vi "Run_old02.vi"(8 "error in (no error)":errorcluster, 11 "Channel in":refnum<class "Channel.lvclass">) -> (0 "error out":errorcluster, 3 "Channel out":refnum<class "Channel.lvclass">)   [LabVIEW 2018, in "Channel.lvclass"]
uses:
  Channel.lvclass
  C:/Users/devstaff/sparc4/s4gui/Versao ZeroMQ REQ-REP/SPARC4_GUI -20241009_20240802/Device/Device.lvclass
  Channel.lvclass/Channel.ctl
  Interface/Interface.lvclass/Interface.ctl
  Device/Device.lvclass/Device.ctl
  StateMachine/State Machine.lvclass
  Interface/Interface.lvclass
  Device/Device.lvclass
panel:
  out "resp RESUME":string
  out "resp PAUSE":string
  out "x = y?":T1
  out "resp ABORT":string
  out "resp STOP":string
  out "resposta do STATUS":string
  out "resp INIT":string
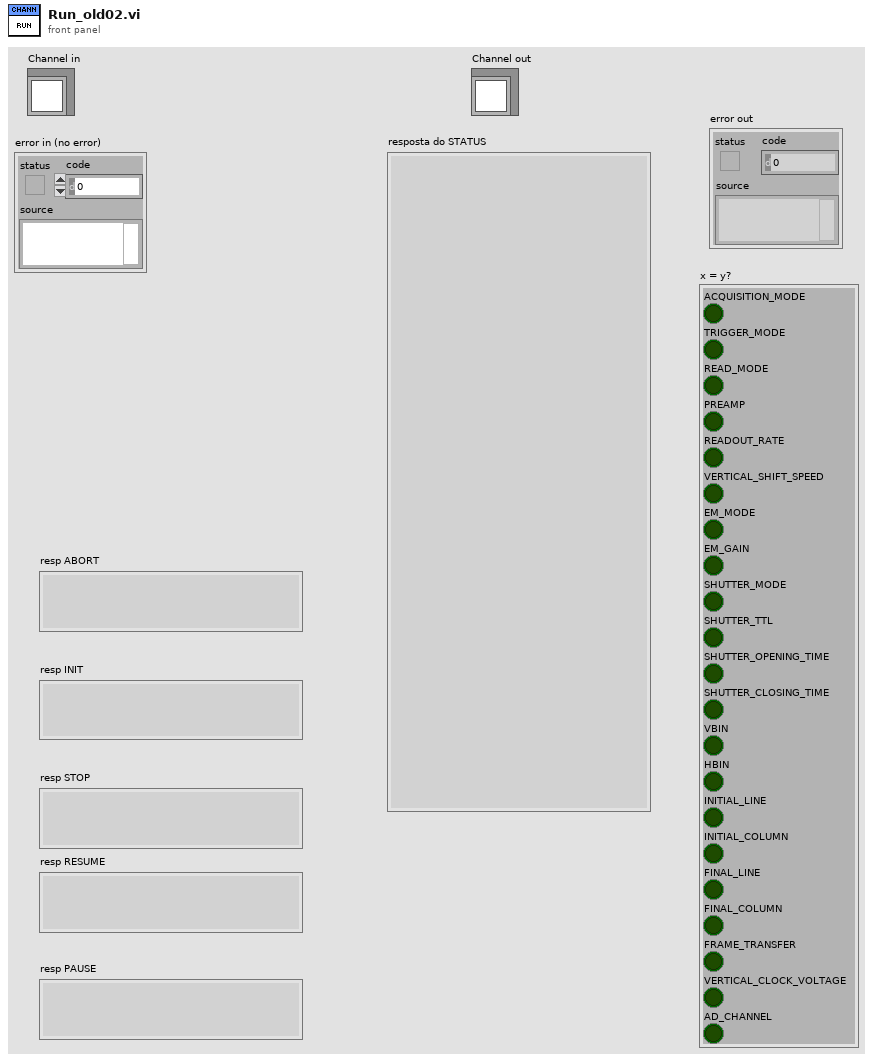
[diagram p1: front panel]
types:
  T1 = cluster{"ACQUISITION_MODE":bool, "TRIGGER_MODE":bool, "READ_MODE":bool, "PREAMP":bool, "READOUT_RATE":bool, "VERTICAL_SHIFT_SPEED":bool, "EM_MODE":bool, "EM_GAIN":bool, "SHUTTER_MODE":bool, "SHUTTER_TTL":bool, "SHUTTER_OPENING_TIME":bool, "SHUTTER_CLOSING_TIME":bool, "VBIN":bool, "HBIN":bool, "INITIAL_LINE":bool, "INITIAL_COLUMN":bool, "FINAL_LINE":bool, "FINAL_COLUMN":bool, "FRAME_TRANSFER":bool, "VERTICAL_CLOCK_VOLTAGE":bool, "AD_CHANNEL":bool}
  T2 = cluster{"TEMP":dbl, "EXPTIME":dbl, "#FRAMES":u32, "#CYCLES":u32, "#SEQS":u32, "WAVEPLATE_POS":u32, "COOLER_POWER_STATUS":dbl, "suffix":string}
  T3 = cluster{"ACQUISITION_MODE":u8, "TRIGGER_MODE":u8, "READ_MODE":u8, "PREAMP":u8, "READOUT_RATE":u8, "VERTICAL_SHIFT_SPEED":u8, "EM_MODE":u8, "EM_GAIN":u16, "SHUTTER_MODE":u8, "SHUTTER_TTL":u8, "SHUTTER_OPENING_TIME":u16, "SHUTTER_CLOSING_TIME":u16, "VBIN":u16, "HBIN":u16, "INITIAL_LINE":u16, "INITIAL_COLUMN":u16, "FINAL_LINE":u16, "FINAL_COLUMN":u16, "FRAME_TRANSFER":bool, "VERTICAL_CLOCK_VOLTAGE":u8, "AD_CHANNEL":u32}
  T4 = cluster{"Image Name":string, "Image Path":string, "#FRAMES":u32, "EXPTIME":dbl, "PREAMP":u8, "READOUT_RATE":u8, "VERTICAL_SHIFT_SPEED":u8, "ACQUISITION_MODE":u8, "READ_MODE":u8, "EM_MODE":u8, "EM_GAIN":u16, "SHUTTER_MODE":u8, "SHUTTER_TTL":u8, "SHUTTER_OPENNING_TIME":u16, "SHUTTER_CLOSING_TIME":u16, "VBIN":u16, "HBIN":u16, "INITIAL_LINE":u16, "INITIAL_COLUMN":u16, "FINAL_LINE":u16, "FINAL_COLUMN":u16, "Cooler ON/OFF":u16, "Set temperature":i8, "Exposições realizadas":u16, "Kinetic Serie Length":u32, "Number of Accumulations":u32, "Kinetic Cycle Time":u32, "FRAME_TRANSFER":bool, "VERTICAL_CLOCK_VOLTAGE":u8, "TRIGGER_MODE":u8, "Number of exp":u32, "AD_CHANNEL":u32}
  T5 = cluster{"OBSERVER":string, "OBJECT":string, "CTRLINTE":string, "PROJID":string, "SYNCMODE":string, "INSTMODE":string, "FILTER":string, "OBSTYPE":string, "CHANNEL 1":bool, "CHANNEL 2":bool, "CHANNEL 3":bool, "CHANNEL 4":bool, "TCSMODE":bool, "COMMENT":string, "broker":string, "GUIVRSN":string, "timestamp":string}
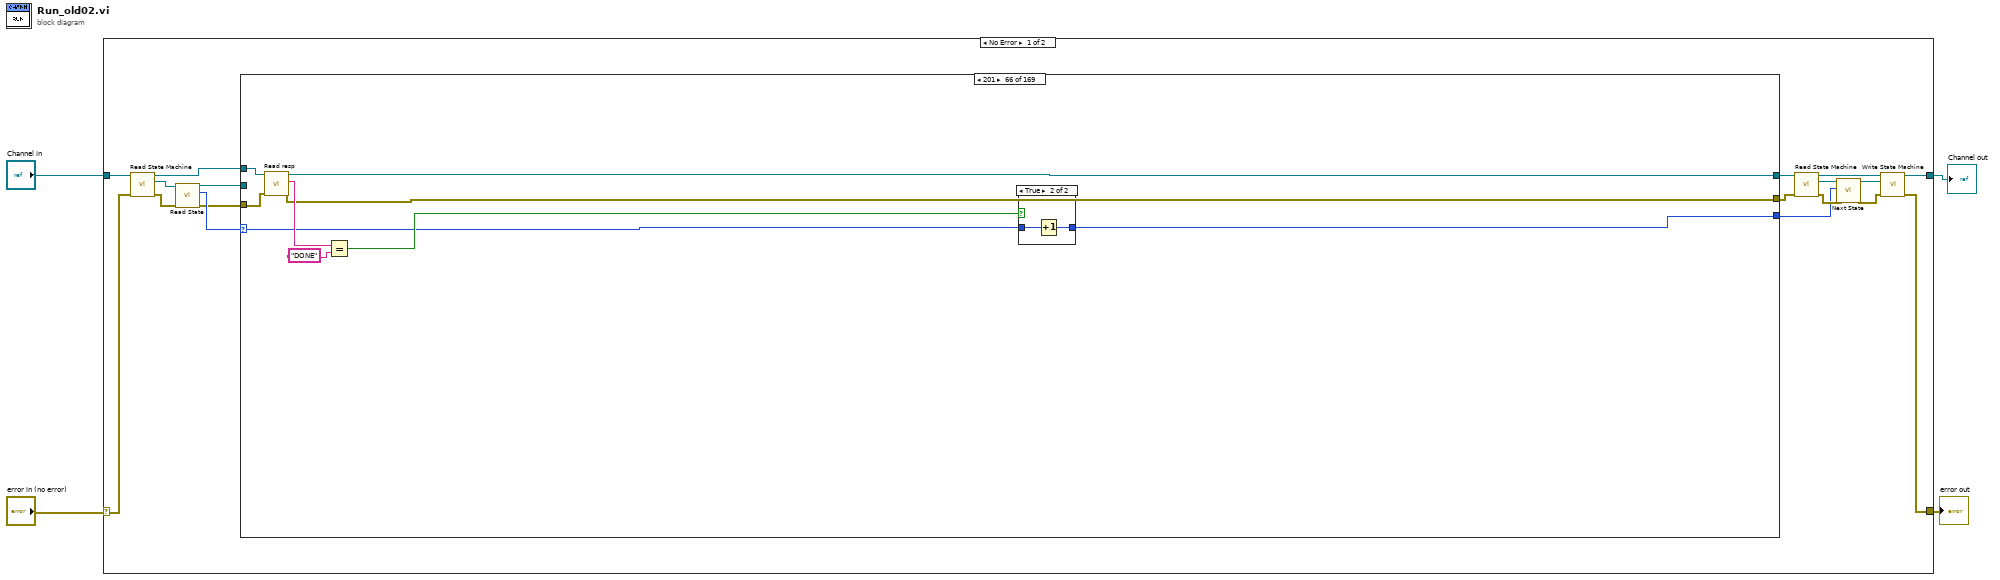
[diagram p0: block diagram]
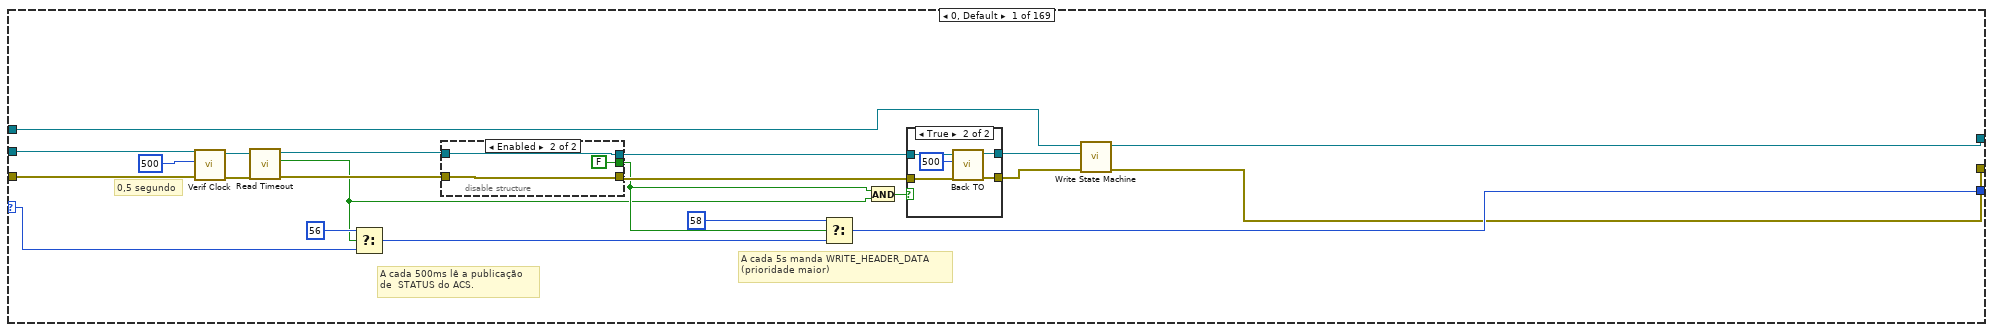
[diagram p2: hidden frame]
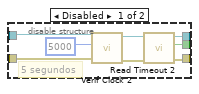
[diagram p3: hidden frame]
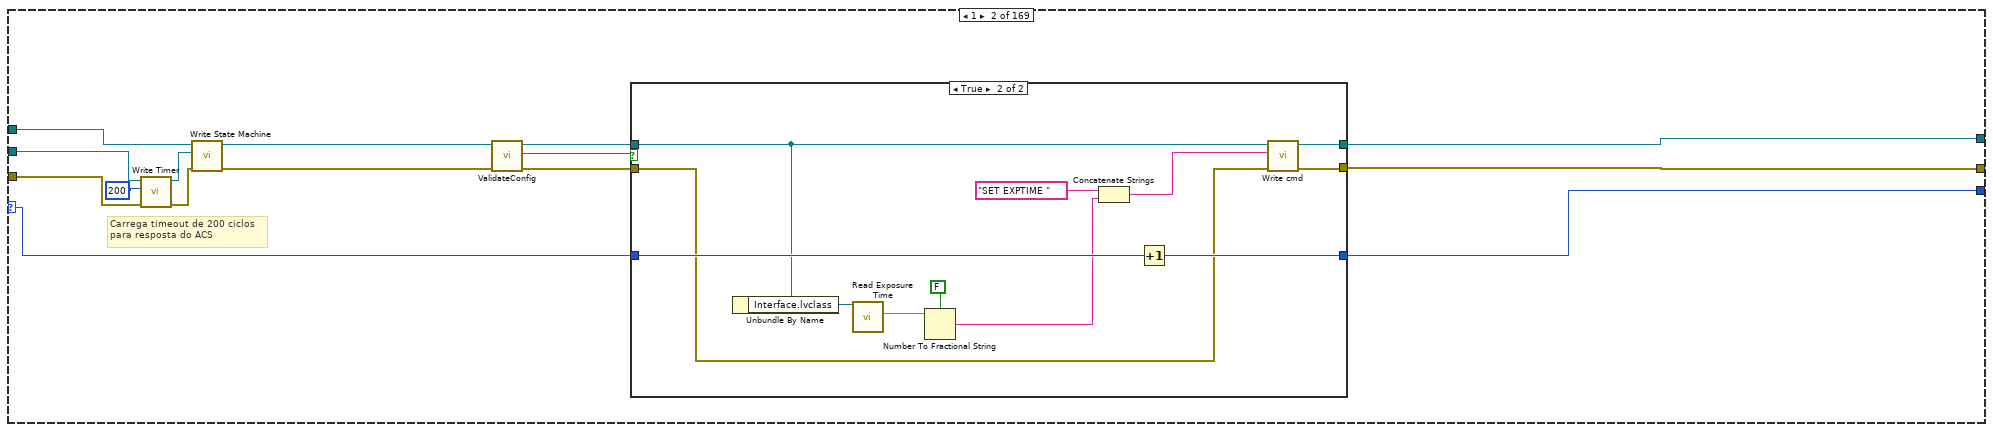
[diagram p5: hidden frame]
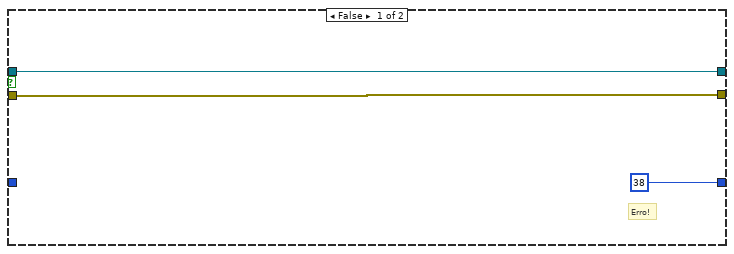
[diagram p6: hidden frame]
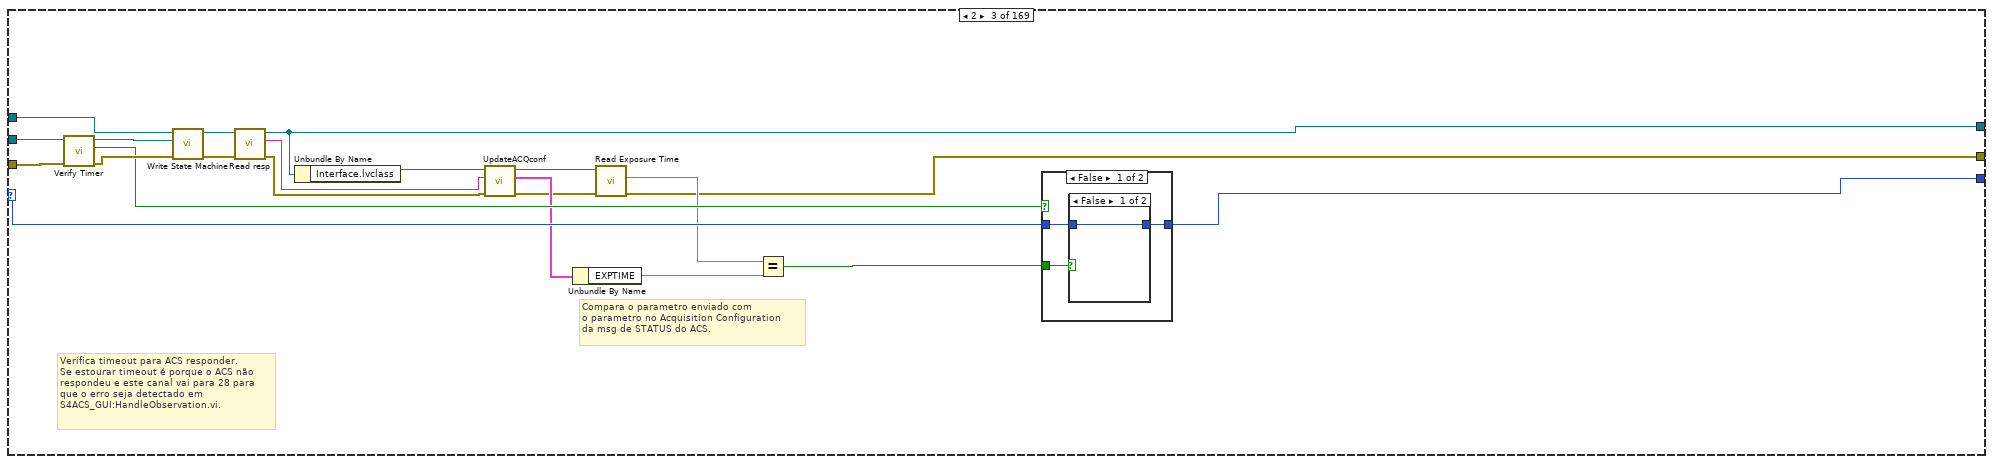
[diagram p7: hidden frame]
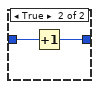
[diagram p8: hidden frame]
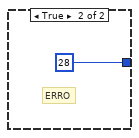
[diagram p9: hidden frame]
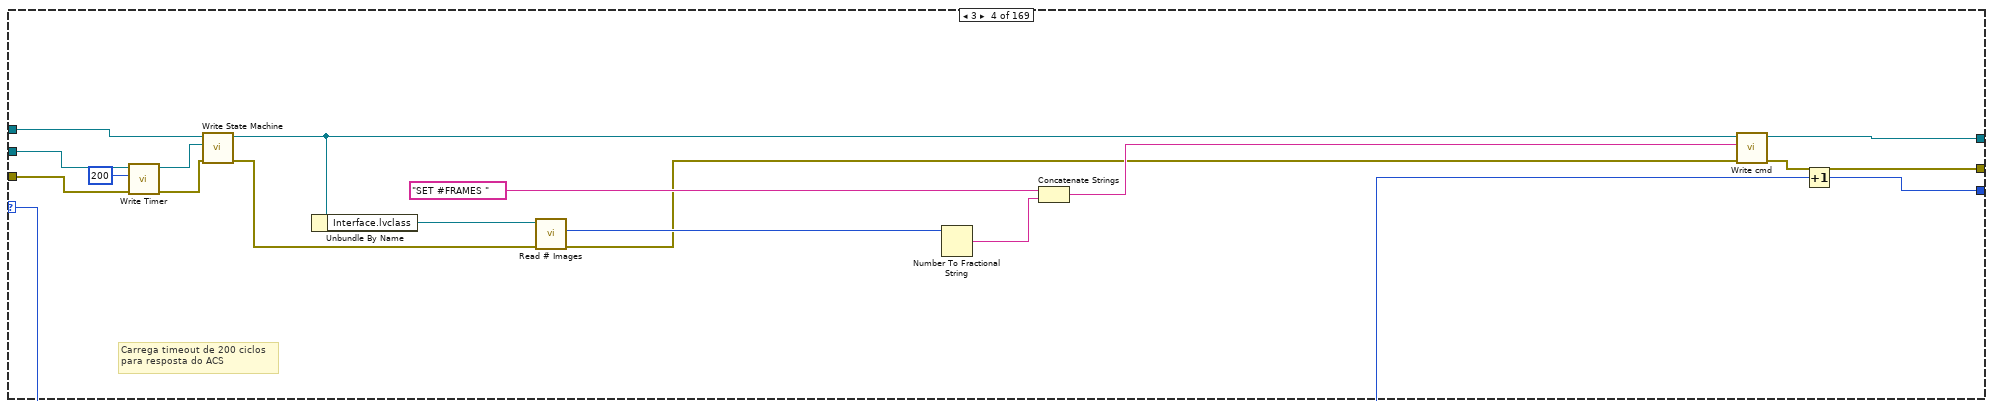
[diagram p10: hidden frame]
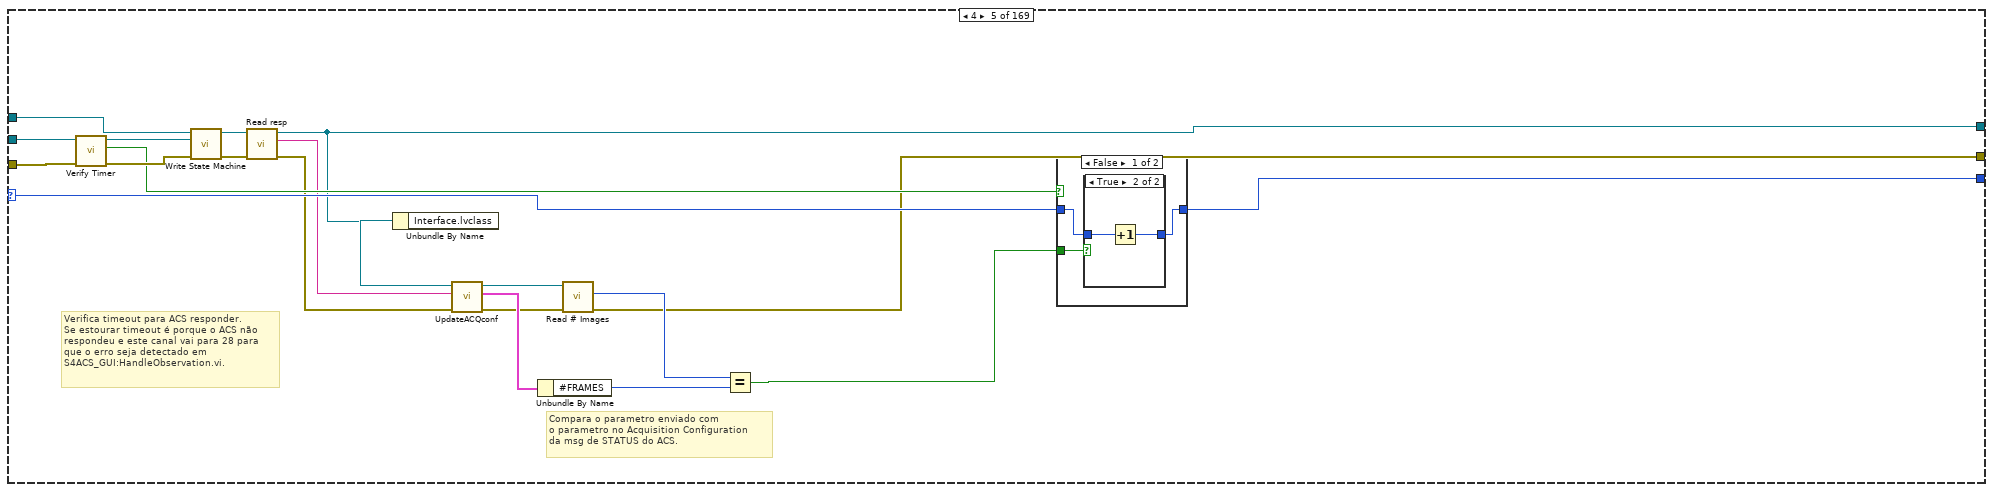
[diagram p11: hidden frame]
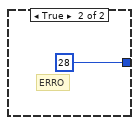
[diagram p13: hidden frame]
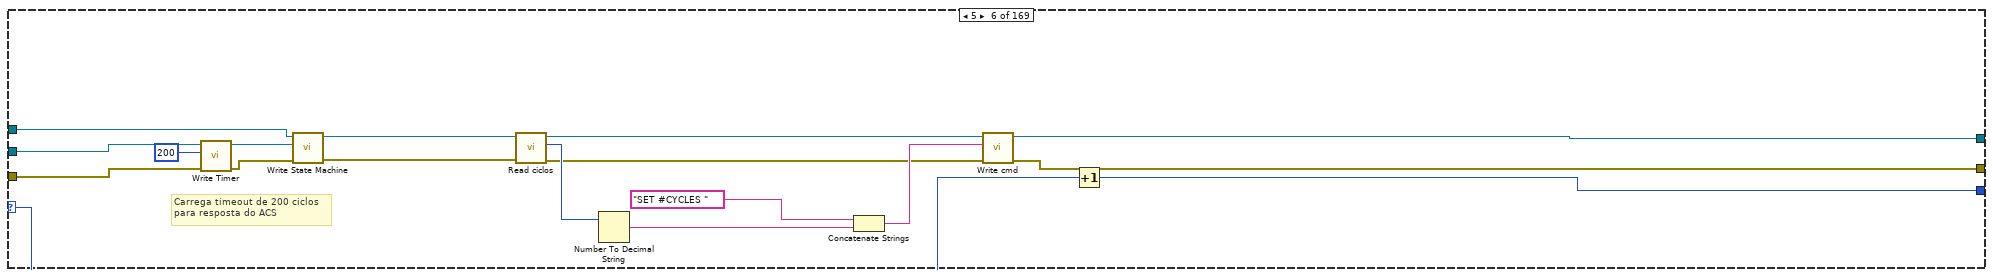
[diagram p14: hidden frame]
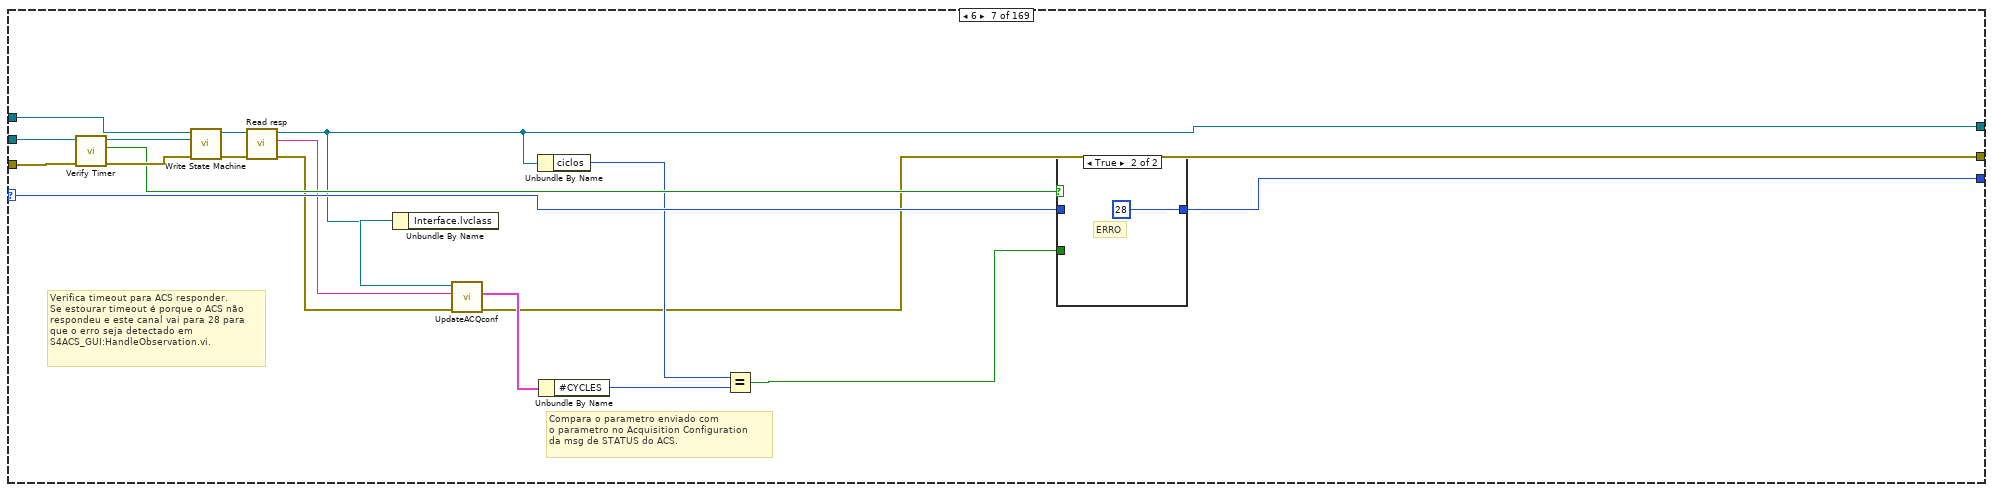
[diagram p15: hidden frame]
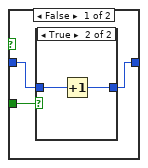
[diagram p16: hidden frame]
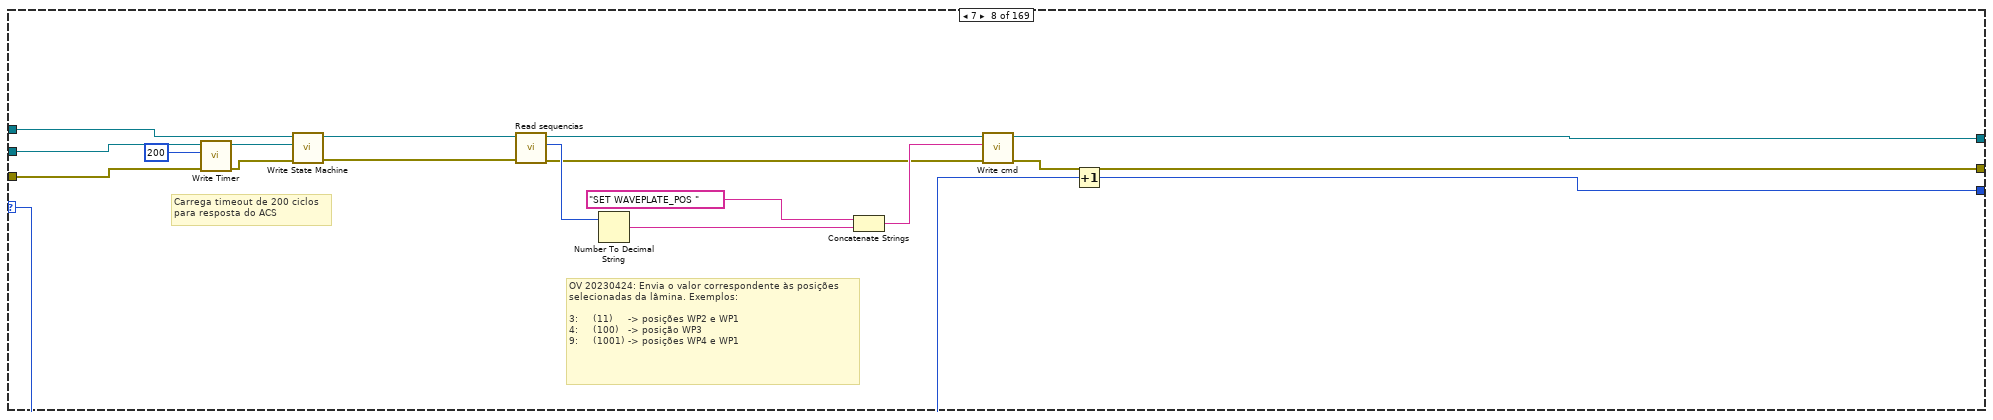
[diagram p18: hidden frame]
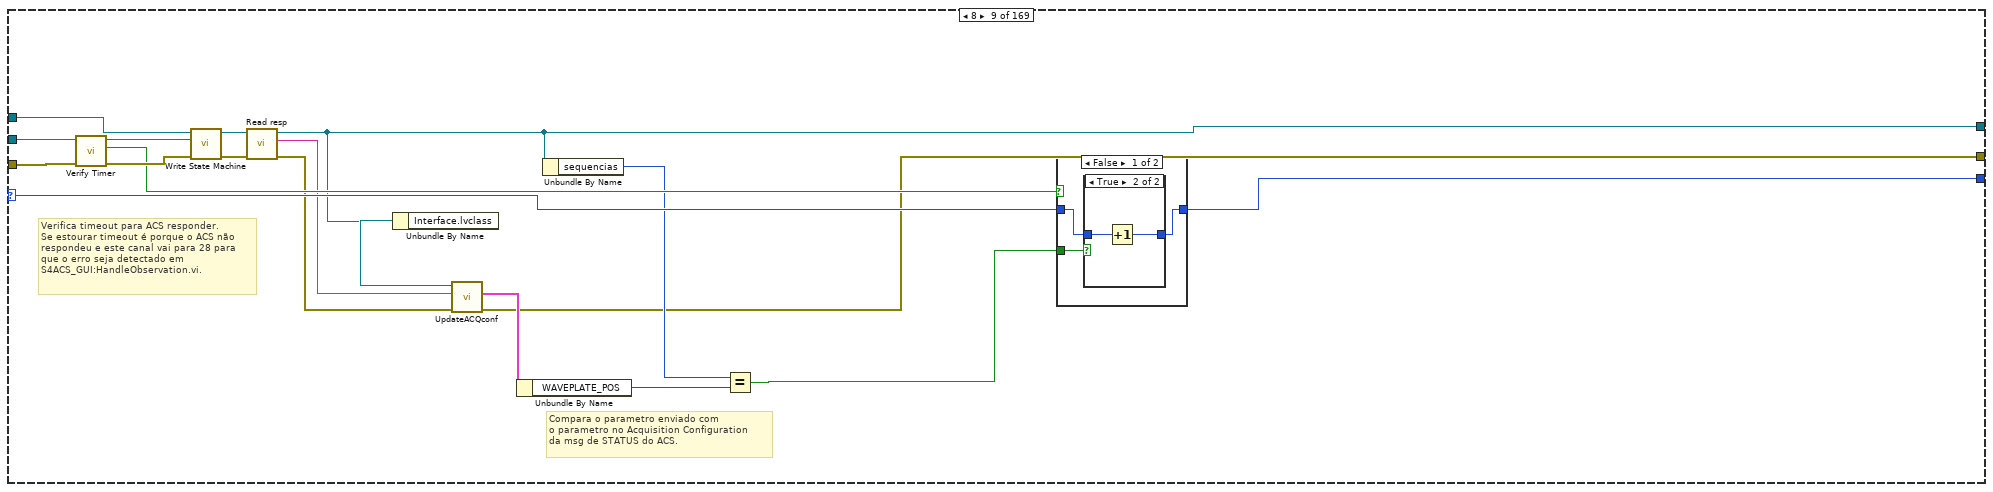
[diagram p19: hidden frame]
diagram:
  n1 = case shown="No Error" "error in (no error)" {
    selector: "error in (no error)" -> [w21 w2905]
    tunnel: [w6 w2905] -> w3
    tunnel: [w11 w2904] -> w1
    tunnel: "Channel in" -> [w22 w2904]
    frame No Error {
      n2 = call-dynamic "Read State Machine.vi"("error in (no error)"=w21, "Device in"=w22) -> ("error out"=w18:errorcluster, "State Machine.lvclass"=w20:refnum<class "State Machine.lvclass">, "Device out"=w16:refnum<class "Channel.lvclass">)  [unwired: 7 in]
      n3 = call-dynamic "Read State.vi"("error in (no error)"=w18, "State Machine in"=w20) -> ("error out"=w17:errorcluster, "State"=w19:i32, "State Machine out"=w5:refnum<class "State Machine.lvclass">)  [unwired: 7 in]
      n4 = case shown="201" w19 {
        selector: w19 -> [w40 w74 w106 w123 w151 w175 w195 w219 w239 w263 w292 w306 w318 w348 w362 w387 w390 w396 w412 w440 w459 w472 w516 w545 _ w568 _ w605 w634 w645 w706 w726 w804 w863 w931 _ _ w1036 w1068 w1089 w1127 w1140 w1156 w1219 w1253 w1286 w1292 w1306 w1314 w1329 _ w1354 _ w1373 w1384 w1404 w1424 w1444 w1464 w1484 w1504 w1524 w1544 _ w1564 w1572 w1585 w1598 w1614 w1622 w1635 w1649 w1661 w1669 w1682 w1695 w1707 w1715 w1728 w1741 w1753 w1761 w1774 w1787 w1799 w1807 w1820 w1833 w1845 w1853 w1866 w1879 w1891 w1899 w1912 w1925 w1937 w1945 w1958 w1971 w1987 w1995 w2008 w2021 w2033 w2041 w2054 w2067 w2079 w2087 w2100 w2113 w2125 w2133 w2146 w2159 w2171 w2179 w2192 w2205 w2217 w2225 w2238 w2251 w2263 w2271 w2284 w2297 w2309 w2317 w2330 w2343 w2355 w2363 w2376 w2389 w2401 w2409 w2422 w2435 w2447 w2455 w2468 w2481 w2497 w2505 w2518 w2531 w2543 w2553 w2566 w2579 w2593 w2601 w2614 w2627 w2645 w2678 w2699 w2721 w2734 w2763 w2769 w2795 w2807 w2832 w2844 w2869 w2881]
        tunnel: w17 -> [w38 w73 w110 w125 w154 w177 w198 w221 w242 w260 w291 w308 w320 w350 w364 w389 w392 w394 w404 w439 w454 w466 w514 w544 w561 w570 w582 w602 w627 w643 w667 w723 w768 w856 w905 w965 w1004 w1044 w1056 w1085 w1122 w1134 w1170 w1216 w1248 w1279 w1296 w1309 w1318 w1331 w1345 w1356 w1370 w1377 w1388 w1399 w1419 w1439 w1459 w1479 w1499 w1519 w1539 w1557 w1570 w1579 w1589 w1601 w1620 w1629 w1639 w1652 w1667 w1676 w1686 w1698 w1713 w1722 w1732 w1744 w1759 w1768 w1778 w1790 w1805 w1814 w1824 w1836 w1851 w1860 w1870 w1882 w1897 w1906 w1916 w1928 w1943 w1952 w1962 w1974 w1993 w2002 w2012 w2024 w2039 w2048 w2058 w2070 w2085 w2094 w2104 w2116 w2131 w2140 w2150 w2162 w2177 w2186 w2196 w2208 w2223 w2232 w2242 w2254 w2269 w2278 w2288 w2300 w2315 w2324 w2334 w2346 w2361 w2370 w2380 w2392 w2407 w2416 w2426 w2438 w2453 w2462 w2472 w2484 w2503 w2512 w2522 w2534 w2549 w2560 w2570 w2582 w2599 w2608 w2618 w2630 w2637 w2682 w2706 w2715 w2740 w2757 w2775 w2797 w2809 w2834 w2846 w2871 w2883]
        tunnel: [w23 w76 w93 w137 w139 w183 w185 w227 w229 w271 w274 w314 w327 w356 w371 w389 w392 w394 w416 w420 w461 w474 w524 w527 w566 w570 w586 w597 w621 w647 w698 w711 w779 w851 w906 w977 w1015 w1043 w1069 w1090 w1119 w1142 w1157 w1221 w1235 w1267 w1293 w1302 w1315 w1326 w1343 w1351 w1365 w1376 w1385 w1399 w1419 w1439 w1459 w1479 w1499 w1519 w1539 w1557 w1569 w1573 w1588 w1599 w1619 w1623 w1638 w1650 w1666 w1670 w1685 w1696 w1712 w1716 w1731 w1742 w1758 w1762 w1777 w1788 w1804 w1808 w1823 w1834 w1850 w1854 w1869 w1880 w1896 w1900 w1915 w1926 w1942 w1946 w1961 w1972 w1992 w1996 w2011 w2022 w2038 w2042 w2057 w2068 w2084 w2088 w2103 w2114 w2130 w2134 w2149 w2160 w2176 w2180 w2195 w2206 w2222 w2226 w2241 w2252 w2268 w2272 w2287 w2298 w2314 w2318 w2333 w2344 w2360 w2364 w2379 w2390 w2406 w2410 w2425 w2436 w2452 w2456 w2471 w2482 w2502 w2506 w2521 w2532 w2548 w2554 w2569 w2580 w2598 w2602 w2617 w2628 w2649 w2664 w2702 w2724 w2743 w2765 w2778 w2803 w2816 w2840 w2853 w2877 w2890] -> w7
        tunnel: w16 -> [w31 w71 w113 w126 w158 w178 w202 w222 w246 w259 w290 w309 w324 w351 w368 w388 w391 w393 w407 w438 w456 w469 w513 w543 w564 w569 w583 w596 w633 w644 w680 w719 w778 w858 w899 w976 w1014 w1038 w1060 w1083 w1123 w1135 w1171 w1215 w1251 w1280 w1297 w1308 w1319 w1323 w1346 w1348 w1371 w1375 w1389 w1397 w1417 w1437 w1457 w1477 w1497 w1517 w1537 w1559 w1568 w1580 w1587 w1602 w1618 w1630 w1637 w1653 w1665 w1677 w1684 w1699 w1711 w1723 w1730 w1745 w1757 w1769 w1776 w1791 w1803 w1815 w1822 w1837 w1849 w1861 w1868 w1883 w1895 w1907 w1914 w1929 w1941 w1953 w1960 w1975 w1991 w2003 w2010 w2025 w2037 w2049 w2056 w2071 w2083 w2095 w2102 w2117 w2129 w2141 w2148 w2163 w2175 w2187 w2194 w2209 w2221 w2233 w2240 w2255 w2267 w2279 w2286 w2301 w2313 w2325 w2332 w2347 w2359 w2371 w2378 w2393 w2405 w2417 w2424 w2439 w2451 w2463 w2470 w2485 w2501 w2513 w2520 w2535 w2547 w2561 w2568 w2583 w2597 w2609 w2616 w2631 w2639 w2685 w2705 w2717 w2741 w2759 w2776 w2798 w2813 w2835 w2850 w2872 w2887]
        tunnel: [w30 w77 w102 w138 w142 w184 w187 w228 w231 w264 w276 w315 w328 w357 w372 w388 w391 w393 w417 w421 w462 w477 w517 w529 w567 w569 w571 w598 w622 w648 w705 w712 w803 w852 w930 w978 w1016 w1045 w1070 w1091 w1120 w1143 w1167 w1222 w1233 w1273 w1294 w1301 w1316 w1325 w1344 w1350 w1369 w1378 w1381 w1401 w1421 w1441 w1461 w1481 w1501 w1521 w1541 w1559 w1571 w1574 w1590 w1597 w1621 w1624 w1640 w1648 w1668 w1671 w1687 w1694 w1714 w1717 w1733 w1740 w1760 w1763 w1779 w1786 w1806 w1809 w1825 w1832 w1852 w1855 w1871 w1878 w1898 w1901 w1917 w1924 w1944 w1947 w1963 w1970 w1994 w1997 w2013 w2020 w2040 w2043 w2059 w2066 w2086 w2089 w2105 w2112 w2132 w2135 w2151 w2158 w2178 w2181 w2197 w2204 w2224 w2227 w2243 w2250 w2270 w2273 w2289 w2296 w2316 w2319 w2335 w2342 w2362 w2365 w2381 w2388 w2408 w2411 w2427 w2434 w2454 w2457 w2473 w2480 w2504 w2507 w2523 w2530 w2550 w2555 w2571 w2578 w2600 w2603 w2619 w2626 w2650 w2675 w2701 w2725 w2744 w2766 w2779 w2804 w2817 w2841 w2854 w2878 w2891] -> w14
        tunnel: [w37 w75 w105 w132 w150 w182 w194 w226 w238 w265 w293 w313 w319 w355 w360 w387 w390 w397 w413 w441 w460 w473 w518 w546 31 ("State") w568 0 ("State") w603 w635 w646 w707 w727 w805 w864 w932 0 ("State") 54 ("State") w1035 w1071 w1088 w1128 w1141 w1155 w1220 w1254 w1287 w1295 w1307 w1317 w1330 0 ("State") w1355 0 ("State") w1374 w1386 w1396 w1416 w1436 w1456 w1476 w1496 w1516 w1536 u8 0 ("State") w1565 w1575 w1586 w1600 w1615 w1625 w1636 w1651 w1662 w1672 w1683 w1697 w1708 w1718 w1729 w1743 w1754 w1764 w1775 w1789 w1800 w1810 w1821 w1835 w1846 w1856 w1867 w1881 w1892 w1902 w1913 w1927 w1938 w1948 w1959 w1973 w1988 w1998 w2009 w2023 w2034 w2044 w2055 w2069 w2080 w2090 w2101 w2115 w2126 w2136 w2147 w2161 w2172 w2182 w2193 w2207 w2218 w2228 w2239 w2253 w2264 w2274 w2285 w2299 w2310 w2320 w2331 w2345 w2356 w2366 w2377 w2391 w2402 w2412 w2423 w2437 w2448 w2458 w2469 w2483 w2498 w2508 w2519 w2533 w2544 w2556 w2567 w2581 w2594 w2604 w2615 w2629 w2646 w2677 w2700 w2722 w2732 w2764 w2767 w2802 w2808 w2839 w2845 w2876 w2879] -> w8
        tunnel: w5 -> [w39 w72 w112 w127 w159 w176 w203 w220 w247 w261 w288 w307 w321 w349 w365 _ _ _ w406 w436 w455 w470 w512 w541 w563 _ w584 w601 w631 _ w670 w724 w771 w860 w904 w966 w1005 w1040 w1061 w1086 w1124 w1137 w1172 w1217 w1252 w1281 _ _ _ _ _ _ _ _ _ _ _ _ _ _ _ _ _ _ _ _ _ _ _ _ _ _ _ _ _ _ _ _ _ _ _ _ _ _ _ _ _ _ _ _ _ _ _ _ _ _ _ _ _ _ _ _ _ _ _ _ _ _ _ _ _ _ _ _ _ _ _ _ _ _ _ _ _ _ _ _ _ _ _ _ _ _ _ _ _ _ _ _ _ _ _ _ _ _ _ _ _ _ _ _ _ _ _ _ _ _ w2641 w2684 w2707 w2713 w2738 w2756 w2773 w2796 w2810 w2833 w2847 w2870 w2884]
        frame 0, Default {
          # "A cada 5s manda WRITE_HEADER_DATA\n(prioridade maior)"
          # "A cada 500ms lê a publicação \nde  STATUS do ACS."
          # "0,5 segundo"
          n5 = call-dynamic "Verif Clock.vi"("error in (no error)"=w38, "period (ms)"=u32 500 ("period"), "State Machine in"=w39) -> ("error out"=w43:errorcluster, "State Machine out"=w42:refnum<class "State Machine.lvclass">)  [unwired: 6 in, 1 out]
          n6 = call-dynamic "Read Timeout.vi"("error in (no error)"=w43, "State Machine in"=w42) -> ("error out"=w33:errorcluster, "Timeout"=w24:bool, "State Machine out"=w34:refnum<class "State Machine.lvclass">)  [unwired: 7 in]
          n7 = Select(t=56 ("State"), s=w24, f=w40) -> (s? t:f=w35:i32)
          n8 = disable-structure shown="Enabled" {
            disable-tunnel: w34 -> [w52 w54]
            disable-tunnel: w33 -> [w50 w53]
            disable-tunnel: [w47 w53] -> w32
            disable-tunnel: [w46 w54] -> w28
            disable-tunnel: [w45 FALSE ("Timeout 2")] -> w25
            frame Disabled {
              # "5 segundos"
              n9 = call-dynamic "Verif Clock 2.vi"("error in (no error)"=w50, "period (ms)"=u32 5000 ("period"), "State Machine in"=w52) -> ("error out"=w49:errorcluster, "State Machine out"=w51:refnum<class "State Machine.lvclass">)  [unwired: 6 in, 1 out]
              n10 = call-dynamic "Read Timeout 2.vi"("error in (no error)"=w49, "State Machine in"=w51) -> ("error out"=w47:errorcluster, "Timeout 2"=w45:bool, "State Machine out"=w46:refnum<class "State Machine.lvclass">)  [unwired: 7 in]
            }
            frame Enabled {
            }
          }
          n11 = Select(t=58 ("f"), s=w25, f=w35) -> (s? t:f=w37:i32)
          n12 = And(x=w25, y=w24) -> (x .and. y?=w26:bool)
          n13 = case shown="True" w26 {
            tunnel: w32 -> [w56 w62]
            tunnel: [w56 w61] -> w29
            tunnel: w28 -> [w57 w60]
            tunnel: [w57 w59] -> w27
            frame False {
            }
            frame True {
              n14 = call-dynamic "Back TO.vi"("error in (no error)"=w62, "time back (ms)"=u32 500 ("time(ms)"), "State Machine in"=w60) -> ("error out"=w61:errorcluster, "State Machine out"=w59:refnum<class "State Machine.lvclass">)  [unwired: 7 in]
            }
          }
          n15 = call-dynamic "Write State Machine.vi"("error in (no error)"=w29, "State Machine.lvclass"=w27, "Device in"=w31) -> ("error out"=w23:errorcluster, "Device out"=w30:refnum<class "Channel.lvclass">)  [unwired: 7 in]
        }
        frame 1 {
          # "Carrega timeout de 200 ciclos\npara resposta do ACS"
          n16 = call-dynamic "Write Timer.vi"("error in (no error)"=w73, "Timer"=u32 200, "State Machine in"=w72) -> ("error out"=w68:errorcluster, "State Machine out"=w70:refnum<class "State Machine.lvclass">)  [unwired: 7 in]
          n17 = call-dynamic "Write State Machine.vi"("error in (no error)"=w68, "State Machine.lvclass"=w70, "Device in"=w71) -> ("error out"=w66:errorcluster, "Device out"=w67:refnum<class "Channel.lvclass">)  [unwired: 7 in]
          n18 = call-dynamic "ValidateConfig.vi"("error in (no error)"=w66, "Channel in"=w67) -> ("error out"=w64:errorcluster, "valid?"=w63:bool, "Channel out"=w65:refnum<class "Channel.lvclass">)  [unwired: 7 in]
          n19 = case shown="True" w63 {
            tunnel: [w80 w92] -> w77
            tunnel: [w79 w91] -> w76
            tunnel: [38 w90] -> w75
            tunnel: w74 -> [_ w89]
            tunnel: w65 -> [w80 w82]
            tunnel: w64 -> [w79 w81]
            frame False {
              # "Erro!"
            }
            frame True {
              n20 = Unbundle By Name(w82) -> ("Interface.lvclass"=w88:refnum<class "Interface.lvclass">)
              n21 = call "Read Exposure Time.vi"("Interface in"=w88) -> ("Exposure Time"=w87:dbl)  [unwired: 8 in, 2 out]
              n22 = Number To Fractional String(use system decimal point (T)=FALSE, number=w87) -> (F-format string=w86:string)  [unwired: 2 in]
              n23 = Concatenate Strings("SET EXPTIME " ("cmd"), w86) -> (w85:string)
              n24 = Increment(x=w89) -> (x+1=w90:i32)
              n25 = call-dynamic "Write cmd.vi"("error in (no error)"=w81, "cmd"=w85, "Device in"=w82) -> ("error out"=w91:errorcluster, "Device out"=w92:refnum<class "Channel.lvclass">)  [unwired: 7 in]
            }
          }
        }
        frame 2 {
          # "Compara o parametro enviado com\no parametro no Acquisition Configuration\nda msg de STATUS do ACS."
          # "Verifica timeout para ACS responder.\nSe estourar timeout é porque o ACS não \nrespondeu e este canal vai para 28 para \nque o erro seja detectado em\nS4ACS_GUI:HandleObservation.vi."
          n26 = call "Verify Timer.vi"("error in (no error)"=w110, "State Machine in"=w112) -> ("error out"=w109:errorcluster, "timeout"=w107:bool, "State Machine out"=w111:refnum<class "State Machine.lvclass">)  [unwired: 7 in]
          n27 = call-dynamic "Write State Machine.vi"("error in (no error)"=w109, "State Machine.lvclass"=w111, "Device in"=w113) -> ("error out"=w108:errorcluster, "Device out"=w104:refnum<class "Channel.lvclass">)  [unwired: 7 in]
          n28 = call-dynamic "Read resp.vi"("error in (no error)"=w108, "Device in"=w104) -> ("error out"=w95:errorcluster, "resp"=w103:string, "Device out"=w102:refnum<class "Channel.lvclass">)  [unwired: 7 in]
          n29 = Unbundle By Name(w102) -> ("Interface.lvclass"=w101:refnum<class "Interface.lvclass">)
          n30 = call-dynamic "UpdateACQconf.vi"("error in (no error)"=w95, "status"=w103, "Interface in"=w101) -> ("error out"=w94:errorcluster, "ACQ conf rx"=w99:T2, "Interface out"=w100:refnum<class "Interface.lvclass">)  [unwired: 6 in]
          n31 = Unbundle By Name(w99) -> ("EXPTIME"=w97:dbl)
          n32 = call "Read Exposure Time.vi"("error in (no error)"=w94, "Interface in"=w100) -> ("error out"=w93:errorcluster, "Exposure Time"=w98:dbl)  [unwired: 7 in, 1 out]
          n33 = Equal?(x=w98, y=w97) -> (x = y?=w96:bool)
          n34 = case shown="False" w107 {
            tunnel: [w115 28] -> w105
            tunnel: w106 -> [w116 _]
            tunnel: w96 -> [w114 _]
            frame False {
              n35 = case shown="False" w114 {
                tunnel: [w117 w118] -> w115
                tunnel: w116 -> [w117 w119]
                frame False {
                }
                frame True {
                  n36 = Increment(x=w119) -> (x+1=w118:i32)
                }
              }
            }
            frame True {
              # "ERRO"
            }
          }
        }
        frame 3 {
          # "Carrega timeout de 200 ciclos\npara resposta do ACS"
          n37 = call-dynamic "Write Timer.vi"("error in (no error)"=w125, "Timer"=u32 200, "State Machine in"=w127) -> ("error out"=w128:errorcluster, "State Machine out"=w130:refnum<class "State Machine.lvclass">)  [unwired: 7 in]
          n38 = call-dynamic "Write State Machine.vi"("error in (no error)"=w128, "State Machine.lvclass"=w130, "Device in"=w126) -> ("error out"=w122:errorcluster, "Device out"=w124:refnum<class "Channel.lvclass">)  [unwired: 7 in]
          n39 = Unbundle By Name(w124) -> ("Interface.lvclass"=w136:refnum<class "Interface.lvclass">)
          n40 = call-dynamic "Read # Images.vi"("error in (no error)"=w122, "Interface in"=w136) -> ("error out"=w121:errorcluster, "# Images"=w135:u32)  [unwired: 7 in, 1 out]
          n41 = Number To Fractional String(number=w135) -> (F-format string=w134:string)  [unwired: 3 in]
          n42 = Concatenate Strings("SET #FRAMES " ("cmd"), w134) -> (w133:string)
          n43 = call-dynamic "Write cmd.vi"("error in (no error)"=w121, "cmd"=w133, "Device in"=w124) -> ("error out"=w137:errorcluster, "Device out"=w138:refnum<class "Channel.lvclass">)  [unwired: 7 in]
          n44 = Increment(x=w123) -> (x+1=w132:i32)
        }
        frame 4 {
          # "Verifica timeout para ACS responder.\nSe estourar timeout é porque o ACS não \nrespondeu e este canal vai para 28 para \nque o erro seja detectado em\nS4ACS_GUI:HandleObservation.vi."
          # "Compara o parametro enviado com\no parametro no Acquisition Configuration\nda msg de STATUS do ACS."
          n45 = call "Verify Timer.vi"("error in (no error)"=w154, "State Machine in"=w159) -> ("error out"=w153:errorcluster, "timeout"=w152:bool, "State Machine out"=w155:refnum<class "State Machine.lvclass">)  [unwired: 7 in]
          n46 = call-dynamic "Write State Machine.vi"("error in (no error)"=w153, "State Machine.lvclass"=w155, "Device in"=w158) -> ("error out"=w156:errorcluster, "Device out"=w157:refnum<class "Channel.lvclass">)  [unwired: 7 in]
          n47 = call-dynamic "Read resp.vi"("error in (no error)"=w156, "Device in"=w157) -> ("error out"=w140:errorcluster, "resp"=w141:string, "Device out"=w142:refnum<class "Channel.lvclass">)  [unwired: 7 in]
          n48 = Unbundle By Name(w142) -> ("Interface.lvclass"=w149:refnum<class "Interface.lvclass">)
          n49 = call-dynamic "UpdateACQconf.vi"("error in (no error)"=w140, "status"=w141, "Interface in"=w149) -> ("error out"=w144:errorcluster, "ACQ conf rx"=w147:T2, "Interface out"=w148:refnum<class "Interface.lvclass">)  [unwired: 6 in]
          n50 = Unbundle By Name(w147) -> ("#FRAMES"=w145:u32)
          n51 = call-dynamic "Read # Images.vi"("error in (no error)"=w144, "Interface in"=w148) -> ("error out"=w139:errorcluster, "# Images"=w146:u32)  [unwired: 7 in, 1 out]
          n52 = Equal?(x=w146, y=w145) -> (x = y?=w143:bool)
          n53 = case shown="False" w152 {
            tunnel: [w161 28] -> w150
            tunnel: w151 -> [w162 _]
            tunnel: w143 -> [w160 _]
            frame False {
              n54 = case shown="True" w160 {
                tunnel: [w163 w164] -> w161
                tunnel: w162 -> [w163 w165]
                frame False {
                }
                frame True {
                  n55 = Increment(x=w165) -> (x+1=w164:i32)
                }
              }
            }
            frame True {
              # "ERRO"
            }
          }
        }
        frame 5 {
          # "Carrega timeout de 200 ciclos\npara resposta do ACS"
          n56 = call-dynamic "Write Timer.vi"("error in (no error)"=w177, "Timer"=u32 200, "State Machine in"=w176) -> ("error out"=w179:errorcluster, "State Machine out"=w181:refnum<class "State Machine.lvclass">)  [unwired: 7 in]
          n57 = call-dynamic "Write State Machine.vi"("error in (no error)"=w179, "State Machine.lvclass"=w181, "Device in"=w178) -> ("error out"=w173:errorcluster, "Device out"=w174:refnum<class "Channel.lvclass">)  [unwired: 7 in]
          n58 = call-dynamic "Read ciclos.vi"("error in (no error)"=w173, "Channel in"=w174) -> ("error out"=w167:errorcluster, "ciclos"=w171:u32, "Channel out"=w172:refnum<class "Channel.lvclass">)  [unwired: 7 in]
          n59 = Number To Decimal String(number=w171) -> (decimal integer string=w169:string)  [unwired: 1 in]
          n60 = Concatenate Strings("SET #CYCLES " ("cmd"), w169) -> (w168:string)
          n61 = call-dynamic "Write cmd.vi"("error in (no error)"=w167, "cmd"=w168, "Device in"=w172) -> ("error out"=w183:errorcluster, "Device out"=w184:refnum<class "Channel.lvclass">)  [unwired: 7 in]
          n62 = Increment(x=w175) -> (x+1=w182:i32)
        }
        frame 6 {
          # "Verifica timeout para ACS responder.\nSe estourar timeout é porque o ACS não \nrespondeu e este canal vai para 28 para \nque o erro seja detectado em\nS4ACS_GUI:HandleObservation.vi."
          # "Compara o parametro enviado com\no parametro no Acquisition Configuration\nda msg de STATUS do ACS."
          n63 = call "Verify Timer.vi"("error in (no error)"=w198, "State Machine in"=w203) -> ("error out"=w197:errorcluster, "timeout"=w196:bool, "State Machine out"=w199:refnum<class "State Machine.lvclass">)  [unwired: 7 in]
          n64 = call-dynamic "Write State Machine.vi"("error in (no error)"=w197, "State Machine.lvclass"=w199, "Device in"=w202) -> ("error out"=w200:errorcluster, "Device out"=w201:refnum<class "Channel.lvclass">)  [unwired: 7 in]
          n65 = call-dynamic "Read resp.vi"("error in (no error)"=w200, "Device in"=w201) -> ("error out"=w188:errorcluster, "resp"=w189:string, "Device out"=w187:refnum<class "Channel.lvclass">)  [unwired: 7 in]
          n66 = Unbundle By Name(w187) -> ("Interface.lvclass"=w193:refnum<class "Interface.lvclass">)
          n67 = call-dynamic "UpdateACQconf.vi"("error in (no error)"=w188, "status"=w189, "Interface in"=w193) -> ("error out"=w185:errorcluster, "ACQ conf rx"=w192:T2)  [unwired: 6 in, 1 out]
          n68 = Unbundle By Name(w187) -> ("ciclos"=w186:u32)
          n69 = Unbundle By Name(w192) -> ("#CYCLES"=w191:u32)
          n70 = Equal?(x=w186, y=w191) -> (x = y?=w190:bool)
          n71 = case shown="True" w196 {
            tunnel: [w205 28] -> w194
            tunnel: w195 -> [w206 _]
            tunnel: w190 -> [w204 _]
            frame False {
              n72 = case shown="True" w204 {
                tunnel: [w207 w208] -> w205
                tunnel: w206 -> [w207 w209]
                frame False {
                }
                frame True {
                  n73 = Increment(x=w209) -> (x+1=w208:i32)
                }
              }
            }
            frame True {
              # "ERRO"
            }
          }
        }
        frame 7 {
          # "OV 20230424: Envia o valor correspondente às posições\nselecionadas da lâmina. Exemplos:\n\n3:     (11)     -> posições WP2 e WP1\n4:     (100)   -> posição WP3\n9:     (1001) -> posições WP4 e WP1"
          # "Carrega timeout de 200 ciclos\npara resposta do ACS"
          n74 = call-dynamic "Write Timer.vi"("error in (no error)"=w221, "Timer"=u32 200, "State Machine in"=w220) -> ("error out"=w223:errorcluster, "State Machine out"=w225:refnum<class "State Machine.lvclass">)  [unwired: 7 in]
          n75 = call-dynamic "Write State Machine.vi"("error in (no error)"=w223, "State Machine.lvclass"=w225, "Device in"=w222) -> ("error out"=w217:errorcluster, "Device out"=w218:refnum<class "Channel.lvclass">)  [unwired: 7 in]
          n76 = call-dynamic "Read sequencias.vi"("error in (no error)"=w217, "Channel in"=w218) -> ("error out"=w211:errorcluster, "sequencias"=w215:u32, "Channel out"=w216:refnum<class "Channel.lvclass">)  [unwired: 7 in]
          n77 = Number To Decimal String(number=w215) -> (decimal integer string=w213:string)  [unwired: 1 in]
          n78 = Concatenate Strings("SET WAVEPLATE_POS " ("cmd"), w213) -> (w212:string)
          n79 = call-dynamic "Write cmd.vi"("error in (no error)"=w211, "cmd"=w212, "Device in"=w216) -> ("error out"=w227:errorcluster, "Device out"=w228:refnum<class "Channel.lvclass">)  [unwired: 7 in]
          n80 = Increment(x=w219) -> (x+1=w226:i32)
        }
        frame 8 {
          # "Verifica timeout para ACS responder.\nSe estourar timeout é porque o ACS não \nrespondeu e este canal vai para 28 para \nque o erro seja detectado em\nS4ACS_GUI:HandleObservation.vi."
          # "Compara o parametro enviado com\no parametro no Acquisition Configuration\nda msg de STATUS do ACS."
          n81 = call "Verify Timer.vi"("error in (no error)"=w242, "State Machine in"=w247) -> ("error out"=w241:errorcluster, "timeout"=w240:bool, "State Machine out"=w243:refnum<class "State Machine.lvclass">)  [unwired: 7 in]
          n82 = call-dynamic "Write State Machine.vi"("error in (no error)"=w241, "State Machine.lvclass"=w243, "Device in"=w246) -> ("error out"=w244:errorcluster, "Device out"=w245:refnum<class "Channel.lvclass">)  [unwired: 7 in]
          n83 = call-dynamic "Read resp.vi"("error in (no error)"=w244, "Device in"=w245) -> ("error out"=w232:errorcluster, "resp"=w233:string, "Device out"=w231:refnum<class "Channel.lvclass">)  [unwired: 7 in]
          n84 = Unbundle By Name(w231) -> ("Interface.lvclass"=w237:refnum<class "Interface.lvclass">)
          n85 = call-dynamic "UpdateACQconf.vi"("error in (no error)"=w232, "status"=w233, "Interface in"=w237) -> ("error out"=w229:errorcluster, "ACQ conf rx"=w236:T2)  [unwired: 6 in, 1 out]
          n86 = Unbundle By Name(w236) -> ("WAVEPLATE_POS"=w235:u32)
          n87 = Unbundle By Name(w231) -> ("sequencias"=w230:u32)
          n88 = Equal?(x=w230, y=w235) -> (x = y?=w234:bool)
          n89 = case shown="False" w240 {
            tunnel: [w249 28] -> w238
            tunnel: w239 -> [w250 _]
            tunnel: w234 -> [w248 _]
            frame False {
              n90 = case shown="True" w248 {
                tunnel: [w251 w252] -> w249
                tunnel: w250 -> [w251 w253]
                frame False {
                }
                frame True {
                  n91 = Increment(x=w253) -> (x+1=w252:i32)
                }
              }
            }
            frame True {
              # "ERRO"
            }
          }
        }
        frame 9 {
          # "Carrega timeout de 200 ciclos\npara resposta do ACS"
          n92 = call-dynamic "Write Timer.vi"("error in (no error)"=w260, "Timer"=u32 200, "State Machine in"=w261) -> ("error out"=w257:errorcluster, "State Machine out"=w258:refnum<class "State Machine.lvclass">)  [unwired: 7 in]
          n93 = call-dynamic "Write State Machine.vi"("error in (no error)"=w257, "State Machine.lvclass"=w258, "Device in"=w259) -> ("error out"=w255:errorcluster, "Device out"=w256:refnum<class "Channel.lvclass">)  [unwired: 7 in]
          n94 = Unbundle By Name(w256) -> ("Interface.lvclass"=w270:refnum<class "Interface.lvclass">)
          n95 = call-dynamic "Read Temperature.vi"("Interface in"=w270) -> ("Temperature"=w267:i8)  [unwired: 8 in, 2 out]
          n96 = Number To Decimal String(number=w267) -> (decimal integer string=w266:string)  [unwired: 1 in]
          n97 = Concatenate Strings("SET TEMP " ("cmd"), w266) -> (w269:string)
          n98 = call-dynamic "Write cmd.vi"("error in (no error)"=w255, "cmd"=w269, "Device in"=w256) -> ("error out"=w271:errorcluster, "Device out"=w264:refnum<class "Channel.lvclass">)  [unwired: 7 in]
          n99 = Increment(x=w263) -> (x+1=w265:i32)
        }
        frame 10 {
          # "Verifica timeout para ACS responder.\nSe estourar timeout é porque o ACS não \nrespondeu e este canal vai para 28 para \nque o erro seja detectado em\nS4ACS_GUI:HandleObservation.vi."
          n100 = call "Verify Timer.vi"("error in (no error)"=w291, "State Machine in"=w288) -> ("error out"=w286:errorcluster, "timeout"=w284:bool, "State Machine out"=w287:refnum<class "State Machine.lvclass">)  [unwired: 7 in]
          n101 = call-dynamic "Write State Machine.vi"("error in (no error)"=w286, "State Machine.lvclass"=w287, "Device in"=w290) -> ("error out"=w285:errorcluster, "Device out"=w289:refnum<class "Channel.lvclass">)  [unwired: 7 in]
          n102 = call-dynamic "Read resp.vi"("error in (no error)"=w285, "Device in"=w289) -> ("error out"=w275:errorcluster, "resp"=w277:string, "Device out"=w276:refnum<class "Channel.lvclass">)  [unwired: 7 in]
          n103 = Unbundle By Name(w276) -> ("Interface.lvclass"=w283:refnum<class "Interface.lvclass">)
          n104 = call-dynamic "UpdateACQconf.vi"("error in (no error)"=w275, "status"=w277, "Interface in"=w283) -> ("error out"=w279:errorcluster, "ACQ conf rx"=w282:T2, "Interface out"=w280:refnum<class "Interface.lvclass">)  [unwired: 6 in]
          n105 = Unbundle By Name(w282) -> ("TEMP"=w273:dbl)
          n106 = call-dynamic "Read Temperature.vi"("error in (no error)"=w279, "Interface in"=w280) -> ("error out"=w274:errorcluster, "Temperature"=w278:i8)  [unwired: 7 in, 1 out]
          n107 = To Byte Integer(number=w273) -> (8bit integer=w272:i8)
          n108 = Equal?(x=w278, y=w272) -> (x = y?=w281:bool)
          n109 = case shown="False" w284 {
            tunnel: w281 -> [w296 _]
            tunnel: [w295 28 ("State")] -> w293
            tunnel: w292 -> [w294 _]
            frame False {
              n110 = case shown="True" w296 {
                tunnel: [w297 0 ("State")] -> w295
                tunnel: w294 -> [w297 _]
                frame False {
                }
                frame True {
                  # "OV 2024-04-2: Apenas seta a temperatura, pois \ncooler já está ligado. Fim do setup inicial para aquisição."
                }
              }
            }
            frame True {
              # "ERRO"
              # "Estourou timeour e ACS não recebeu\no valor da temperatura desejada.\nAborta o processo com erro de \nconfiguração"
            }
          }
        }
        frame 11 {
          # "Carrega timeout de 50 ciclos\npara resposta do ACS"
          n111 = call-dynamic "Write Timer.vi"("error in (no error)"=w308, "Timer"=u32 50, "State Machine in"=w307) -> ("error out"=w310:errorcluster, "State Machine out"=w312:refnum<class "State Machine.lvclass">)  [unwired: 7 in]
          n112 = call-dynamic "Write State Machine.vi"("error in (no error)"=w310, "State Machine.lvclass"=w312, "Device in"=w309) -> ("error out"=w303:errorcluster, "Device out"=w302:refnum<class "Channel.lvclass">)  [unwired: 7 in]
          n113 = Unbundle By Name(w302) -> ("Channel Status"=w301:u32)
          n114 = Number To Decimal String(number=w301) -> (decimal integer string=w300:string)  [unwired: 1 in]
          n115 = Concatenate Strings("SET CHANNELSST " ("cmd"), w300) -> (w304:string)
          n116 = call-dynamic "Write cmd.vi"("error in (no error)"=w303, "cmd"=w304, "Device in"=w302) -> ("error out"=w314:errorcluster, "Device out"=w315:refnum<class "Channel.lvclass">)  [unwired: 7 in]
          n117 = Increment(x=w306) -> (x+1=w313:i32)
        }
        frame 12 {
          n118 = call "Verify Timer.vi"("error in (no error)"=w320, "State Machine in"=w321) -> ("error out"=w325:errorcluster, "timeout"=w317:bool, "State Machine out"=w326:refnum<class "State Machine.lvclass">)  [unwired: 7 in]
          n119 = call-dynamic "Write State Machine.vi"("error in (no error)"=w325, "State Machine.lvclass"=w326, "Device in"=w324) -> ("error out"=w322:errorcluster, "Device out"=w323:refnum<class "Channel.lvclass">)  [unwired: 7 in]
          n120 = call-dynamic "Read resp.vi"("error in (no error)"=w322, "Device in"=w323) -> ("error out"=w327:errorcluster, "resp"=w330:string, "Device out"=w328:refnum<class "Channel.lvclass">)  [unwired: 7 in]
          n121 = Equal?(x=w330, y="DONE") -> (x = y?=w316:bool)
          n122 = case shown="True" w317 {
            tunnel: [w332 w338] -> w319
            tunnel: w318 -> [w333 w337]
            tunnel: w316 -> [w331 _]
            frame False {
              n123 = case shown="True" w331 {
                tunnel: [w334 w335] -> w332
                tunnel: w333 -> [w334 w336]
                frame False {
                }
                frame True {
                  n124 = Increment(x=w336) -> (x+1=w335:i32)
                }
              }
            }
            frame True {
              n125 = disable-structure shown="Enabled" {
                disable-tunnel: [28 w340] -> w338
                disable-tunnel: w337 -> [_ w341]
                frame Enabled {
                  # "ERRO"
                }
                frame Disabled {
                  # "Por enquanto, prossegue\nmesmo sem receber DONE."
                  n126 = Increment(x=w341) -> (x+1=w340:i32)
                }
              }
            }
          }
        }
        frame 13 {
          # "Carrega timeout de 50 ciclos\npara resposta do ACS"
          n127 = call-dynamic "Write Timer.vi"("error in (no error)"=w350, "Timer"=u32 50, "State Machine in"=w349) -> ("error out"=w352:errorcluster, "State Machine out"=w354:refnum<class "State Machine.lvclass">)  [unwired: 7 in]
          n128 = call-dynamic "Write State Machine.vi"("error in (no error)"=w352, "State Machine.lvclass"=w354, "Device in"=w351) -> ("error out"=w345:errorcluster, "Device out"=w344:refnum<class "Channel.lvclass">)  [unwired: 7 in]
          n129 = Unbundle By Name(w344) -> ("syncmode"=w343:bool)
          n130 = case shown="False" w343 {
            tunnel: ["ASYNC" "SYNC"] -> w342
            frame False {
            }
            frame True {
            }
          }
          n131 = Concatenate Strings("SET SYNCMODE " ("cmd"), w342) -> (w346:string)
          n132 = call-dynamic "Write cmd.vi"("error in (no error)"=w345, "cmd"=w346, "Device in"=w344) -> ("error out"=w356:errorcluster, "Device out"=w357:refnum<class "Channel.lvclass">)  [unwired: 7 in]
          n133 = Increment(x=w348) -> (x+1=w355:i32)
        }
        frame 14 {
          n134 = call "Verify Timer.vi"("error in (no error)"=w364, "State Machine in"=w365) -> ("error out"=w369:errorcluster, "timeout"=w363:bool, "State Machine out"=w370:refnum<class "State Machine.lvclass">)  [unwired: 7 in]
          n135 = call-dynamic "Write State Machine.vi"("error in (no error)"=w369, "State Machine.lvclass"=w370, "Device in"=w368) -> ("error out"=w366:errorcluster, "Device out"=w367:refnum<class "Channel.lvclass">)  [unwired: 7 in]
          n136 = call-dynamic "Read resp.vi"("error in (no error)"=w366, "Device in"=w367) -> ("error out"=w371:errorcluster, "resp"=w374:string, "Device out"=w372:refnum<class "Channel.lvclass">)  [unwired: 7 in]
          n137 = Equal?(x=w374, y="DONE") -> (x = y?=w361:bool)
          n138 = case shown="True" w363 {
            tunnel: [w376 w384] -> w360
            tunnel: w362 -> [w377 _]
            tunnel: w361 -> [w375 _]
            frame False {
              n139 = case shown="True" w375 {
                tunnel: [w378 w379] -> w376
                tunnel: w377 -> [w378 w380]
                frame False {
                }
                frame True {
                  n140 = disable-structure shown="Enabled" {
                    disable-tunnel: w380 -> [w382 _]
                    disable-tunnel: [w381 29 ("State")] -> w379
                    frame Disabled {
                      n141 = Increment(x=w382) -> (x+1=w381:i32)
                    }
                    frame Enabled {
                    }
                  }
                }
              }
            }
            frame True {
              n142 = disable-structure shown="Enabled" {
                disable-tunnel: [28 29] -> w384
                frame Enabled {
                  # "ERRO"
                }
                frame Disabled {
                  # "Por enquanto, prossegue\nmesmo sem receber DONE."
                }
              }
            }
          }
        }
        frame 27 {
          # "ESTADO DE ERRO: Falha na configuraçãodo sufixo: vide estados 300 e 301."
        }
        frame 28 {
          # "ESTADO DE ERRO: Fica aqui até que S4GUI:HandleObservationSync.vi ou S4GUI:HandleObservationAsync.vi ou os botões START, STOP, ABORT mandem para outro estado."
        }
        frame 29 {
          n143 = Unbundle By Name(w393) -> ("expose"=w395:bool)
          n144 = case shown="True" w395 {
            tunnel: [u8 0 ("State") u8 50 ("State")] -> w397
            tunnel: w396 -> [_ _]
            frame False {
            }
            frame True {
            }
          }
        }
        frame 30 {
          n145 = call-dynamic "Write Timer.vi"("error in (no error)"=w404, "Timer"=u32 50, "State Machine in"=w406) -> ("error out"=w403:errorcluster, "State Machine out"=w405:refnum<class "State Machine.lvclass">)  [unwired: 7 in]
          n146 = call-dynamic "Write State Machine.vi"("error in (no error)"=w403, "State Machine.lvclass"=w405, "Device in"=w407) -> ("error out"=w401:errorcluster, "Device out"=w402:refnum<class "Channel.lvclass">)  [unwired: 7 in]
          n147 = Unbundle By Name(w402) -> ("Interface.lvclass"=w415:refnum<class "Interface.lvclass">)
          n148 = call-dynamic "Read Cooler ON_OFF.vi"("error in (no error)"=w401, "Interface in"=w415) -> ("error out"=w400:errorcluster, "Cooler ON/OFF"=w410:i16)  [unwired: 7 in, 1 out]
          n149 = case shown="0" w410 {
            tunnel: ["1" "0"] -> w409
            frame 0 {
              (unwired) "ON"
              # "Se COOLER desligado, manda ligar."
            }
            frame 1, Default {
              (unwired) "OFF"
              # "Se COOLER ligado, manda desligar."
            }
          }
          n150 = Concatenate Strings("SET COOLER_POWER_STATUS " ("cmd"), w409) -> (w414:string)
          n151 = call-dynamic "Write cmd.vi"("error in (no error)"=w400, "cmd"=w414, "Device in"=w402) -> ("error out"=w416:errorcluster, "Device out"=w417:refnum<class "Channel.lvclass">)  [unwired: 7 in]
          n152 = Increment(x=w412) -> (x+1=w413:i32)
        }
        frame 31 {
          n153 = call "Verify Timer.vi"("error in (no error)"=w439, "State Machine in"=w436) -> ("error out"=w434:errorcluster, "timeout"=w432:bool, "State Machine out"=w435:refnum<class "State Machine.lvclass">)  [unwired: 7 in]
          n154 = call-dynamic "Write State Machine.vi"("error in (no error)"=w434, "State Machine.lvclass"=w435, "Device in"=w438) -> ("error out"=w433:errorcluster, "Device out"=w437:refnum<class "Channel.lvclass">)  [unwired: 7 in]
          n155 = call-dynamic "Read resp.vi"("error in (no error)"=w433, "Device in"=w437) -> ("error out"=w422:errorcluster, "resp"=w423:string, "Device out"=w421:refnum<class "Channel.lvclass">)  [unwired: 7 in]
          n156 = Unbundle By Name(w421) -> ("Interface.lvclass"=w431:refnum<class "Interface.lvclass">)
          n157 = call-dynamic "UpdateACQconf.vi"("error in (no error)"=w422, "status"=w423, "Interface in"=w431) -> ("error out"=w428:errorcluster, "ACQ conf rx"=w430:T2, "Interface out"=w429:refnum<class "Interface.lvclass">)  [unwired: 6 in]
          n158 = Unbundle By Name(w430) -> ("COOLER_POWER_STATUS"=w426:dbl)
          n159 = call-dynamic "Read Cooler ON_OFF.vi"("error in (no error)"=w428, "Interface in"=w429) -> ("error out"=w420:errorcluster, "Cooler ON/OFF"=w427:i16)  [unwired: 7 in, 1 out]
          n160 = To Byte Integer(number=w426) -> (8bit integer=w425:i8)
          n161 = Equal?(x=w427, y=w425) -> (x = y?=w424:bool)
          n162 = case shown="True" w432 {
            tunnel: w424 -> [w444 _]
            tunnel: [w443 w447] -> w441
            tunnel: w440 -> [w442 _]
            frame False {
              n163 = case shown="False" w444 {
                tunnel: [w445 300 ("State")] -> w443
                tunnel: w442 -> [w445 _]
                frame False {
                }
                frame True {
                }
              }
            }
            frame True {
              n164 = disable-structure shown="Enabled" {
                disable-tunnel: [0 ("State") 300 ("State")] -> w447
                frame Disabled {
                }
                frame Enabled {
                  (unwired) 12 ("State")
                  # "300: configura os\nparametros por comando\nSET"
                }
              }
            }
          }
        }
        frame 32 {
          # "Este estado não é mais usado!!"
          n165 = call-dynamic "Write Timer.vi"("error in (no error)"=w454, "Timer"=u32 50, "State Machine in"=w455) -> ("error out"=w457:errorcluster, "State Machine out"=w452:refnum<class "State Machine.lvclass">)  [unwired: 7 in]
          n166 = call-dynamic "Write State Machine.vi"("error in (no error)"=w457, "State Machine.lvclass"=w452, "Device in"=w456) -> ("error out"=w450:errorcluster, "Device out"=w451:refnum<class "Channel.lvclass">)  [unwired: 7 in]
          n167 = call-dynamic "Write cmd.vi"("error in (no error)"=w450, "cmd"="GET COOLER_POWER_STATUS ", "Device in"=w451) -> ("error out"=w461:errorcluster, "Device out"=w462:refnum<class "Channel.lvclass">)  [unwired: 7 in]
          n168 = Increment(x=w459) -> (x+1=w460:i32)
        }
        frame 33 {
          # "Este estado não é mais usado!!"
          n169 = call "Verify Timer.vi"("error in (no error)"=w466, "State Machine in"=w470) -> ("error out"=w465:errorcluster, "timeout"=w464:bool, "State Machine out"=w467:refnum<class "State Machine.lvclass">)  [unwired: 7 in]
          n170 = call-dynamic "Write State Machine.vi"("error in (no error)"=w465, "State Machine.lvclass"=w467, "Device in"=w469) -> ("error out"=w463:errorcluster, "Device out"=w468:refnum<class "Channel.lvclass">)  [unwired: 7 in]
          n171 = call-dynamic "Read resp.vi"("error in (no error)"=w463, "Device in"=w468) -> ("error out"=w475:errorcluster, "resp"=w471:string, "Device out"=w476:refnum<class "Channel.lvclass">)  [unwired: 7 in]
          n172 = case shown="False" w464 {
            tunnel: [w484 w505] -> w477
            tunnel: w476 -> [w483 w505]
            tunnel: w475 -> [w482 w504]
            tunnel: [w481 w504] -> w474
            tunnel: [w480 w503] -> w473
            tunnel: w472 -> [w479 _]
            tunnel: w471 -> [w478 _]
            frame False {
              n173 = case shown="\"0\", \"1\"" w478 {
                selector: w478 -> [_ w496]
                tunnel: [w487 w492] -> w484
                tunnel: w483 -> [w487 w500]
                tunnel: w482 -> [w486 w498]
                tunnel: [w486 w490] -> w481
                tunnel: [w485 w497] -> w480
                tunnel: w479 -> [w485 _]
                frame Default {
                }
                frame "0", "1" {
                  n174 = Decimal String To Number(string=w496) -> (number=w495:i32)  [unwired: 2 in, 1 out]
                  n175 = Unbundle By Name(w500) -> ("Interface.lvclass"=w499:refnum<class "Interface.lvclass">)
                  n176 = To Word Integer(number=w495) -> (16bit integer=w494:i16)
                  n177 = call-dynamic "Write Cooler ON_OFF.vi"("error in (no error)"=w498, "Cooler ON/OFF"=w494, "Interface in"=w499) -> ("error out"=w491:errorcluster, "Interface out"=w489:refnum<class "Interface.lvclass">)  [unwired: 7 in]
                  n178 = Bundle By Name(cluster=w500, "Interface.lvclass"=w489) -> (w493:refnum<class "Channel.lvclass">)
                  n179 = disable-structure shown="Enabled" {
                    disable-tunnel: [0 ("State") 300 ("State")] -> w497
                    frame Disabled {
                    }
                    frame Enabled {
                      (unwired) 12 ("State")
                      # "300: configura os\nparametros por comando\nSET"
                    }
                  }
                  n180 = call-dynamic "Save Temp.vi"("error in (no error)"=w491, "temp file"="lasttemp.cfg", "Channel in"=w493) -> ("error out"=w490:errorcluster, "Channel out"=w492:refnum<class "Channel.lvclass">)  [unwired: 7 in]
                }
              }
            }
            frame True {
              n181 = disable-structure shown="Enabled" {
                disable-tunnel: [0 ("State") 300 ("State")] -> w503
                frame Disabled {
                }
                frame Enabled {
                  (unwired) 12 ("State")
                  # "300: configura os\nparametros por comando\nSET"
                }
              }
            }
          }
        }
        frame 35 {
          # "Carrega timeout de 50 ciclos\n50 x 20ms = 1s\npara resposta do ACS"
          n182 = call-dynamic "Write Timer.vi"("error in (no error)"=w514, "Timer"=u32 50, "State Machine in"=w512) -> ("error out"=w510:errorcluster, "State Machine out"=w511:refnum<class "State Machine.lvclass">)  [unwired: 7 in]
          n183 = call-dynamic "Write State Machine.vi"("error in (no error)"=w510, "State Machine.lvclass"=w511, "Device in"=w513) -> ("error out"=w509:errorcluster, "Device out"=w508:refnum<class "Channel.lvclass">)  [unwired: 7 in]
          n184 = Unbundle By Name(w508) -> ("Interface.lvclass"=w523:refnum<class "Interface.lvclass">)
          n185 = call-dynamic "Read Temperature.vi"("Interface in"=w523) -> ("Temperature"=w520:i8)  [unwired: 8 in, 2 out]
          n186 = Number To Decimal String(number=w520) -> (decimal integer string=w519:string)  [unwired: 1 in]
          n187 = Concatenate Strings("SET TEMP " ("cmd"), w519) -> (w522:string)
          n188 = call-dynamic "Write cmd.vi"("error in (no error)"=w509, "cmd"=w522, "Device in"=w508) -> ("error out"=w524:errorcluster, "Device out"=w517:refnum<class "Channel.lvclass">)  [unwired: 7 in]
          n189 = Increment(x=w516) -> (x+1=w518:i32)
        }
        frame 36 {
          n190 = call "Verify Timer.vi"("error in (no error)"=w544, "State Machine in"=w541) -> ("error out"=w539:errorcluster, "timeout"=w537:bool, "State Machine out"=w540:refnum<class "State Machine.lvclass">)  [unwired: 7 in]
          n191 = call-dynamic "Write State Machine.vi"("error in (no error)"=w539, "State Machine.lvclass"=w540, "Device in"=w543) -> ("error out"=w538:errorcluster, "Device out"=w542:refnum<class "Channel.lvclass">)  [unwired: 7 in]
          n192 = call-dynamic "Read resp.vi"("error in (no error)"=w538, "Device in"=w542) -> ("error out"=w528:errorcluster, "resp"=w530:string, "Device out"=w529:refnum<class "Channel.lvclass">)  [unwired: 7 in]
          n193 = Unbundle By Name(w529) -> ("Interface.lvclass"=w536:refnum<class "Interface.lvclass">)
          n194 = call-dynamic "UpdateACQconf.vi"("error in (no error)"=w528, "status"=w530, "Interface in"=w536) -> ("error out"=w532:errorcluster, "ACQ conf rx"=w535:T2, "Interface out"=w533:refnum<class "Interface.lvclass">)  [unwired: 6 in]
          n195 = Unbundle By Name(w535) -> ("TEMP"=w526:dbl)
          n196 = call-dynamic "Read Temperature.vi"("error in (no error)"=w532, "Interface in"=w533) -> ("error out"=w527:errorcluster, "Temperature"=w531:i8)  [unwired: 7 in, 1 out]
          n197 = To Byte Integer(number=w526) -> (8bit integer=w525:i8)
          n198 = Equal?(x=w531, y=w525) -> (x = y?=w534:bool)
          n199 = case shown="True" w537 {
            tunnel: w534 -> [w549 _]
            tunnel: [w548 w553] -> w546
            tunnel: w545 -> [w547 _]
            frame False {
              n200 = case shown="True" w549 {
                tunnel: [w550 w551] -> w548
                tunnel: w547 -> [w550 w552]
                frame False {
                }
                frame True {
                  # "OV 2022-11-16: Ao setar a temperatura, liga \nautomaticamente o COLLER."
                  n201 = Increment(x=w552) -> (x+1=w551:i32)
                }
              }
            }
            frame True {
              n202 = disable-structure shown="Enabled" {
                disable-tunnel: [0 ("State") 300 ("State")] -> w553
                frame Disabled {
                }
                frame Enabled {
                  (unwired) 12 ("State")
                  # "300: configura os\nparametros por comando\nSET e WAIT_EXPOSE_COMMAND"
                }
              }
            }
          }
        }
        frame 37 {
          # "Liga COOLER"
          n203 = call-dynamic "Write Timer.vi"("error in (no error)"=w561, "Timer"=u32 50, "State Machine in"=w563) -> ("error out"=w560:errorcluster, "State Machine out"=w562:refnum<class "State Machine.lvclass">)  [unwired: 7 in]
          n204 = call-dynamic "Write State Machine.vi"("error in (no error)"=w560, "State Machine.lvclass"=w562, "Device in"=w564) -> ("error out"=w558:errorcluster, "Device out"=w557:refnum<class "Channel.lvclass">)  [unwired: 7 in]
          n205 = call-dynamic "Write cmd.vi"("error in (no error)"=w558, "cmd"="SET COOLER_POWER_STATUS 1", "Device in"=w557) -> ("error out"=w566:errorcluster, "Device out"=w567:refnum<class "Channel.lvclass">)  [unwired: 7 in]
        }
        frame 38 {
          # "ESTADO DE ERRO: Texp incompativel com a configuração do CCD;\nFica aqui até que S4GUI:HandleObservationSync.vi ou S4GUI:HandleObservationAsync.vi ou os botões START, STOP, ABORT mandem para outro estado."
        }
        frame 40 {
          n206 = disable-structure shown="Disabled" {
            disable-tunnel: [w591 w593] -> w585
            disable-tunnel: w584 -> [w589 w593]
            disable-tunnel: w582 -> [w588 w592]
            disable-tunnel: [w587 w592] -> w581
            frame Disabled {
              # "Carrega timeout de 10 ciclos\npara resposta do ACS"
              n207 = call-dynamic "Write Timer.vi"("error in (no error)"=w588, "Timer"=u32 10, "State Machine in"=w589) -> ("error out"=w587:errorcluster, "State Machine out"=w591:refnum<class "State Machine.lvclass">)  [unwired: 7 in]
            }
            frame Enabled {
            }
          }
          n208 = call-dynamic "Write State Machine.vi"("error in (no error)"=w581, "State Machine.lvclass"=w585, "Device in"=w583) -> ("error out"=w580:errorcluster, "Device out"=w577:refnum<class "Channel.lvclass">)  [unwired: 7 in]
          n209 = Unbundle By Name(w577) -> ("wait_expose"=w576:bool)
          n210 = Select(t="ON", s=w576, f="OFF") -> (s? t:f=w573:string)
          n211 = Concatenate Strings("WAIT_EXPOSE_COMMAND " ("cmd"), w573) -> (w572:string)
          n212 = call-dynamic "Write cmd.vi"("error in (no error)"=w580, "cmd"=w572, "Device in"=w577) -> ("error out"=w586:errorcluster, "Device out"=w571:refnum<class "Channel.lvclass">)  [unwired: 7 in]
        }
        frame 50 {
          n213 = Bundle By Name(cluster=w596, "stopping"=FALSE) -> (w594:refnum<class "Channel.lvclass">)
          n214 = call-dynamic "Write cmd.vi"("error in (no error)"=w602, "cmd"="EXPOSE", "Device in"=w594) -> ("error out"=w599:errorcluster, "Device out"=w600:refnum<class "Channel.lvclass">)  [unwired: 7 in]
          n215 = disable-structure shown="Enabled" {
            disable-tunnel: w605 -> [w609 w612]
            disable-tunnel: [w606 w610] -> w603
            disable-tunnel: w601 -> [_ w619]
            disable-tunnel: w600 -> [w608 w617]
            disable-tunnel: w599 -> [w607 w615]
            disable-tunnel: [w608 w616] -> w598
            disable-tunnel: [w607 w613] -> w597
            frame Disabled {
              # "OV 2024-03-12:\nVai para a pausa antes\ndo pedido de STATUS"
              n216 = Increment(x=w609) -> (x+1=w606:i32)
            }
            frame Enabled {
              # "Força a recarga do Ticks com\no valor do relógio do PC.\n\n2024-03-20: Nao precisa mais \npedir STATUS, pois ACS o publica\na cada 1s."
              n217 = call-dynamic "Verif Clock.vi"("error in (no error)"=w615, "period (ms)"=u32 1 ("period"), "State Machine in"=w619) -> ("error out"=w614:errorcluster, "State Machine out"=w618:refnum<class "State Machine.lvclass">)  [unwired: 6 in, 1 out]
              n218 = Add(x=w612, y=3) -> (x+y=w610:i32)
              n219 = call-dynamic "Write State Machine.vi"("error in (no error)"=w614, "State Machine.lvclass"=w618, "Device in"=w617) -> ("error out"=w613:errorcluster, "Device out"=w616:refnum<class "Channel.lvclass">)  [unwired: 7 in]
            }
          }
        }
        frame 51 {
          # "ESTADO OPCIONAL:\nEspera estourar o timeout (200ms).\nApós o timeout vai para o próximo estado enviar STATUS para confirmar\nse o ACS  foi para ACTIVE."
          n220 = call-dynamic "Verif Clock.vi"("error in (no error)"=w627, "period (ms)"=u32 200 ("period"), "State Machine in"=w631) -> ("error out"=w626:errorcluster, "State Machine out"=w630:refnum<class "State Machine.lvclass">)  [unwired: 6 in, 1 out]
          n221 = call-dynamic "Read Timeout.vi"("error in (no error)"=w626, "State Machine in"=w630) -> ("error out"=w625:errorcluster, "Timeout"=w628:bool, "State Machine out"=w629:refnum<class "State Machine.lvclass">)  [unwired: 7 in]
          n222 = call-dynamic "Write State Machine.vi"("error in (no error)"=w625, "State Machine.lvclass"=w629, "Device in"=w633) -> ("error out"=w624:errorcluster, "Device out"=w623:refnum<class "Channel.lvclass">)  [unwired: 7 in]
          n223 = case shown="True" w628 {
            tunnel: [w638 w641] -> w635
            tunnel: w634 -> [w638 w642]
            tunnel: w624 -> [w636 w639]
            tunnel: w623 -> [w637 w640]
            tunnel: [w637 w640] -> w622
            tunnel: [w636 w639] -> w621
            frame False {
            }
            frame True {
              n224 = Increment(x=w642) -> (x+1=w641:i32)
            }
          }
        }
        frame 52 {
          n225 = disable-structure shown="Enabled" {
            disable-tunnel: [w653 w655] -> w648
            disable-tunnel: [w652 w654] -> w647
            disable-tunnel: w644 -> [w650 w655]
            disable-tunnel: w643 -> [w649 w654]
            frame Disabled {
              n226 = call-dynamic "Write cmd.vi"("error in (no error)"=w649, "cmd"="STATUS", "Device in"=w650) -> ("error out"=w652:errorcluster, "Device out"=w653:refnum<class "Channel.lvclass">)  [unwired: 7 in]
            }
            frame Enabled {
              # "ACS publica STATUS"
            }
          }
          n227 = Increment(x=w645) -> (x+1=w646:i32)
        }
        frame 53 {
          # "Status.Texp = Current frame exptime\nlastStatus = cam status (acquiring, idle, writing, reading, ...)\nStatus.Nimages = frames done\nStatus.CubesDone = ciclos realizados pelo ACS\nStatus.SequesDone = sequencias realizadas pelo ACS.\nStatus.UsedDiskSpace = espaco usado no disco.\nStatus.Error = Se TRUE, houve erro na aquisição do canal."
          # "Verifica timeout para ACS iniciar exposição.\nSe estourar timeout é porque o ACS não \nrecebeu o EXPOSE e então volta para 50\npara enviar novo EXPOSE."
          # "Extrair todos os parametros da respsota de STATUS e\natualizar a informação na classe Channel."
          n228 = call-dynamic "Verif Clock.vi"("error in (no error)"=w667, "period (ms)"=u32 500 ("period"), "State Machine in"=w670) -> ("error out"=w668:errorcluster, "State Machine out"=w669:refnum<class "State Machine.lvclass">)  [unwired: 6 in, 1 out]
          n229 = call-dynamic "Read Timeout.vi"("error in (no error)"=w668, "State Machine in"=w669) -> ("error out"=w681:errorcluster, "Timeout"=w671:bool, "State Machine out"=w682:refnum<class "State Machine.lvclass">)  [unwired: 7 in]
          n230 = call-dynamic "Write State Machine.vi"("error in (no error)"=w681, "State Machine.lvclass"=w682, "Device in"=w680) -> ("error out"=w678:errorcluster, "Device out"=w679:refnum<class "Channel.lvclass">)  [unwired: 7 in]
          n231 = call-dynamic "Read resp.vi"("error in (no error)"=w678, "Device in"=w679) -> ("error out"=w700:errorcluster, "resp"=w701:string, "Device out"=w704:refnum<class "Channel.lvclass">)  [unwired: 7 in]
          "resposta do STATUS" <- w701
          n232 = call-dynamic "Read Interface.vi"("error in (no error)"=w700, "Channel in"=w704) -> ("error out"=w699:errorcluster, "Interface.lvclass"=w702:refnum<class "Interface.lvclass">, "Channel out"=w703:refnum<class "Channel.lvclass">)  [unwired: 7 in]
          n233 = call-dynamic "UpdateStatus.vi"("error in (no error)"=w699, "status"=w701, "Interface in"=w702) -> ("error out"=w658:errorcluster, "Interface out"=w660:refnum<class "Interface.lvclass">)  [unwired: 7 in]
          n234 = call-dynamic "Read Error.vi"("error in (no error)"=w658, "Interface in"=w660) -> ("error out"=w657:errorcluster, "Error"=w656:bool, "Interface out"=w659:refnum<class "Interface.lvclass">)  [unwired: 7 in]
          n235 = call-dynamic "Read Exposições realizadas.vi"("error in (no error)"=w657, "Interface in"=w659) -> ("error out"=w687:errorcluster, "Exposições realizadas"=w688:dbl, "Interface out"=w689:refnum<class "Interface.lvclass">)  [unwired: 7 in]
          n236 = call-dynamic "Read Cam_Status.vi"("error in (no error)"=w687, "Interface in"=w689) -> ("error out"=w695:errorcluster, "Cam_Status"=w683:string, "Interface out"=w696:refnum<class "Interface.lvclass">)  [unwired: 7 in]
          n237 = call-dynamic "Read %Acquired.vi"("error in (no error)"=w695, "Interface in"=w696) -> ("error out"=w676:errorcluster, "% Acquired"=w692:dbl, "Interface out"=w677:refnum<class "Interface.lvclass">)  [unwired: 7 in]
          n238 = call-dynamic "Read Number of Cycles.vi"("error in (no error)"=w676, "Interface in"=w677) -> ("error out"=w673:errorcluster, "Number of Cycles"=w675:u32, "Interface out"=w674:refnum<class "Interface.lvclass">)  [unwired: 7 in]
          n239 = call-dynamic "Read Number of Sequences.vi"("error in (no error)"=w673, "Interface in"=w674) -> ("error out"=w663:errorcluster, "Number of Sequences"=w672:u32, "Interface out"=w665:refnum<class "Interface.lvclass">)  [unwired: 7 in]
          n240 = call-dynamic "Read Ocupacao do disco.vi"("error in (no error)"=w663, "Interface in"=w665) -> ("error out"=w662:errorcluster, "Ocupacao do disco"=w661:u16, "Interface out"=w664:refnum<class "Interface.lvclass">)  [unwired: 7 in]
          n241 = call "Read Exposure Time.vi"("error in (no error)"=w662, "Interface in"=w664) -> ("error out"=w685:errorcluster, "Exposure Time"=w694:dbl, "Interface out"=w684:refnum<class "Interface.lvclass">)  [unwired: 7 in]
          n242 = call-dynamic "Write Interface.vi"("error in (no error)"=w685, "Interface.lvclass"=w684, "Channel in"=w703) -> ("error out"=w698:errorcluster, "Channel out"=w697:refnum<class "Channel.lvclass">)  [unwired: 7 in]
          n243 = case shown="Default" w683 {
            tunnel: [w708 w710] -> w707
            tunnel: w706 -> [w709 w710]
            tunnel: w671 -> [_ _]
            frame "ACTIVE" {
              n244 = Increment(x=w709) -> (x+1=w708:i32)
            }
            frame Default {
              # "Não usa o timeout. Deixa o \nS4GUI:HandleObservationSync.vi  e ..Async.vi\ndetectarem o timeout no estado 53."
            }
          }
          n245 = To Unsigned Long Integer(number=w688) -> (unsigned 32bit integer=w686:u32)
          n246 = Divide(x=w692, y=100.0) -> (x/y=w690:dbl)
          n247 = Multiply(x=w694, y=w690) -> (x*y=w693:dbl)
          n248 = Bundle By Name(cluster=w697, "Texp"=w693, "lastStatus"=w683, "Nimages"=w686, "CyclesDone"=w675, "SequesDone"=w672, "UsedDiskSpace"=w661, "Error"=w656) -> (w705:refnum<class "Channel.lvclass">)
        }
        frame 54 {
          # "Verifica o timeout de 5s para enviar\ntelemetria para o ACS."
          n249 = call-dynamic "Verif Clock 2.vi"("error in (no error)"=w723, "period (ms)"=u32 5000 ("period"), "State Machine in"=w724) -> ("error out"=w721:errorcluster, "State Machine out"=w722:refnum<class "State Machine.lvclass">)  [unwired: 6 in, 1 out]
          n250 = call-dynamic "Read Timeout 2.vi"("error in (no error)"=w721, "State Machine in"=w722) -> ("error out"=w717:errorcluster, "Timeout 2"=w720:bool, "State Machine out"=w718:refnum<class "State Machine.lvclass">)  [unwired: 7 in]
          n251 = call-dynamic "Write State Machine.vi"("error in (no error)"=w717, "State Machine.lvclass"=w718, "Device in"=w719) -> ("error out"=w716:errorcluster, "Device out"=w715:refnum<class "Channel.lvclass">)  [unwired: 7 in]
          n252 = case shown="False" w720 {
            tunnel: [w740 w749] -> w714
            tunnel: [w739 w750] -> w713
            tunnel: [w738 w751] -> w727
            tunnel: w726 -> [w737 w748]
            tunnel: w715 -> [w736 w749]
            tunnel: w716 -> [w735 w750]
            frame False {
              n253 = disable-structure shown="Enabled" {
                disable-tunnel: [w745 w747] -> w740
                disable-tunnel: [w744 w746] -> w739
                disable-tunnel: w736 -> [w742 w747]
                disable-tunnel: w735 -> [w741 w746]
                frame Disabled {
                  n254 = call-dynamic "Write cmd.vi"("error in (no error)"=w741, "cmd"="STATUS", "Device in"=w742) -> ("error out"=w744:errorcluster, "Device out"=w745:refnum<class "Channel.lvclass">)  [unwired: 7 in]
                }
                frame Enabled {
                  # "2024_03_20: Nao pede mais STATUS,\npois ACS o publica a cada 1s."
                }
              }
              n255 = Increment(x=w737) -> (x+1=w738:i32)
            }
            frame True {
              n256 = disable-structure shown="Enabled" {
                disable-tunnel: [59 w753] -> w751
                disable-tunnel: w748 -> [_ w753]
                frame Disabled {
                  # "Estourou timeout de 5s:\nDesvia para enviar dados de \nTELEMETRIA a cada 5s (estado 59)"
                }
                frame Enabled {
                  # "2024-03020: Não evia mais dados\nda TELEMETRIA, pois ACS assina\nas publicacoes do S4GUI, TCS, etc."
                }
              }
            }
          }
          n257 = disable-structure shown="Disabled" {
            disable-tunnel: w714 -> [w731 w734]
            disable-tunnel: w713 -> [w730 w733]
            disable-tunnel: [w729 w734] -> w712
            disable-tunnel: [w728 w733] -> w711
            frame Disabled {
              n258 = call "Write connected.vi"("error in (no error)"=w730, "connected"=FALSE, "Device in"=w731) -> ("error out"=w728:errorcluster, "Device out"=w729:refnum<class "Channel.lvclass">)  [unwired: 7 in]
            }
            frame Enabled {
            }
          }
        }
        frame 55 {
          # "Status.Texp = Current frame exptime\nlastStatus = cam status (acquiring, idle, writing, reading, ...)\nStatus.Nimages = frames done\nStatus.CubesDone = ciclos realizados pelo ACS\nStatus.SequesDone = sequencias realizadas pelo ACS.\nStatus.UsedDiskSpace = espaco usado no disco.\nStatus.Error = Se TRUE, houve erro na aquisição do canal."
          # "Extrair todos os parametros da respsota de STATUS e\natualizar a informação na classe Channel."
          n259 = call-dynamic "Verif Clock.vi"("error in (no error)"=w768, "period (ms)"=u32 500 ("period"), "State Machine in"=w771) -> ("error out"=w767:errorcluster, "State Machine out"=w770:refnum<class "State Machine.lvclass">)  [unwired: 6 in, 1 out]
          n260 = call-dynamic "Read Timeout.vi"("error in (no error)"=w767, "State Machine in"=w770) -> ("error out"=w765:errorcluster, "Timeout"=w766:bool, "State Machine out"=w769:refnum<class "State Machine.lvclass">)  [unwired: 7 in]
          n261 = call-dynamic "Read resp.vi"("error in (no error)"=w765, "Device in"=w778) -> ("error out"=w798:errorcluster, "resp"=w799:string, "Device out"=w802:refnum<class "Channel.lvclass">)  [unwired: 7 in]
          n262 = call-dynamic "Read Interface.vi"("error in (no error)"=w798, "Channel in"=w802) -> ("error out"=w797:errorcluster, "Interface.lvclass"=w800:refnum<class "Interface.lvclass">, "Channel out"=w801:refnum<class "Channel.lvclass">)  [unwired: 7 in]
          n263 = call-dynamic "UpdateStatus.vi"("error in (no error)"=w797, "status"=w799, "Interface in"=w800) -> ("error out"=w756:errorcluster, "Interface out"=w758:refnum<class "Interface.lvclass">)  [unwired: 7 in]
          n264 = call-dynamic "Read Error.vi"("error in (no error)"=w756, "Interface in"=w758) -> ("error out"=w755:errorcluster, "Error"=w754:bool, "Interface out"=w757:refnum<class "Interface.lvclass">)  [unwired: 7 in]
          n265 = call-dynamic "Read Exposições realizadas.vi"("error in (no error)"=w755, "Interface in"=w757) -> ("error out"=w785:errorcluster, "Exposições realizadas"=w786:dbl, "Interface out"=w787:refnum<class "Interface.lvclass">)  [unwired: 7 in]
          n266 = call-dynamic "Read Cam_Status.vi"("error in (no error)"=w785, "Interface in"=w787) -> ("error out"=w794:errorcluster, "Cam_Status"=w783:string, "Interface out"=w796:refnum<class "Interface.lvclass">)  [unwired: 7 in]
          n267 = call-dynamic "Read %Acquired.vi"("error in (no error)"=w794, "Interface in"=w796) -> ("error out"=w793:errorcluster, "% Acquired"=w790:dbl, "Interface out"=w795:refnum<class "Interface.lvclass">)  [unwired: 7 in]
          n268 = call "Read Exposure Time.vi"("error in (no error)"=w793, "Interface in"=w795) -> ("error out"=w776:errorcluster, "Exposure Time"=w792:dbl, "Interface out"=w777:refnum<class "Interface.lvclass">)  [unwired: 7 in]
          n269 = call-dynamic "Read Number of Cycles.vi"("error in (no error)"=w776, "Interface in"=w777) -> ("error out"=w773:errorcluster, "Number of Cycles"=w775:u32, "Interface out"=w774:refnum<class "Interface.lvclass">)  [unwired: 7 in]
          n270 = call-dynamic "Read Number of Sequences.vi"("error in (no error)"=w773, "Interface in"=w774) -> ("error out"=w762:errorcluster, "Number of Sequences"=w772:u32, "Interface out"=w763:refnum<class "Interface.lvclass">)  [unwired: 7 in]
          n271 = call-dynamic "Read Ocupacao do disco.vi"("error in (no error)"=w762, "Interface in"=w763) -> ("error out"=w761:errorcluster, "Ocupacao do disco"=w759:u16, "Interface out"=w760:refnum<class "Interface.lvclass">)  [unwired: 7 in]
          n272 = call-dynamic "Write Interface.vi"("error in (no error)"=w761, "Interface.lvclass"=w760, "Channel in"=w801) -> ("error out"=w782:errorcluster, "Channel out"=w781:refnum<class "Channel.lvclass">)  [unwired: 7 in]
          n273 = case shown="Default" w783 {
            tunnel: [w814 w823 w837] -> w805
            tunnel: w804 -> [_ w824 w838]
            tunnel: w782 -> [w812 w819 w835]
            tunnel: [w809 w821 w832] -> w780
            tunnel: w781 -> [w810 w822 w836]
            tunnel: [w806 w818 w829] -> w779
            tunnel: w769 -> [w813 w820 w834]
            tunnel: w766 -> [_ w817 w828]
            frame "ACQUISITION_ABORTED" {
              # "250x20ms=5s"
              n274 = call-dynamic "Write Timer.vi"("error in (no error)"=w812, "Timer"=u32 250, "State Machine in"=w813) -> ("error out"=w807:errorcluster, "State Machine out"=w808:refnum<class "State Machine.lvclass">)  [unwired: 7 in]
              n275 = call-dynamic "Write State Machine.vi"("error in (no error)"=w807, "State Machine.lvclass"=w808, "Device in"=w810) -> ("error out"=w806:errorcluster, "Device out"=w809:refnum<class "Channel.lvclass">)  [unwired: 7 in]
              n276 = disable-structure shown="Enabled" {
                disable-tunnel: [32 ("State") 0 ("State")] -> w814
                frame Disabled {
                }
                frame Enabled {
                  # "OVJ 20230704"
                }
              }
            }
            frame "ACTIVE", "IDLE", "WAITING_EXPOSE_COMMAND" {
              # "STATUS DETECTOR = ACTIVE or WAITING EXPOSE COMMAND"
              n277 = case shown="True" w817 {
                tunnel: w824 -> [w825 w827]
                tunnel: [w825 w826] -> w823
                frame False {
                }
                frame True {
                  n278 = Decrement(x=w827) -> (x-1=w826:i32)
                }
              }
              n279 = call-dynamic "Write State Machine.vi"("error in (no error)"=w819, "State Machine.lvclass"=w820, "Device in"=w822) -> ("error out"=w818:errorcluster, "Device out"=w821:refnum<class "Channel.lvclass">)  [unwired: 7 in]
            }
            frame Default {
              # "STATUS \ndesconhecido\nou IDLE"
              n280 = case shown="False" w828 {
                tunnel: w838 -> [w840 _]
                tunnel: [w839 0] -> w837
                tunnel: w836 -> [w843 w846]
                tunnel: [w843 w846] -> w833
                tunnel: w835 -> [w842 w847]
                tunnel: [w842 w844] -> w830
                tunnel: w834 -> [w841 w849]
                tunnel: [w841 w845] -> w831
                frame False {
                  n281 = Decrement(x=w840) -> (x-1=w839:i32)
                }
                frame True {
                  n282 = call-dynamic "Write Timer.vi"("error in (no error)"=w847, "Timer"=u32 250, "State Machine in"=w849) -> ("error out"=w844:errorcluster, "State Machine out"=w845:refnum<class "State Machine.lvclass">)  [unwired: 7 in]
                }
              }
              n283 = call-dynamic "Write State Machine.vi"("error in (no error)"=w830, "State Machine.lvclass"=w831, "Device in"=w833) -> ("error out"=w829:errorcluster, "Device out"=w832:refnum<class "Channel.lvclass">)  [unwired: 7 in]
            }
          }
          n284 = To Unsigned Long Integer(number=w786) -> (unsigned 32bit integer=w784:u32)
          n285 = Divide(x=w790, y=100.0) -> (x/y=w788:dbl)
          n286 = Multiply(x=w792, y=w788) -> (x*y=w791:dbl)
          n287 = Bundle By Name(cluster=w780, "Texp"=w791, "lastStatus"=w783, "Nimages"=w784, "CyclesDone"=w775, "SequesDone"=w772, "UsedDiskSpace"=w759, "Error"=w754) -> (w803:refnum<class "Channel.lvclass">)
        }
        frame 56 {
          # "Pedido de STATUS para verificar conexão com ACS"
          # "Carrega timeout de 10 ciclos \n(20 x 20ms = 0.4s) \npara resposta do ACS"
          n288 = call-dynamic "Write Timer.vi"("error in (no error)"=w856, "Timer"=u32 20, "State Machine in"=w860) -> ("error out"=w861:errorcluster, "State Machine out"=w862:refnum<class "State Machine.lvclass">)  [unwired: 7 in]
          n289 = call-dynamic "Write State Machine.vi"("error in (no error)"=w861, "State Machine.lvclass"=w862, "Device in"=w858) -> ("error out"=w855:errorcluster, "Device out"=w857:refnum<class "Channel.lvclass">)  [unwired: 7 in]
          n290 = disable-structure shown="Enabled" {
            disable-tunnel: w857 -> [w875 w878]
            disable-tunnel: w855 -> [w874 w877]
            disable-tunnel: [w873 w878] -> w854
            disable-tunnel: [w872 w877] -> w853
            frame Disabled {
              n291 = call-dynamic "Write cmd.vi"("error in (no error)"=w874, "cmd"="STATUS", "Device in"=w875) -> ("error out"=w872:errorcluster, "Device out"=w873:refnum<class "Channel.lvclass">)  [unwired: 7 in]
            }
            frame Enabled {
              # "2024-03-20: Não envia mais pedido\nde STATUS, pois o ACS publica seu\nSTATUS a cada 1s."
            }
          }
          n292 = Increment(x=w863) -> (x+1=w864:i32)
          n293 = disable-structure shown="Disabled" {
            disable-tunnel: w854 -> [w869 w871]
            disable-tunnel: w853 -> [w868 w870]
            disable-tunnel: [w867 w871] -> w852
            disable-tunnel: [w866 w870] -> w851
            frame Disabled {
              # "2024.05.16\ncausa bug de\nfalsa queda na\ncomunicação \ncom ACS"
              n294 = call "Write connected.vi"("error in (no error)"=w868, "connected"=FALSE, "Device in"=w869) -> ("error out"=w866:errorcluster, "Device out"=w867:refnum<class "Channel.lvclass">)  [unwired: 7 in]
            }
            frame Enabled {
            }
          }
        }
        frame 57 {
          # "Status.Texp = Current frame exptime\nlastStatus = cam status (acquiring, idle, writing, reading, ...)\nStatus.Nimages = frames done\nStatus.CubesDone = ciclos realizados pelo ACS\nStatus.SequesDone = sequencias realizadas pelo ACS.\nStatus.UsedDiskSpace = espaco usado no disco.\nStatus.Error = Se TRUE, houve erro na aquisção do canal."
          # "Extrair todos os parametros da respsota de STATUS e\natualizar a informação na classe Channel."
          n295 = call "Verify Timer.vi"("error in (no error)"=w905, "State Machine in"=w904) -> ("error out"=w901:errorcluster, "State Machine out"=w903:refnum<class "State Machine.lvclass">)  [unwired: 7 in, 1 out]
          n296 = call-dynamic "Read Timeout.vi"("error in (no error)"=w901, "State Machine in"=w903) -> ("error out"=w896:errorcluster, "Timeout"=w900:bool, "State Machine out"=w902:refnum<class "State Machine.lvclass">)  [unwired: 7 in]
          n297 = call "Read connected.vi"("error in (no error)"=w896, "Device in"=w899) -> ("error out"=w897:errorcluster, "connected"=w895:bool, "Device out"=w898:refnum<class "Channel.lvclass">)  [unwired: 7 in]
          n298 = call-dynamic "Read resp.vi"("error in (no error)"=w897, "Device in"=w898) -> ("error out"=w925:errorcluster, "resp"=w926:string, "Device out"=w929:refnum<class "Channel.lvclass">)  [unwired: 7 in]
          n299 = call-dynamic "Read Interface.vi"("error in (no error)"=w925, "Channel in"=w929) -> ("error out"=w924:errorcluster, "Interface.lvclass"=w927:refnum<class "Interface.lvclass">, "Channel out"=w928:refnum<class "Channel.lvclass">)  [unwired: 7 in]
          n300 = call-dynamic "UpdateStatus.vi"("error in (no error)"=w924, "status"=w926, "Interface in"=w927) -> ("error out"=w881:errorcluster, "Interface out"=w883:refnum<class "Interface.lvclass">)  [unwired: 7 in]
          n301 = call-dynamic "Read Error.vi"("error in (no error)"=w881, "Interface in"=w883) -> ("error out"=w880:errorcluster, "Error"=w879:bool, "Interface out"=w882:refnum<class "Interface.lvclass">)  [unwired: 7 in]
          n302 = call-dynamic "Read Exposições realizadas.vi"("error in (no error)"=w880, "Interface in"=w882) -> ("error out"=w912:errorcluster, "Exposições realizadas"=w913:dbl, "Interface out"=w914:refnum<class "Interface.lvclass">)  [unwired: 7 in]
          n303 = call-dynamic "Read Cam_Status.vi"("error in (no error)"=w912, "Interface in"=w914) -> ("error out"=w921:errorcluster, "Cam_Status"=w910:string, "Interface out"=w923:refnum<class "Interface.lvclass">)  [unwired: 7 in]
          n304 = call-dynamic "Read %Acquired.vi"("error in (no error)"=w921, "Interface in"=w923) -> ("error out"=w920:errorcluster, "% Acquired"=w917:dbl, "Interface out"=w922:refnum<class "Interface.lvclass">)  [unwired: 7 in]
          n305 = call "Read Exposure Time.vi"("error in (no error)"=w920, "Interface in"=w922) -> ("error out"=w893:errorcluster, "Exposure Time"=w919:dbl, "Interface out"=w894:refnum<class "Interface.lvclass">)  [unwired: 7 in]
          n306 = call-dynamic "Read Number of Cycles.vi"("error in (no error)"=w893, "Interface in"=w894) -> ("error out"=w890:errorcluster, "Number of Cycles"=w892:u32, "Interface out"=w891:refnum<class "Interface.lvclass">)  [unwired: 7 in]
          n307 = call-dynamic "Read Number of Sequences.vi"("error in (no error)"=w890, "Interface in"=w891) -> ("error out"=w886:errorcluster, "Number of Sequences"=w889:u32, "Interface out"=w888:refnum<class "Interface.lvclass">)  [unwired: 7 in]
          n308 = call-dynamic "Read Ocupacao do disco.vi"("error in (no error)"=w886, "Interface in"=w888) -> ("error out"=w885:errorcluster, "Ocupacao do disco"=w884:u16, "Interface out"=w887:refnum<class "Interface.lvclass">)  [unwired: 7 in]
          n309 = call-dynamic "Write Interface.vi"("error in (no error)"=w885, "Interface.lvclass"=w887, "Channel in"=w928) -> ("error out"=w909:errorcluster, "Channel out"=w908:refnum<class "Channel.lvclass">)  [unwired: 7 in]
          n310 = case shown="False" w895 {
            tunnel: [w935 w952] -> w932
            tunnel: w931 -> [w936 w953]
            tunnel: w909 -> [w933 w950]
            tunnel: [w938 w947] -> w907
            tunnel: w908 -> [w939 w951]
            tunnel: [w937 w944] -> w906
            tunnel: w902 -> [w934 w949]
            tunnel: w900 -> [_ w943]
            frame True {
              # "Conneted=T\nACS respondeu"
              n311 = disable-structure shown="Enabled" {
                disable-tunnel: w936 -> [w941 _]
                disable-tunnel: [w940 0] -> w935
                frame Disabled {
                  n312 = Increment(x=w941) -> (x+1=w940:i32)
                }
                frame Enabled {
                }
              }
              n313 = call-dynamic "Write State Machine.vi"("error in (no error)"=w933, "State Machine.lvclass"=w934, "Device in"=w939) -> ("error out"=w937:errorcluster, "Device out"=w938:refnum<class "Channel.lvclass">)  [unwired: 7 in]
            }
            frame False {
              # "Conneted=F\nACS não resp."
              n314 = case shown="True" w943 {
                tunnel: w953 -> [w954 _]
                tunnel: [w954 0] -> w952
                tunnel: w951 -> [w957 w960]
                tunnel: [w957 w960] -> w948
                tunnel: w950 -> [w956 w961]
                tunnel: [w956 w958] -> w945
                tunnel: w949 -> [w955 w963]
                tunnel: [w955 w959] -> w946
                frame False {
                }
                frame True {
                  n315 = call-dynamic "Write Timer.vi"("error in (no error)"=w961, "Timer"=u32 250, "State Machine in"=w963) -> ("error out"=w958:errorcluster, "State Machine out"=w959:refnum<class "State Machine.lvclass">)  [unwired: 7 in]
                }
              }
              n316 = call-dynamic "Write State Machine.vi"("error in (no error)"=w945, "State Machine.lvclass"=w946, "Device in"=w948) -> ("error out"=w944:errorcluster, "Device out"=w947:refnum<class "Channel.lvclass">)  [unwired: 7 in]
            }
          }
          n317 = Divide(x=w917, y=100.0) -> (x/y=w915:dbl)
          n318 = To Unsigned Long Integer(number=w913) -> (unsigned 32bit integer=w911:u32)
          n319 = Multiply(x=w919, y=w915) -> (x*y=w918:dbl)
          n320 = Bundle By Name(cluster=w907, "Texp"=w918, "lastStatus"=w910, "Nimages"=w911, "CyclesDone"=w892, "SequesDone"=w889, "UsedDiskSpace"=w884, "Error"=w879) -> (w930:refnum<class "Channel.lvclass">)
        }
        frame 58 {
          w969 = "}" ("regular expression")
          # "Passa valores da telemetria adquiridos do TCS"
          n321 = call-dynamic "Write State Machine.vi"("error in (no error)"=w965, "State Machine.lvclass"=w966, "Device in"=w976) -> ("error out"=w973:errorcluster, "Device out"=w975:refnum<class "Channel.lvclass">)  [unwired: 7 in]
          n322 = Unbundle By Name(w975) -> ("TCS telemetry"=w970:string, "Filter"=w972:u8)
          n323 = Match Pattern(string=w970, regular expression=w969) -> (before substring=w968:string, match substring=w967:string)  [unwired: 1 in, 2 out]
          n324 = Equal?(x=w967, y=w969) -> (x = y?=w971:bool)
          n325 = case shown="True" w971 {
            tunnel: [w980 w990] -> w978
            tunnel: [w979 w989] -> w977
            tunnel: w975 -> [w980 w988]
            tunnel: w973 -> [w979 w985]
            tunnel: w972 -> [_ w984]
            tunnel: w968 -> [_ w983]
            tunnel: w967 -> [_ w982]
            frame False {
            }
            frame True {
              (unwired) "\"CTRLINTE\":\"S4GUI\"}" ("string")
              (unwired) "\"FILTER\":\"" ("string")
              n326 = case shown="5" w984 {
                tunnel: ["CLEAR\"," ("string") "U\"," ("string") "B\"," ("string") "V\"," ("string") "R\"," ("string") "S\"," ("string")] -> _
                frame 0, Default {
                }
                frame 1 {
                }
                frame 2 {
                }
                frame 3 {
                }
                frame 4 {
                }
                frame 5 {
                }
              }
              n327 = Concatenate Strings(w983, w982) -> (w981:string)
              n328 = Concatenate Strings("WRITE_HEADER_DATA " ("cmd"), w981) -> (w986:string)
              n329 = disable-structure shown="Enabled" {
                disable-tunnel: [w995 w997] -> w990
                disable-tunnel: [w994 w996] -> w989
                disable-tunnel: w988 -> [w993 w997]
                disable-tunnel: w986 -> [w992 _]
                disable-tunnel: w985 -> [w991 w996]
                frame Disabled {
                  n330 = call-dynamic "Write cmd.vi"("error in (no error)"=w991, "cmd"=w992, "Device in"=w993) -> ("error out"=w994:errorcluster, "Device out"=w995:refnum<class "Channel.lvclass">)  [unwired: 7 in]
                }
                frame Enabled {
                  # "Não existe mais\neste comando."
                }
              }
            }
          }
        }
        frame 59 {
          w1008 = "}" ("regular expression")
          # "Passa valores da telemetria adquiridos do TCS durante a aquisição do canal (estados 54 e 55)"
          n331 = call-dynamic "Write State Machine.vi"("error in (no error)"=w1004, "State Machine.lvclass"=w1005, "Device in"=w1014) -> ("error out"=w1011:errorcluster, "Device out"=w1013:refnum<class "Channel.lvclass">)  [unwired: 7 in]
          n332 = Unbundle By Name(w1013) -> ("TCS telemetry"=w1009:string)
          n333 = Match Pattern(string=w1009, regular expression=w1008) -> (before substring=w1007:string, match substring=w1006:string)  [unwired: 1 in, 2 out]
          n334 = Equal?(x=w1006, y=w1008) -> (x = y?=w1010:bool)
          n335 = case shown="True" w1010 {
            tunnel: [w1018 w1027] -> w1016
            tunnel: [w1017 w1026] -> w1015
            tunnel: w1013 -> [w1018 w1025]
            tunnel: w1011 -> [w1017 w1022]
            tunnel: w1007 -> [_ w1021]
            tunnel: w1006 -> [_ w1020]
            frame False {
            }
            frame True {
              n336 = Concatenate Strings(w1021, w1020) -> (w1019:string)
              n337 = Concatenate Strings("WRITE_HEADER_DATA " ("cmd"), w1019) -> (w1023:string)
              n338 = disable-structure shown="Enabled" {
                disable-tunnel: [w1032 w1034] -> w1027
                disable-tunnel: [w1031 w1033] -> w1026
                disable-tunnel: w1025 -> [w1030 w1034]
                disable-tunnel: w1023 -> [w1029 _]
                disable-tunnel: w1022 -> [w1028 w1033]
                frame Disabled {
                  n339 = call-dynamic "Write cmd.vi"("error in (no error)"=w1028, "cmd"=w1029, "Device in"=w1030) -> ("error out"=w1031:errorcluster, "Device out"=w1032:refnum<class "Channel.lvclass">)  [unwired: 7 in]
                }
                frame Enabled {
                  # "Não existe mais\neste comando."
                }
              }
            }
          }
        }
        frame 60 {
          # "Carrega timeout de 5 ciclos\npara resposta do ACS"
          n340 = call-dynamic "Write Timer.vi"("Timer"=u32 5, "State Machine in"=w1040) -> ("error out"=w1041:errorcluster, "State Machine out"=w1039:refnum<class "State Machine.lvclass">)  [unwired: 8 in]
          n341 = call-dynamic "Write State Machine.vi"("error in (no error)"=w1041, "State Machine.lvclass"=w1039, "Device in"=w1038) -> ("Device out"=w1037:refnum<class "Channel.lvclass">)  [unwired: 7 in, 1 out]
          n342 = disable-structure shown="Enabled" {
            disable-tunnel: [w1052 w1054] -> w1045
            disable-tunnel: w1044 -> [w1051 w1053]
            disable-tunnel: [w1050 w1053] -> w1043
            disable-tunnel: w1037 -> [w1048 w1054]
            disable-tunnel: w1036 -> [w1047 _]
            disable-tunnel: [w1046 62] -> w1035
            frame Disabled {
              n343 = Increment(x=w1047) -> (x+1=w1046:i32)
              n344 = call-dynamic "Write cmd.vi"("error in (no error)"=w1051, "cmd"="INIT", "Device in"=w1048) -> ("error out"=w1050:errorcluster, "Device out"=w1052:refnum<class "Channel.lvclass">)  [unwired: 7 in]
            }
            frame Enabled {
            }
          }
        }
        frame 61 {
          w1065 = "INITIALIZATION"
          # "Verifica timeout para ACS responder.\nSe estourar timeout é porque o ACS não \nrespondeu e este canal volta para o estado 0\npara não \"travar\" os outros canais no \nS4ACS_GUI:HandleObservation.vi."
          n345 = call "Verify Timer.vi"("error in (no error)"=w1056, "State Machine in"=w1061) -> ("error out"=w1062:errorcluster, "timeout"=w1057:bool, "State Machine out"=w1063:refnum<class "State Machine.lvclass">)  [unwired: 7 in]
          n346 = call-dynamic "Write State Machine.vi"("error in (no error)"=w1062, "State Machine.lvclass"=w1063, "Device in"=w1060) -> ("error out"=w1058:errorcluster, "Device out"=w1059:refnum<class "Channel.lvclass">)  [unwired: 7 in]
          n347 = call-dynamic "Read resp.vi"("error in (no error)"=w1058, "Device in"=w1059) -> ("error out"=w1069:errorcluster, "resp"=w1067:string, "Device out"=w1070:refnum<class "Channel.lvclass">)  [unwired: 7 in]
          "resp INIT" <- w1067
          n348 = Match Pattern(string=w1067, regular expression=w1065) -> (match substring=w1066:string)  [unwired: 1 in, 3 out]
          n349 = Equal?(x=w1066, y=w1065) -> (x = y?=w1064:bool)
          n350 = case shown="True" w1064 {
            tunnel: [w1072 w1077] -> w1071
            tunnel: w1068 -> [w1073 w1078]
            tunnel: w1057 -> [w1074 _]
            frame False {
              n351 = case shown="False" w1074 {
                tunnel: [w1075 0 ("State")] -> w1072
                tunnel: w1073 -> [w1075 _]
                frame False {
                }
                frame True {
                }
              }
            }
            frame True {
              n352 = disable-structure shown="Enabled" {
                disable-tunnel: w1078 -> [w1080 _]
                disable-tunnel: [w1079 54] -> w1077
                frame Disabled {
                  n353 = Increment(x=w1080) -> (x+1=w1079:i32)
                }
                frame Enabled {
                  # "debug:\nNão deve enviar\n WRITE_SETUP para o \nACS antigo"
                }
              }
            }
          }
        }
        frame 62 {
          # "Aguarda para reconfigurar.\n(o timer deve ser recarregado \nquando SM:NextState.vi recebe 62).\n\nIsso foi inserido para dar tempo\ndas VIs de ZMQ estarem prontas\npara enviar e receber mensagens \ndos ACS após o S4GUI:Initialize.vi."
          n354 = call "Verify Timer.vi"("error in (no error)"=w1085, "State Machine in"=w1086) -> ("error out"=w1082:errorcluster, "timeout"=w1087:bool, "State Machine out"=w1084:refnum<class "State Machine.lvclass">)  [unwired: 7 in]
          n355 = case shown="True" w1087 {
            tunnel: [w1095 w1118] -> w1091
            tunnel: [w1096 w1117] -> w1090
            tunnel: w1089 -> [w1097 w1115]
            tunnel: [w1097 w1109] -> w1088
            tunnel: w1082 -> [w1092 w1100]
            tunnel: w1084 -> [w1094 w1102]
            tunnel: w1083 -> [w1093 w1104]
            frame False {
              n356 = call-dynamic "Write State Machine.vi"("error in (no error)"=w1092, "State Machine.lvclass"=w1094, "Device in"=w1093) -> ("error out"=w1096:errorcluster, "Device out"=w1095:refnum<class "Channel.lvclass">)  [unwired: 7 in]
            }
            frame True {
              # "Salta para estado 65\npara tratar a próxima\npublicação de STATUS\n do ACS."
              n357 = call-dynamic "Write Timer.vi"("error in (no error)"=w1100, "Timer"=u32 50, "State Machine in"=w1102) -> ("error out"=w1099:errorcluster, "State Machine out"=w1101:refnum<class "State Machine.lvclass">)  [unwired: 7 in]
              n358 = call-dynamic "Write State Machine.vi"("error in (no error)"=w1099, "State Machine.lvclass"=w1101, "Device in"=w1104) -> ("error out"=w1098:errorcluster, "Device out"=w1103:refnum<class "Channel.lvclass">)  [unwired: 7 in]
              n359 = call-dynamic "Read target cluster.vi"("error in (no error)"=w1098, "Channel in"=w1103) -> ("error out"=w1107:errorcluster, "target cluster"=w1108:T3, "Channel out"=w1106:refnum<class "Channel.lvclass">)  [unwired: 7 in]
              n360 = Increment(x=w1115) -> (x+1=w1116:i32)
              n361 = Flatten To JSON(anything=w1108, error in (no error)=w1107) -> (JSON string=w1112:string, 11:w1111:errorcluster)  [unwired: 1 in]
              n362 = Increment(x=w1116) -> (x+1=w1110:i32)
              n363 = Increment(x=w1110) -> (x+1=w1109:i32)
              n364 = Concatenate Strings("WRITE_SETUP " ("cmd"), w1112) -> (w1113:string)
              n365 = call-dynamic "Write cmd.vi"("error in (no error)"=w1111, "cmd"=w1113, "Device in"=w1106) -> ("error out"=w1117:errorcluster, "Device out"=w1118:refnum<class "Channel.lvclass">)  [unwired: 7 in]
            }
          }
        }
        frame 63 {
          # "Não há resposta para o comando WRTITE_SETUP\nQuando estourar timeout vai para o estado 64 para \nobter o STATUS do ACS."
          n366 = call "Verify Timer.vi"("error in (no error)"=w1122, "State Machine in"=w1124) -> ("error out"=w1125:errorcluster, "timeout"=w1121:bool, "State Machine out"=w1126:refnum<class "State Machine.lvclass">)  [unwired: 7 in]
          n367 = call-dynamic "Write State Machine.vi"("error in (no error)"=w1125, "State Machine.lvclass"=w1126, "Device in"=w1123) -> ("error out"=w1119:errorcluster, "Device out"=w1120:refnum<class "Channel.lvclass">)  [unwired: 7 in]
          n368 = case shown="True" w1121 {
            tunnel: [w1129 w1130] -> w1128
            tunnel: w1127 -> [w1129 w1131]
            frame False {
            }
            frame True {
              n369 = Increment(x=w1131) -> (x+1=w1130:i32)
            }
          }
        }
        frame 64 {
          # "Carrega timeout de 50 ciclos\npara resposta do ACS"
          n370 = call-dynamic "Write Timer.vi"("error in (no error)"=w1134, "Timer"=u32 50, "State Machine in"=w1137) -> ("error out"=w1138:errorcluster, "State Machine out"=w1136:refnum<class "State Machine.lvclass">)  [unwired: 7 in]
          n371 = call-dynamic "Write State Machine.vi"("error in (no error)"=w1138, "State Machine.lvclass"=w1136, "Device in"=w1135) -> ("error out"=w1132:errorcluster, "Device out"=w1133:refnum<class "Channel.lvclass">)  [unwired: 7 in]
          n372 = disable-structure shown="Enabled" {
            disable-tunnel: [w1148 w1150] -> w1143
            disable-tunnel: [w1147 w1149] -> w1142
            disable-tunnel: w1133 -> [w1146 w1150]
            disable-tunnel: w1132 -> [w1144 w1149]
            frame Disabled {
              n373 = call-dynamic "Write cmd.vi"("error in (no error)"=w1144, "cmd"="READ_SETUP ", "Device in"=w1146) -> ("error out"=w1147:errorcluster, "Device out"=w1148:refnum<class "Channel.lvclass">)  [unwired: 7 in]
            }
            frame Enabled {
            }
          }
          n374 = Increment(x=w1140) -> (x+1=w1141:i32)
        }
        frame 65 {
          n375 = call "Verify Timer.vi"("error in (no error)"=w1170, "State Machine in"=w1172) -> ("error out"=w1173:errorcluster, "timeout"=w1159:bool, "State Machine out"=w1174:refnum<class "State Machine.lvclass">)  [unwired: 7 in]
          n376 = call-dynamic "Write State Machine.vi"("error in (no error)"=w1173, "State Machine.lvclass"=w1174, "Device in"=w1171) -> ("error out"=w1168:errorcluster, "Device out"=w1169:refnum<class "Channel.lvclass">)  [unwired: 7 in]
          n377 = call-dynamic "Read resp.vi"("error in (no error)"=w1168, "Device in"=w1169) -> ("error out"=w1164:errorcluster, "resp"=w1154:string, "Device out"=w1151:refnum<class "Channel.lvclass">)  [unwired: 7 in]
          n378 = disable-structure shown="Enabled" {
            disable-tunnel: w1151 -> [w1175 w1190]
            disable-tunnel: [w1182 w1185] -> w1166
            disable-tunnel: [w1181 w1187] -> w1165
            disable-tunnel: w1164 -> [w1179 w1188]
            disable-tunnel: [w1178 w1184] -> w1163
            disable-tunnel: w1154 -> [w1177 w1189]
            disable-tunnel: [w1176 w1183] -> w1153
            disable-tunnel: [w1175 w1186] -> w1152
            frame Disabled {
              n379 = Unbundle By Name(w1175) -> ("Interface.lvclass"=w1180:refnum<class "Interface.lvclass">)
              n380 = call-dynamic "UpdateCCDconf.vi"("error in (no error)"=w1179, "status"=w1177, "Interface in"=w1180) -> ("error out"=w1181:errorcluster, "CCD conf rx"=w1178:T3, "Cluster comparison"=w1176:T1, "Interface out"=w1182:refnum<class "Interface.lvclass">)  [unwired: 5 in]
            }
            frame Enabled {
              n381 = call-dynamic "Check CCD Config.vi"("error in (no error)"=w1188, "Status"=w1189, "Channel in"=w1190) -> ("error out"=w1187:errorcluster, "cluster RX"=w1184:T3, "Cluster COMPARE"=w1183:T1, "Channel out"=w1186:refnum<class "Channel.lvclass">)  [unwired: 5 in]
              n382 = Unbundle By Name(w1186) -> ("Interface.lvclass"=w1185:refnum<class "Interface.lvclass">)
            }
          }
          n383 = case shown="True" w1159 {
            tunnel: w1166 -> [w1193 w1208]
            tunnel: w1165 -> [w1192 w1207]
            tunnel: w1163 -> [_ w1203]
            tunnel: [w1193 w1206] -> w1161
            tunnel: [w1192 w1205] -> w1162
            tunnel: [w1194 w1202] -> w1160
            tunnel: w1156 -> [w1191 w1204]
            tunnel: [w1191 w1199] -> w1155
            tunnel: w1153 -> [_ w1202]
            frame False {
              n384 = disable-structure shown="Enabled" {
                disable-tunnel: [T1 {"ACQUISITION_MODE"=FALSE, "TRIGGER_MODE"=FALSE, "READ_MODE"=FALSE, "PREAMP"=FALSE, "READOUT_RATE"=FALSE, "VERTICAL_SHIFT_SPEED"=FALSE, "EM_MODE"=FALSE, "EM_GAIN"=FALSE, "SHUTTER_MODE"=FALSE, "SHUTTER_TTL"=FALSE, "SHUTTER_OPENING_TIME"=FALSE, "SHUTTER_CLOSING_TIME"=FALSE, "VBIN"=FALSE, "HBIN"=FALSE, "INITIAL_LINE"=FALSE, "INITIAL_COLUMN"=FALSE, "FINAL_LINE"=FALSE, "FINAL_COLUMN"=FALSE, "FRAME_TRANSFER"=FALSE, "VERTICAL_CLOCK_VOLTAGE"=FALSE, "AD_CHANNEL"=FALSE} ("x = y?") T1 {"ACQUISITION_MODE"=TRUE, "TRIGGER_MODE"=TRUE, "READ_MODE"=TRUE, "PREAMP"=TRUE, "READOUT_RATE"=TRUE, "VERTICAL_SHIFT_SPEED"=TRUE, "EM_MODE"=TRUE, "EM_GAIN"=TRUE, "SHUTTER_MODE"=TRUE, "SHUTTER_TTL"=TRUE, "SHUTTER_OPENING_TIME"=TRUE, "SHUTTER_CLOSING_TIME"=TRUE, "VBIN"=TRUE, "HBIN"=TRUE, "INITIAL_LINE"=TRUE, "INITIAL_COLUMN"=TRUE, "FINAL_LINE"=TRUE, "FINAL_COLUMN"=TRUE, "FRAME_TRANSFER"=TRUE, "VERTICAL_CLOCK_VOLTAGE"=TRUE, "AD_CHANNEL"=TRUE} ("x = y?")] -> w1194
                frame Disabled {
                }
                frame Enabled {
                }
              }
            }
            frame True {
              n385 = Not Equal?(x=T1 {"ACQUISITION_MODE"=TRUE, "TRIGGER_MODE"=TRUE, "READ_MODE"=TRUE, "PREAMP"=TRUE, "READOUT_RATE"=TRUE, "VERTICAL_SHIFT_SPEED"=TRUE, "EM_MODE"=TRUE, "EM_GAIN"=TRUE, "SHUTTER_MODE"=TRUE, "SHUTTER_TTL"=TRUE, "SHUTTER_OPENING_TIME"=TRUE, "SHUTTER_CLOSING_TIME"=TRUE, "VBIN"=TRUE, "HBIN"=TRUE, "INITIAL_LINE"=TRUE, "INITIAL_COLUMN"=TRUE, "FINAL_LINE"=TRUE, "FINAL_COLUMN"=TRUE, "FRAME_TRANSFER"=TRUE, "VERTICAL_CLOCK_VOLTAGE"=TRUE, "AD_CHANNEL"=TRUE}, y=w1202) -> (x != y?=w1200:bool)
              n386 = Increment(x=w1204) -> (x+1=w1197:i32)
              n387 = call-dynamic "Set CCD_Config.vi"("error in (no error)"=w1207, "input cluster"=w1203, "Interface in"=w1208) -> ("error out"=w1205:errorcluster, "Interface out"=w1206:refnum<class "Interface.lvclass">)  [unwired: 7 in]
              n388 = Select(t=27 ("f"), s=w1200, f=w1197) -> (s? t:f=w1199:i32)
            }
          }
          "x = y?" <- w1160
          n389 = call "Write Checked Params.vi"("error in (no error)"=w1162, "Checked Params"=w1160, "Interface in"=w1161) -> ("error out"=w1157:errorcluster, "Interface out"=w1158:refnum<class "Interface.lvclass">)  [unwired: 7 in]
          n390 = Bundle By Name(cluster=w1152, "Interface.lvclass"=w1158) -> (w1167:refnum<class "Channel.lvclass">)
        }
        frame 66 {
          # "O valor do COOLER aqui\nfoi carregado no Acquistion:Init.vi"
          # "Se COOLER=0\n        SET COLLERPOWER_STATUS 0\n        AVANÇA ESTADO\n        VAI PRA 0\nSe COOLER=1:\n      DESVIA PARA Estado 35"
          # "Carrega timeout de 50 ciclos\npara resposta do ACS"
          n391 = call-dynamic "Write Timer.vi"("error in (no error)"=w1216, "Timer"=u32 50, "State Machine in"=w1217) -> ("error out"=w1214:errorcluster, "State Machine out"=w1213:refnum<class "State Machine.lvclass">)  [unwired: 7 in]
          n392 = call-dynamic "Write State Machine.vi"("error in (no error)"=w1214, "State Machine.lvclass"=w1213, "Device in"=w1215) -> ("error out"=w1212:errorcluster, "Device out"=w1211:refnum<class "Channel.lvclass">)  [unwired: 7 in]
          n393 = Unbundle By Name(w1211) -> ("Interface.lvclass"=w1210:refnum<class "Interface.lvclass">)
          n394 = call-dynamic "Read Cooler ON_OFF.vi"("Interface in"=w1210) -> ("Cooler ON/OFF"=w1209:i16)  [unwired: 8 in, 2 out]
          n395 = case shown="1" w1209 {
            tunnel: [w1225 w1232] -> w1222
            tunnel: [w1224 w1231] -> w1221
            tunnel: [35 w1230] -> w1220
            tunnel: w1219 -> [_ w1229]
            tunnel: w1212 -> [w1224 w1227]
            tunnel: w1211 -> [w1225 w1226]
            frame 1 {
              # "Se COOLER foi carregado com 1 na inicialização.\ndesvia para 35 para setar a temperatura e ligar o COOLER."
            }
            frame 0, Default {
              n396 = Increment(x=w1229) -> (x+1=w1230:i32)
              n397 = call-dynamic "Write cmd.vi"("error in (no error)"=w1227, "cmd"="SET COOLER_POWER_STATUS 0", "Device in"=w1226) -> ("error out"=w1231:errorcluster, "Device out"=w1232:refnum<class "Channel.lvclass">)  [unwired: 7 in]
            }
          }
        }
        frame 67 {
          # "Compara o parametro enviado com\no parametro no Acquisition Configuration\nda msg de STATUS do ACS."
          n398 = call "Verify Timer.vi"("error in (no error)"=w1248, "State Machine in"=w1252) -> ("error out"=w1247:errorcluster, "timeout"=w1245:bool, "State Machine out"=w1249:refnum<class "State Machine.lvclass">)  [unwired: 7 in]
          n399 = call-dynamic "Write State Machine.vi"("error in (no error)"=w1247, "State Machine.lvclass"=w1249, "Device in"=w1251) -> ("error out"=w1246:errorcluster, "Device out"=w1250:refnum<class "Channel.lvclass">)  [unwired: 7 in]
          n400 = call-dynamic "Read resp.vi"("error in (no error)"=w1246, "Device in"=w1250) -> ("error out"=w1237:errorcluster, "resp"=w1238:string, "Device out"=w1233:refnum<class "Channel.lvclass">)  [unwired: 7 in]
          n401 = Unbundle By Name(w1233) -> ("Interface.lvclass"=w1244:refnum<class "Interface.lvclass">)
          n402 = call-dynamic "UpdateACQconf.vi"("error in (no error)"=w1237, "status"=w1238, "Interface in"=w1244) -> ("error out"=w1239:errorcluster, "ACQ conf rx"=w1242:T2, "Interface out"=w1243:refnum<class "Interface.lvclass">)  [unwired: 6 in]
          n403 = Unbundle By Name(w1242) -> ("COOLER_POWER_STATUS"=w1240:dbl)
          n404 = call-dynamic "Read Cooler ON_OFF.vi"("error in (no error)"=w1239, "Interface in"=w1243) -> ("error out"=w1235:errorcluster, "Cooler ON/OFF"=w1241:i16)  [unwired: 7 in, 1 out]
          n405 = To Word Integer(number=w1240) -> (16bit integer=w1234:i16)
          n406 = Equal?(x=w1241, y=w1234) -> (x = y?=w1236:bool)
          n407 = case shown="False" w1236 {
            tunnel: [w1255 w1260] -> w1254
            tunnel: w1253 -> [w1256 _]
            tunnel: w1245 -> [w1257 _]
            frame False {
              n408 = case shown="True" w1257 {
                tunnel: [w1258 300 ("State")] -> w1255
                tunnel: w1256 -> [w1258 _]
                frame False {
                }
                frame True {
                  (unwired) 40 ("State")
                  # "2024.07.01:\nConfigura\nsuffix e  \nExp mode."
                }
              }
            }
            frame True {
              n409 = disable-structure shown="Enabled" {
                disable-tunnel: [54 ("State") 300 ("State")] -> w1260
                frame Disabled {
                }
                frame Enabled {
                  # "Fim. Vai para 300\nsetar Suffix e\nhabilitar WAIT_\nEXPOSE_COMMAND"
                }
              }
            }
          }
        }
        frame 70 {
          w1266 = "" ("resp")
          # "Carrega timeout de 5 ciclos\npara resposta do ACS"
          n410 = call-dynamic "Write Timer.vi"("error in (no error)"=w1279, "Timer"=u32 5, "State Machine in"=w1281) -> ("error out"=w1283:errorcluster, "State Machine out"=w1282:refnum<class "State Machine.lvclass">)  [unwired: 7 in]
          n411 = call-dynamic "Write State Machine.vi"("error in (no error)"=w1283, "State Machine.lvclass"=w1282, "Device in"=w1280) -> ("error out"=w1278:errorcluster, "Device out"=w1265:refnum<class "Channel.lvclass">)  [unwired: 7 in]
          n412 = Bundle By Name(cluster=w1265, "stopping"=TRUE) -> (w1263:refnum<class "Channel.lvclass">)
          n413 = call-dynamic "Write cmd.vi"("error in (no error)"=w1278, "cmd"="STOP_ACQUISITION", "Device in"=w1263) -> ("error out"=w1276:errorcluster, "Device out"=w1277:refnum<class "Channel.lvclass">)  [unwired: 7 in]
          n414 = call-dynamic "Write resp.vi"("error in (no error)"=w1276, "resp"=w1266, "Device in"=w1277) -> ("error out"=w1272:errorcluster, "Device out"=w1275:refnum<class "Channel.lvclass">)  [unwired: 7 in]
          n415 = call-dynamic "Read Interface.vi"("error in (no error)"=w1272, "Channel in"=w1275) -> ("error out"=w1271:errorcluster, "Interface.lvclass"=w1270:refnum<class "Interface.lvclass">, "Channel out"=w1274:refnum<class "Channel.lvclass">)  [unwired: 7 in]
          n416 = call-dynamic "UpdateStatus.vi"("error in (no error)"=w1271, "status"=w1266, "Interface in"=w1270) -> ("error out"=w1268:errorcluster, "Interface out"=w1269:refnum<class "Interface.lvclass">)  [unwired: 7 in]
          n417 = call-dynamic "Write Interface.vi"("error in (no error)"=w1268, "Interface.lvclass"=w1269, "Channel in"=w1274) -> ("error out"=w1267:errorcluster, "Channel out"=w1273:refnum<class "Channel.lvclass">)  [unwired: 7 in]
          n418 = Increment(x=w1286) -> (x+1=w1287:i32)
        }
        frame 71 {
          w1289 = "DONE"
          n419 = call-dynamic "Read resp.vi"("error in (no error)"=w1296, "Device in"=w1297) -> ("error out"=w1293:errorcluster, "resp"=w1291:string, "Device out"=w1294:refnum<class "Channel.lvclass">)  [unwired: 7 in]
          "resp STOP" <- w1291
          n420 = Match Pattern(string=w1291, regular expression=w1289) -> (match substring=w1290:string)  [unwired: 1 in, 3 out]
          n421 = Equal?(x=w1290, y=w1289) -> ()  [unwired: 1 out]
          n422 = case shown="True" TRUE {
            tunnel: [w1298 0 ("State")] -> w1295
            tunnel: w1292 -> [w1298 _]
            frame False {
            }
            frame True {
            }
          }
        }
        frame 80 {
          n423 = call-dynamic "Write cmd.vi"("error in (no error)"=w1309, "cmd"="ABORT_ACQUISITION", "Device in"=w1308) -> ("error out"=w1303:errorcluster, "Device out"=w1304:refnum<class "Channel.lvclass">)  [unwired: 7 in]
          n424 = call-dynamic "Write resp.vi"("error in (no error)"=w1303, "resp"="", "Device in"=w1304) -> ("error out"=w1302:errorcluster, "Device out"=w1301:refnum<class "Channel.lvclass">)  [unwired: 7 in]
          n425 = Increment(x=w1306) -> (x+1=w1307:i32)
        }
        frame 81 {
          w1311 = "DONE"
          n426 = call-dynamic "Read resp.vi"("error in (no error)"=w1318, "Device in"=w1319) -> ("error out"=w1315:errorcluster, "resp"=w1313:string, "Device out"=w1316:refnum<class "Channel.lvclass">)  [unwired: 7 in]
          "resp ABORT" <- w1313
          n427 = Match Pattern(string=w1313, regular expression=w1311) -> (match substring=w1312:string)  [unwired: 1 in, 3 out]
          n428 = Equal?(x=w1312, y=w1311) -> ()  [unwired: 1 out]
          n429 = case shown="True" TRUE {
            tunnel: [w1320 0 ("State")] -> w1317
            tunnel: w1314 -> [w1320 _]
            frame False {
            }
            frame True {
            }
          }
        }
        frame 90 {
          n430 = Unbundle By Name(w1323) -> ("wait_expose"=w1322:bool)
          n431 = case shown="False" w1322 {
            tunnel: w1331 -> [w1336 w1337]
            tunnel: w1323 -> [w1335 w1338]
            tunnel: [w1334 w1338] -> w1328
            tunnel: [w1333 w1337] -> w1327
            frame False {
              # "20240710: Se o ACS não estiver\nesperando EXPOSE, manda pausar a\naquisição."
              n432 = call-dynamic "Write cmd.vi"("error in (no error)"=w1336, "cmd"="PAUSE_ACQUISITION", "Device in"=w1335) -> ("error out"=w1333:errorcluster, "Device out"=w1334:refnum<class "Channel.lvclass">)  [unwired: 7 in]
            }
            frame True {
            }
          }
          n433 = call-dynamic "Write resp.vi"("error in (no error)"=w1327, "resp"="", "Device in"=w1328) -> ("error out"=w1326:errorcluster, "Device out"=w1325:refnum<class "Channel.lvclass">)  [unwired: 7 in]
          n434 = Increment(x=w1329) -> (x+1=w1330:i32)
        }
        frame 91 {
          w1340 = "DONE"
          # "Volta pra repouso para que os indicadores de progresso da aquisição sejam atualizados na GUI."
          n435 = call-dynamic "Read resp.vi"("error in (no error)"=w1345, "Device in"=w1346) -> ("error out"=w1343:errorcluster, "resp"=w1342:string, "Device out"=w1344:refnum<class "Channel.lvclass">)  [unwired: 7 in]
          "resp PAUSE" <- w1342
          n436 = Match Pattern(string=w1342, regular expression=w1340) -> (match substring=w1341:string)  [unwired: 1 in, 3 out]
          n437 = Equal?(x=w1341, y=w1340) -> ()  [unwired: 1 out]
        }
        frame 96 {
          n438 = Unbundle By Name(w1348) -> ("wait_expose"=w1347:bool)
          n439 = case shown="False" w1347 {
            tunnel: w1356 -> [w1361 w1362]
            tunnel: w1348 -> [w1360 w1363]
            tunnel: [w1359 w1363] -> w1353
            tunnel: [w1358 w1362] -> w1352
            frame False {
              # "20240710: Se o ACS não estiver\nesperando EXPOSE, manda reiniciar\na aquisição."
              n440 = call-dynamic "Write cmd.vi"("error in (no error)"=w1361, "cmd"="RESUME_ACQUISITION", "Device in"=w1360) -> ("error out"=w1358:errorcluster, "Device out"=w1359:refnum<class "Channel.lvclass">)  [unwired: 7 in]
            }
            frame True {
            }
          }
          n441 = call-dynamic "Write resp.vi"("error in (no error)"=w1352, "resp"="", "Device in"=w1353) -> ("error out"=w1351:errorcluster, "Device out"=w1350:refnum<class "Channel.lvclass">)  [unwired: 7 in]
          n442 = Increment(x=w1354) -> (x+1=w1355:i32)
        }
        frame 97 {
          w1366 = "DONE"
          # "No estado 500 de S4GUI:HandleObservationSync.vi e S4GUI:HandleObservationAsync.vi\né feita a verificação se o canal foi pra repouso (estados 0,56,57 de Channel:Run.vi). \nSe foi, o estado de retorno do canal é recarregado e o processo continua de onde parou."
          n443 = call-dynamic "Read resp.vi"("error in (no error)"=w1370, "Device in"=w1371) -> ("error out"=w1365:errorcluster, "resp"=w1368:string, "Device out"=w1369:refnum<class "Channel.lvclass">)  [unwired: 7 in]
          "resp RESUME" <- w1368
          n444 = Match Pattern(string=w1368, regular expression=w1366) -> (match substring=w1367:string)  [unwired: 1 in, 3 out]
          n445 = Equal?(x=w1367, y=w1366) -> ()  [unwired: 1 out]
        }
        frame 100 {
          (unwired) "S4ACS C1/C2/C3/C4 NIMAGES " ("cmd")
          n446 = call-dynamic "Write cmd.vi"("error in (no error)"=w1377, "cmd"="INIT", "Device in"=w1375) -> ("error out"=w1376:errorcluster, "Device out"=w1378:refnum<class "Channel.lvclass">)  [unwired: 7 in]
          n447 = Increment(x=w1373) -> (x+1=w1374:i32)
        }
        frame 101 {
          w1380 = "\r\n"
          n448 = call-dynamic "Read resp.vi"("error in (no error)"=w1388, "Device in"=w1389) -> ("error out"=w1385:errorcluster, "resp"=w1379:string, "Device out"=w1382:refnum<class "Channel.lvclass">)  [unwired: 7 in]
          n449 = Match Pattern(string=w1379, regular expression=w1380) -> (match substring=w1383:string)  [unwired: 1 in, 3 out]
          n450 = Equal?(x=w1383, y=w1380) -> (x = y?=w1387:bool)
          n451 = case shown="False" w1387 {
            tunnel: [w1390 u8 0] -> w1386
            tunnel: w1384 -> [w1390 _]
            tunnel: w1382 -> [w1391 w1395]
            tunnel: [w1391 w1394] -> w1381
            tunnel: w1379 -> [_ w1393]
            frame False {
            }
            frame True {
              n452 = Bundle By Name(cluster=w1395, "lastStatus"=w1393) -> (w1394:refnum<class "Channel.lvclass">)
            }
          }
        }
        frame 102 {
          w1403 = "EXPTIME "
          n453 = Unbundle By Name(w1397) -> ("lastStatus"=w1398:string)
          n454 = Match Pattern(string=w1398, regular expression=w1403) -> (match substring=w1402:string, after substring=w1400:string)  [unwired: 1 in, 2 out]
          n455 = Equal?(x=w1402, y=w1403) -> (x = y?=w1406:bool)
          n456 = case shown="True" w1406 {
            tunnel: [w1407 w1409] -> w1405
            tunnel: w1404 -> [w1407 w1409]
            tunnel: w1397 -> [w1408 w1415]
            tunnel: [w1408 w1413] -> w1401
            tunnel: w1400 -> [_ w1411]
            frame False {
            }
            frame True {
              n457 = call <vilib>:"Space Constant.vi"() -> ("String"=w1412:string)
              n458 = Match Pattern(string=w1411, regular expression=w1412) -> (before substring=w1410:string)  [unwired: 1 in, 3 out]
              n459 = Fract/Exp String To Number(string=w1410) -> (number=w1414:dbl)  [unwired: 3 in, 1 out]
              n460 = Bundle By Name(cluster=w1415, "Texp"=w1414) -> (w1413:refnum<class "Channel.lvclass">)
            }
          }
          n461 = Increment(x=w1405) -> (x+1=w1396:i32)
        }
        frame 103 {
          w1423 = "NIMAGES "
          n462 = Unbundle By Name(w1417) -> ("lastStatus"=w1418:string)
          n463 = Match Pattern(string=w1418, regular expression=w1423) -> (match substring=w1422:string, after substring=w1420:string)  [unwired: 1 in, 2 out]
          n464 = Equal?(x=w1422, y=w1423) -> (x = y?=w1426:bool)
          n465 = case shown="True" w1426 {
            tunnel: [w1427 w1429] -> w1425
            tunnel: w1424 -> [w1427 w1429]
            tunnel: w1417 -> [w1428 w1435]
            tunnel: [w1428 w1433] -> w1421
            tunnel: w1420 -> [_ w1431]
            frame False {
            }
            frame True {
              n466 = call <vilib>:"Space Constant.vi"() -> ("String"=w1432:string)
              n467 = Match Pattern(string=w1431, regular expression=w1432) -> (before substring=w1430:string)  [unwired: 1 in, 3 out]
              n468 = Fract/Exp String To Number(string=w1430) -> (number=w1434:dbl)  [unwired: 3 in, 1 out]
              n469 = Bundle By Name(cluster=w1435, "Nimages"=w1434) -> (w1433:refnum<class "Channel.lvclass">)
            }
          }
          n470 = Increment(x=w1425) -> (x+1=w1416:i32)
        }
        frame 104 {
          w1443 = "INITIAL_LINE "
          n471 = Unbundle By Name(w1437) -> ("lastStatus"=w1438:string)
          n472 = Match Pattern(string=w1438, regular expression=w1443) -> (match substring=w1442:string, after substring=w1440:string)  [unwired: 1 in, 2 out]
          n473 = Equal?(x=w1442, y=w1443) -> (x = y?=w1446:bool)
          n474 = case shown="True" w1446 {
            tunnel: [w1447 w1449] -> w1445
            tunnel: w1444 -> [w1447 w1449]
            tunnel: w1437 -> [w1448 w1455]
            tunnel: [w1448 w1453] -> w1441
            tunnel: w1440 -> [_ w1451]
            frame False {
            }
            frame True {
              n475 = call <vilib>:"Space Constant.vi"() -> ("String"=w1452:string)
              n476 = Match Pattern(string=w1451, regular expression=w1452) -> (before substring=w1450:string)  [unwired: 1 in, 3 out]
              n477 = Fract/Exp String To Number(string=w1450) -> (number=w1454:dbl)  [unwired: 3 in, 1 out]
              n478 = Bundle By Name(cluster=w1455, "InitialLine"=w1454) -> (w1453:refnum<class "Channel.lvclass">)
            }
          }
          n479 = Increment(x=w1445) -> (x+1=w1436:i32)
        }
        frame 105 {
          w1463 = "FINAL_LINE "
          n480 = Unbundle By Name(w1457) -> ("lastStatus"=w1458:string)
          n481 = Match Pattern(string=w1458, regular expression=w1463) -> (match substring=w1462:string, after substring=w1460:string)  [unwired: 1 in, 2 out]
          n482 = Equal?(x=w1462, y=w1463) -> (x = y?=w1466:bool)
          n483 = case shown="True" w1466 {
            tunnel: [w1467 w1469] -> w1465
            tunnel: w1464 -> [w1467 w1469]
            tunnel: w1457 -> [w1468 w1475]
            tunnel: [w1468 w1473] -> w1461
            tunnel: w1460 -> [_ w1471]
            frame False {
            }
            frame True {
              n484 = call <vilib>:"Space Constant.vi"() -> ("String"=w1472:string)
              n485 = Match Pattern(string=w1471, regular expression=w1472) -> (before substring=w1470:string)  [unwired: 1 in, 3 out]
              n486 = Fract/Exp String To Number(string=w1470) -> (number=w1474:dbl)  [unwired: 3 in, 1 out]
              n487 = Bundle By Name(cluster=w1475, "FinalLine"=w1474) -> (w1473:refnum<class "Channel.lvclass">)
            }
          }
          n488 = Increment(x=w1465) -> (x+1=w1456:i32)
        }
        frame 106 {
          w1483 = "INITIAL_COLUMN "
          n489 = Unbundle By Name(w1477) -> ("lastStatus"=w1478:string)
          n490 = Match Pattern(string=w1478, regular expression=w1483) -> (match substring=w1482:string, after substring=w1480:string)  [unwired: 1 in, 2 out]
          n491 = Equal?(x=w1482, y=w1483) -> (x = y?=w1486:bool)
          n492 = case shown="True" w1486 {
            tunnel: [w1487 w1489] -> w1485
            tunnel: w1484 -> [w1487 w1489]
            tunnel: w1477 -> [w1488 w1495]
            tunnel: [w1488 w1493] -> w1481
            tunnel: w1480 -> [_ w1491]
            frame False {
            }
            frame True {
              n493 = call <vilib>:"Space Constant.vi"() -> ("String"=w1492:string)
              n494 = Match Pattern(string=w1491, regular expression=w1492) -> (before substring=w1490:string)  [unwired: 1 in, 3 out]
              n495 = Fract/Exp String To Number(string=w1490) -> (number=w1494:dbl)  [unwired: 3 in, 1 out]
              n496 = Bundle By Name(cluster=w1495, "InitialColumn"=w1494) -> (w1493:refnum<class "Channel.lvclass">)
            }
          }
          n497 = Increment(x=w1485) -> (x+1=w1476:i32)
        }
        frame 107 {
          w1503 = "FINAL_COLUMN "
          n498 = Unbundle By Name(w1497) -> ("lastStatus"=w1498:string)
          n499 = Match Pattern(string=w1498, regular expression=w1503) -> (match substring=w1502:string, after substring=w1500:string)  [unwired: 1 in, 2 out]
          n500 = Equal?(x=w1502, y=w1503) -> (x = y?=w1506:bool)
          n501 = case shown="True" w1506 {
            tunnel: [w1507 w1509] -> w1505
            tunnel: w1504 -> [w1507 w1509]
            tunnel: w1497 -> [w1508 w1515]
            tunnel: [w1508 w1513] -> w1501
            tunnel: w1500 -> [_ w1511]
            frame False {
            }
            frame True {
              n502 = call <vilib>:"Space Constant.vi"() -> ("String"=w1512:string)
              n503 = Match Pattern(string=w1511, regular expression=w1512) -> (before substring=w1510:string)  [unwired: 1 in, 3 out]
              n504 = Fract/Exp String To Number(string=w1510) -> (number=w1514:dbl)  [unwired: 3 in, 1 out]
              n505 = Bundle By Name(cluster=w1515, "FinalColumn"=w1514) -> (w1513:refnum<class "Channel.lvclass">)
            }
          }
          n506 = Increment(x=w1505) -> (x+1=w1496:i32)
        }
        frame 108 {
          w1523 = "EM_GAIN "
          n507 = Unbundle By Name(w1517) -> ("lastStatus"=w1518:string)
          n508 = Match Pattern(string=w1518, regular expression=w1523) -> (match substring=w1522:string, after substring=w1520:string)  [unwired: 1 in, 2 out]
          n509 = Equal?(x=w1522, y=w1523) -> (x = y?=w1526:bool)
          n510 = case shown="True" w1526 {
            tunnel: [w1527 w1529] -> w1525
            tunnel: w1524 -> [w1527 w1529]
            tunnel: w1517 -> [w1528 w1535]
            tunnel: [w1528 w1533] -> w1521
            tunnel: w1520 -> [_ w1531]
            frame False {
            }
            frame True {
              n511 = call <vilib>:"Space Constant.vi"() -> ("String"=w1532:string)
              n512 = Match Pattern(string=w1531, regular expression=w1532) -> (before substring=w1530:string)  [unwired: 1 in, 3 out]
              n513 = Fract/Exp String To Number(string=w1530) -> (number=w1534:dbl)  [unwired: 3 in, 1 out]
              n514 = Bundle By Name(cluster=w1535, "EmGain"=w1534) -> (w1533:refnum<class "Channel.lvclass">)
            }
          }
          n515 = Increment(x=w1525) -> (x+1=w1516:i32)
        }
        frame 109 {
          w1543 = "COOLER "
          n516 = Unbundle By Name(w1537) -> ("lastStatus"=w1538:string)
          n517 = Match Pattern(string=w1538, regular expression=w1543) -> (match substring=w1542:string, after substring=w1540:string)  [unwired: 1 in, 2 out]
          n518 = Equal?(x=w1542, y=w1543) -> (x = y?=w1546:bool)
          n519 = case shown="True" w1546 {
            tunnel: [w1547 w1549] -> w1545
            tunnel: w1544 -> [w1547 w1549]
            tunnel: w1537 -> [w1548 w1556]
            tunnel: [w1548 w1555] -> w1541
            tunnel: w1540 -> [_ w1553]
            frame False {
            }
            frame True {
              n520 = call <vilib>:"Space Constant.vi"() -> ("String"=w1554:string)
              n521 = Match Pattern(string=w1553, regular expression=w1554) -> (before substring=w1552:string)  [unwired: 1 in, 3 out]
              n522 = Equal?(x=w1552, y="ON") -> (x = y?=w1550:bool)
              n523 = Bundle By Name(cluster=w1556, "Cooler Off"=w1550) -> (w1555:refnum<class "Channel.lvclass">)
            }
          }
          n524 = Increment(x=w1545) -> (x+1=w1536:i32)
        }
        frame 110 {
        }
        frame 200 {
          n525 = Unbundle By Name(w1568) -> ("Interface.lvclass"=w1567:refnum<class "Interface.lvclass">)
          n526 = call "Read Camera Setup.vi"("Interface in"=w1567) -> ("Camera Setup"=w1561:T4)  [unwired: 8 in, 2 out]
          n527 = Unbundle By Name(w1561) -> ("EXPTIME"=w1560:dbl)
          n528 = Number To Fractional String(number=w1560) -> (F-format string=w1562:string)  [unwired: 3 in]
          n529 = Concatenate Strings("SET EXPTIME " ("cmd"), w1562) -> (w1566:string)
          n530 = call-dynamic "Write cmd.vi"("error in (no error)"=w1570, "cmd"=w1566, "Device in"=w1568) -> ("error out"=w1569:errorcluster, "Device out"=w1571:refnum<class "Channel.lvclass">)  [unwired: 7 in]
          n531 = Increment(x=w1564) -> (x+1=w1565:i32)
        }
        frame 201 {
          n532 = call-dynamic "Read resp.vi"("error in (no error)"=w1579, "Device in"=w1580) -> ("error out"=w1573:errorcluster, "resp"=w1578:string, "Device out"=w1574:refnum<class "Channel.lvclass">)  [unwired: 7 in]
          n533 = Equal?(x=w1578, y="DONE") -> (x = y?=w1576:bool)
          n534 = case shown="True" w1576 {
            tunnel: [w1581 w1582] -> w1575
            tunnel: w1572 -> [w1581 w1583]
            frame False {
            }
            frame True {
              n535 = Increment(x=w1583) -> (x+1=w1582:i32)
            }
          }
        }
        frame 202 {
          n536 = call-dynamic "Write cmd.vi"("error in (no error)"=w1589, "cmd"="GET EXPTIME", "Device in"=w1587) -> ("error out"=w1588:errorcluster, "Device out"=w1590:refnum<class "Channel.lvclass">)  [unwired: 7 in]
          n537 = Increment(x=w1585) -> (x+1=w1586:i32)
        }
        frame 203 {
          n538 = call-dynamic "Read resp.vi"("error in (no error)"=w1601, "Device in"=w1602) -> ("error out"=w1599:errorcluster, "resp"=w1594:string, "Device out"=w1597:refnum<class "Channel.lvclass">)  [unwired: 7 in]
          n539 = Fract/Exp String To Number(string=w1594) -> (number=w1591:dbl)  [unwired: 3 in, 1 out]
          n540 = Unbundle By Name(w1597) -> ("Interface.lvclass"=w1596:refnum<class "Interface.lvclass">)
          n541 = call "Read Camera Setup.vi"("Interface in"=w1596) -> ("Camera Setup"=w1595:T4)  [unwired: 8 in, 2 out]
          n542 = Unbundle By Name(w1595) -> ("EXPTIME"=w1592:dbl)
          n543 = Equal?(x=w1592, y=w1591) -> (x = y?=w1593:bool)
          n544 = disable-structure shown="Enabled" {
            disable-tunnel: [w1605 224 ("State")] -> w1600
            disable-tunnel: w1598 -> [w1604 _]
            disable-tunnel: w1593 -> [w1603 _]
            frame Disabled {
              n545 = case shown="True" w1603 {
                tunnel: [w1606 w1607] -> w1605
                tunnel: w1604 -> [w1606 w1608]
                frame False {
                }
                frame True {
                  n546 = Increment(x=w1608) -> (x+1=w1607:i32)
                }
              }
            }
            frame Enabled {
            }
          }
        }
        frame 204 {
          n547 = Unbundle By Name(w1618) -> ("Interface.lvclass"=w1617:refnum<class "Interface.lvclass">)
          n548 = call "Read Camera Setup.vi"("Interface in"=w1617) -> ("Camera Setup"=w1611:T4)  [unwired: 8 in, 2 out]
          n549 = Unbundle By Name(w1611) -> ("#FRAMES"=w1610:u32)
          n550 = Number To Fractional String(number=w1610) -> (F-format string=w1612:string)  [unwired: 3 in]
          n551 = Concatenate Strings("SET #FRAMES " ("cmd"), w1612) -> (w1616:string)
          n552 = call-dynamic "Write cmd.vi"("error in (no error)"=w1620, "cmd"=w1616, "Device in"=w1618) -> ("error out"=w1619:errorcluster, "Device out"=w1621:refnum<class "Channel.lvclass">)  [unwired: 7 in]
          n553 = Increment(x=w1614) -> (x+1=w1615:i32)
        }
        frame 205 {
          n554 = call-dynamic "Read resp.vi"("error in (no error)"=w1629, "Device in"=w1630) -> ("error out"=w1623:errorcluster, "resp"=w1628:string, "Device out"=w1624:refnum<class "Channel.lvclass">)  [unwired: 7 in]
          n555 = Equal?(x=w1628, y="DONE") -> (x = y?=w1626:bool)
          n556 = case shown="True" w1626 {
            tunnel: [w1631 w1632] -> w1625
            tunnel: w1622 -> [w1631 w1633]
            frame False {
            }
            frame True {
              n557 = Increment(x=w1633) -> (x+1=w1632:i32)
            }
          }
        }
        frame 206 {
          n558 = call-dynamic "Write cmd.vi"("error in (no error)"=w1639, "cmd"="GET #FRAMES", "Device in"=w1637) -> ("error out"=w1638:errorcluster, "Device out"=w1640:refnum<class "Channel.lvclass">)  [unwired: 7 in]
          n559 = Increment(x=w1635) -> (x+1=w1636:i32)
        }
        frame 207 {
          n560 = call-dynamic "Read resp.vi"("error in (no error)"=w1652, "Device in"=w1653) -> ("error out"=w1650:errorcluster, "resp"=w1645:string, "Device out"=w1648:refnum<class "Channel.lvclass">)  [unwired: 7 in]
          n561 = Decimal String To Number(string=w1645) -> (number=w1643:i32)  [unwired: 2 in, 1 out]
          n562 = Unbundle By Name(w1648) -> ("Interface.lvclass"=w1647:refnum<class "Interface.lvclass">)
          n563 = call "Read Camera Setup.vi"("Interface in"=w1647) -> ("Camera Setup"=w1646:T4)  [unwired: 8 in, 2 out]
          n564 = To Unsigned Long Integer(number=w1643) -> (unsigned 32bit integer=w1641:u32)
          n565 = Unbundle By Name(w1646) -> ("#FRAMES"=w1642:u32)
          n566 = Equal?(x=w1642, y=w1641) -> (x = y?=w1644:bool)
          n567 = case shown="True" w1644 {
            tunnel: [w1654 w1655] -> w1651
            tunnel: w1649 -> [w1654 w1656]
            frame False {
            }
            frame True {
              n568 = Increment(x=w1656) -> (x+1=w1655:i32)
            }
          }
        }
        frame 208 {
          n569 = Unbundle By Name(w1665) -> ("Interface.lvclass"=w1664:refnum<class "Interface.lvclass">)
          n570 = call "Read Camera Setup.vi"("Interface in"=w1664) -> ("Camera Setup"=w1658:T4)  [unwired: 8 in, 2 out]
          n571 = Unbundle By Name(w1658) -> ("TRIGGER_MODE"=w1657:u8)
          n572 = Number To Fractional String(number=w1657) -> (F-format string=w1659:string)  [unwired: 3 in]
          n573 = Concatenate Strings("SET TRIGGER_MODE " ("cmd"), w1659) -> (w1663:string)
          n574 = call-dynamic "Write cmd.vi"("error in (no error)"=w1667, "cmd"=w1663, "Device in"=w1665) -> ("error out"=w1666:errorcluster, "Device out"=w1668:refnum<class "Channel.lvclass">)  [unwired: 7 in]
          n575 = Increment(x=w1661) -> (x+1=w1662:i32)
        }
        frame 209 {
          n576 = call-dynamic "Read resp.vi"("error in (no error)"=w1676, "Device in"=w1677) -> ("error out"=w1670:errorcluster, "resp"=w1675:string, "Device out"=w1671:refnum<class "Channel.lvclass">)  [unwired: 7 in]
          n577 = Equal?(x=w1675, y="DONE") -> (x = y?=w1673:bool)
          n578 = case shown="True" w1673 {
            tunnel: [w1678 w1679] -> w1672
            tunnel: w1669 -> [w1678 w1680]
            frame False {
            }
            frame True {
              n579 = Increment(x=w1680) -> (x+1=w1679:i32)
            }
          }
        }
        frame 210 {
          n580 = call-dynamic "Write cmd.vi"("error in (no error)"=w1686, "cmd"="GET TRIGGER_MODE", "Device in"=w1684) -> ("error out"=w1685:errorcluster, "Device out"=w1687:refnum<class "Channel.lvclass">)  [unwired: 7 in]
          n581 = Increment(x=w1682) -> (x+1=w1683:i32)
        }
        frame 211 {
          n582 = call-dynamic "Read resp.vi"("error in (no error)"=w1698, "Device in"=w1699) -> ("error out"=w1696:errorcluster, "resp"=w1691:string, "Device out"=w1694:refnum<class "Channel.lvclass">)  [unwired: 7 in]
          n583 = Fract/Exp String To Number(string=w1691) -> (number=w1689:dbl)  [unwired: 3 in, 1 out]
          n584 = Unbundle By Name(w1694) -> ("Interface.lvclass"=w1693:refnum<class "Interface.lvclass">)
          n585 = call "Read Camera Setup.vi"("Interface in"=w1693) -> ("Camera Setup"=w1692:T4)  [unwired: 8 in, 2 out]
          n586 = Unbundle By Name(w1692) -> ("TRIGGER_MODE"=w1688:u8)
          n587 = Equal?(x=w1688, y=w1689) -> (x = y?=w1690:bool)
          n588 = case shown="False" w1690 {
            tunnel: [w1700 w1701] -> w1697
            tunnel: w1695 -> [w1700 w1702]
            frame False {
            }
            frame True {
              n589 = Increment(x=w1702) -> (x+1=w1701:i32)
            }
          }
        }
        frame 212 {
          n590 = Unbundle By Name(w1711) -> ("Interface.lvclass"=w1710:refnum<class "Interface.lvclass">)
          n591 = call "Read Camera Setup.vi"("Interface in"=w1710) -> ("Camera Setup"=w1704:T4)  [unwired: 8 in, 2 out]
          n592 = Unbundle By Name(w1704) -> ("READ_MODE"=w1703:u8)
          n593 = Number To Fractional String(number=w1703) -> (F-format string=w1705:string)  [unwired: 3 in]
          n594 = Concatenate Strings("SET READ_MODE " ("cmd"), w1705) -> (w1709:string)
          n595 = call-dynamic "Write cmd.vi"("error in (no error)"=w1713, "cmd"=w1709, "Device in"=w1711) -> ("error out"=w1712:errorcluster, "Device out"=w1714:refnum<class "Channel.lvclass">)  [unwired: 7 in]
          n596 = Increment(x=w1707) -> (x+1=w1708:i32)
        }
        frame 213 {
          n597 = call-dynamic "Read resp.vi"("error in (no error)"=w1722, "Device in"=w1723) -> ("error out"=w1716:errorcluster, "resp"=w1721:string, "Device out"=w1717:refnum<class "Channel.lvclass">)  [unwired: 7 in]
          n598 = Equal?(x=w1721, y="DONE") -> (x = y?=w1719:bool)
          n599 = case shown="True" w1719 {
            tunnel: [w1724 w1725] -> w1718
            tunnel: w1715 -> [w1724 w1726]
            frame False {
            }
            frame True {
              n600 = Increment(x=w1726) -> (x+1=w1725:i32)
            }
          }
        }
        frame 214 {
          n601 = call-dynamic "Write cmd.vi"("error in (no error)"=w1732, "cmd"="GET READ_MODE", "Device in"=w1730) -> ("error out"=w1731:errorcluster, "Device out"=w1733:refnum<class "Channel.lvclass">)  [unwired: 7 in]
          n602 = Increment(x=w1728) -> (x+1=w1729:i32)
        }
        frame 215 {
          n603 = call-dynamic "Read resp.vi"("error in (no error)"=w1744, "Device in"=w1745) -> ("error out"=w1742:errorcluster, "resp"=w1737:string, "Device out"=w1740:refnum<class "Channel.lvclass">)  [unwired: 7 in]
          n604 = Fract/Exp String To Number(string=w1737) -> (number=w1735:dbl)  [unwired: 3 in, 1 out]
          n605 = Unbundle By Name(w1740) -> ("Interface.lvclass"=w1739:refnum<class "Interface.lvclass">)
          n606 = call "Read Camera Setup.vi"("Interface in"=w1739) -> ("Camera Setup"=w1738:T4)  [unwired: 8 in, 2 out]
          n607 = Unbundle By Name(w1738) -> ("READ_MODE"=w1734:u8)
          n608 = Equal?(x=w1734, y=w1735) -> (x = y?=w1736:bool)
          n609 = case shown="True" w1736 {
            tunnel: [w1746 w1747] -> w1743
            tunnel: w1741 -> [w1746 w1748]
            frame False {
            }
            frame True {
              n610 = Increment(x=w1748) -> (x+1=w1747:i32)
            }
          }
        }
        frame 216 {
          n611 = Unbundle By Name(w1757) -> ("Interface.lvclass"=w1756:refnum<class "Interface.lvclass">)
          n612 = call "Read Camera Setup.vi"("Interface in"=w1756) -> ("Camera Setup"=w1750:T4)  [unwired: 8 in, 2 out]
          n613 = Unbundle By Name(w1750) -> ("READOUT_RATE"=w1749:u8)
          n614 = Number To Fractional String(number=w1749) -> (F-format string=w1751:string)  [unwired: 3 in]
          n615 = Concatenate Strings("SET READOUT_RATE " ("cmd"), w1751) -> (w1755:string)
          n616 = call-dynamic "Write cmd.vi"("error in (no error)"=w1759, "cmd"=w1755, "Device in"=w1757) -> ("error out"=w1758:errorcluster, "Device out"=w1760:refnum<class "Channel.lvclass">)  [unwired: 7 in]
          n617 = Increment(x=w1753) -> (x+1=w1754:i32)
        }
        frame 217 {
          n618 = call-dynamic "Read resp.vi"("error in (no error)"=w1768, "Device in"=w1769) -> ("error out"=w1762:errorcluster, "resp"=w1767:string, "Device out"=w1763:refnum<class "Channel.lvclass">)  [unwired: 7 in]
          n619 = Equal?(x=w1767, y="DONE") -> (x = y?=w1765:bool)
          n620 = case shown="True" w1765 {
            tunnel: [w1770 w1771] -> w1764
            tunnel: w1761 -> [w1770 w1772]
            frame False {
            }
            frame True {
              n621 = Increment(x=w1772) -> (x+1=w1771:i32)
            }
          }
        }
        frame 218 {
          n622 = call-dynamic "Write cmd.vi"("error in (no error)"=w1778, "cmd"="GET READOUT_RATE", "Device in"=w1776) -> ("error out"=w1777:errorcluster, "Device out"=w1779:refnum<class "Channel.lvclass">)  [unwired: 7 in]
          n623 = Increment(x=w1774) -> (x+1=w1775:i32)
        }
        frame 219 {
          n624 = call-dynamic "Read resp.vi"("error in (no error)"=w1790, "Device in"=w1791) -> ("error out"=w1788:errorcluster, "resp"=w1783:string, "Device out"=w1786:refnum<class "Channel.lvclass">)  [unwired: 7 in]
          n625 = Fract/Exp String To Number(string=w1783) -> (number=w1781:dbl)  [unwired: 3 in, 1 out]
          n626 = Unbundle By Name(w1786) -> ("Interface.lvclass"=w1785:refnum<class "Interface.lvclass">)
          n627 = call "Read Camera Setup.vi"("Interface in"=w1785) -> ("Camera Setup"=w1784:T4)  [unwired: 8 in, 2 out]
          n628 = Unbundle By Name(w1784) -> ("READOUT_RATE"=w1780:u8)
          n629 = Equal?(x=w1780, y=w1781) -> (x = y?=w1782:bool)
          n630 = case shown="True" w1782 {
            tunnel: [w1792 w1793] -> w1789
            tunnel: w1787 -> [w1792 w1794]
            frame False {
            }
            frame True {
              n631 = Increment(x=w1794) -> (x+1=w1793:i32)
            }
          }
        }
        frame 220 {
          n632 = Unbundle By Name(w1803) -> ("Interface.lvclass"=w1802:refnum<class "Interface.lvclass">)
          n633 = call "Read Camera Setup.vi"("Interface in"=w1802) -> ("Camera Setup"=w1796:T4)  [unwired: 8 in, 2 out]
          n634 = Unbundle By Name(w1796) -> ("VERTICAL_SHIFT_SPEED"=w1795:u8)
          n635 = Number To Fractional String(number=w1795) -> (F-format string=w1797:string)  [unwired: 3 in]
          n636 = Concatenate Strings("SET VERTICAL_SHIFT_SPEED " ("cmd"), w1797) -> (w1801:string)
          n637 = call-dynamic "Write cmd.vi"("error in (no error)"=w1805, "cmd"=w1801, "Device in"=w1803) -> ("error out"=w1804:errorcluster, "Device out"=w1806:refnum<class "Channel.lvclass">)  [unwired: 7 in]
          n638 = Increment(x=w1799) -> (x+1=w1800:i32)
        }
        frame 221 {
          n639 = call-dynamic "Read resp.vi"("error in (no error)"=w1814, "Device in"=w1815) -> ("error out"=w1808:errorcluster, "resp"=w1813:string, "Device out"=w1809:refnum<class "Channel.lvclass">)  [unwired: 7 in]
          n640 = Equal?(x=w1813, y="DONE") -> (x = y?=w1811:bool)
          n641 = case shown="True" w1811 {
            tunnel: [w1816 w1817] -> w1810
            tunnel: w1807 -> [w1816 w1818]
            frame False {
            }
            frame True {
              n642 = Increment(x=w1818) -> (x+1=w1817:i32)
            }
          }
        }
        frame 222 {
          n643 = call-dynamic "Write cmd.vi"("error in (no error)"=w1824, "cmd"="GET VERTICAL_SHIFT_SPEED", "Device in"=w1822) -> ("error out"=w1823:errorcluster, "Device out"=w1825:refnum<class "Channel.lvclass">)  [unwired: 7 in]
          n644 = Increment(x=w1820) -> (x+1=w1821:i32)
        }
        frame 223 {
          n645 = call-dynamic "Read resp.vi"("error in (no error)"=w1836, "Device in"=w1837) -> ("error out"=w1834:errorcluster, "resp"=w1829:string, "Device out"=w1832:refnum<class "Channel.lvclass">)  [unwired: 7 in]
          n646 = Fract/Exp String To Number(string=w1829) -> (number=w1827:dbl)  [unwired: 3 in, 1 out]
          n647 = Unbundle By Name(w1832) -> ("Interface.lvclass"=w1831:refnum<class "Interface.lvclass">)
          n648 = call "Read Camera Setup.vi"("Interface in"=w1831) -> ("Camera Setup"=w1830:T4)  [unwired: 8 in, 2 out]
          n649 = Unbundle By Name(w1830) -> ("VERTICAL_SHIFT_SPEED"=w1826:u8)
          n650 = Equal?(x=w1826, y=w1827) -> (x = y?=w1828:bool)
          n651 = case shown="True" w1828 {
            tunnel: [w1838 w1839] -> w1835
            tunnel: w1833 -> [w1838 w1840]
            frame False {
            }
            frame True {
              n652 = Increment(x=w1840) -> (x+1=w1839:i32)
            }
          }
        }
        frame 224 {
          n653 = Unbundle By Name(w1849) -> ("Interface.lvclass"=w1848:refnum<class "Interface.lvclass">)
          n654 = call "Read Camera Setup.vi"("Interface in"=w1848) -> ("Camera Setup"=w1842:T4)  [unwired: 8 in, 2 out]
          n655 = Unbundle By Name(w1842) -> ("PREAMP"=w1841:u8)
          n656 = Number To Fractional String(number=w1841) -> (F-format string=w1843:string)  [unwired: 3 in]
          n657 = Concatenate Strings("SET PREAMP " ("cmd"), w1843) -> (w1847:string)
          n658 = call-dynamic "Write cmd.vi"("error in (no error)"=w1851, "cmd"=w1847, "Device in"=w1849) -> ("error out"=w1850:errorcluster, "Device out"=w1852:refnum<class "Channel.lvclass">)  [unwired: 7 in]
          n659 = Increment(x=w1845) -> (x+1=w1846:i32)
        }
        frame 225 {
          n660 = call-dynamic "Read resp.vi"("error in (no error)"=w1860, "Device in"=w1861) -> ("error out"=w1854:errorcluster, "resp"=w1859:string, "Device out"=w1855:refnum<class "Channel.lvclass">)  [unwired: 7 in]
          n661 = Equal?(x=w1859, y="DONE") -> (x = y?=w1857:bool)
          n662 = case shown="True" w1857 {
            tunnel: [w1862 w1863] -> w1856
            tunnel: w1853 -> [w1862 w1864]
            frame False {
            }
            frame True {
              n663 = Increment(x=w1864) -> (x+1=w1863:i32)
            }
          }
        }
        frame 226 {
          n664 = call-dynamic "Write cmd.vi"("error in (no error)"=w1870, "cmd"="GET PREAMP", "Device in"=w1868) -> ("error out"=w1869:errorcluster, "Device out"=w1871:refnum<class "Channel.lvclass">)  [unwired: 7 in]
          n665 = Increment(x=w1866) -> (x+1=w1867:i32)
        }
        frame 227 {
          n666 = call-dynamic "Read resp.vi"("error in (no error)"=w1882, "Device in"=w1883) -> ("error out"=w1880:errorcluster, "resp"=w1875:string, "Device out"=w1878:refnum<class "Channel.lvclass">)  [unwired: 7 in]
          n667 = Fract/Exp String To Number(string=w1875) -> (number=w1873:dbl)  [unwired: 3 in, 1 out]
          n668 = Unbundle By Name(w1878) -> ("Interface.lvclass"=w1877:refnum<class "Interface.lvclass">)
          n669 = call "Read Camera Setup.vi"("Interface in"=w1877) -> ("Camera Setup"=w1876:T4)  [unwired: 8 in, 2 out]
          n670 = Unbundle By Name(w1876) -> ("PREAMP"=w1872:u8)
          n671 = Equal?(x=w1872, y=w1873) -> (x = y?=w1874:bool)
          n672 = case shown="True" w1874 {
            tunnel: [w1884 w1885] -> w1881
            tunnel: w1879 -> [w1884 w1886]
            frame False {
            }
            frame True {
              n673 = Increment(x=w1886) -> (x+1=w1885:i32)
            }
          }
        }
        frame 228 {
          n674 = Unbundle By Name(w1895) -> ("Interface.lvclass"=w1894:refnum<class "Interface.lvclass">)
          n675 = call "Read Camera Setup.vi"("Interface in"=w1894) -> ("Camera Setup"=w1888:T4)  [unwired: 8 in, 2 out]
          n676 = Unbundle By Name(w1888) -> ("EM_MODE"=w1887:u8)
          n677 = Number To Fractional String(number=w1887) -> (F-format string=w1889:string)  [unwired: 3 in]
          n678 = Concatenate Strings("SET EM_MODE " ("cmd"), w1889) -> (w1893:string)
          n679 = call-dynamic "Write cmd.vi"("error in (no error)"=w1897, "cmd"=w1893, "Device in"=w1895) -> ("error out"=w1896:errorcluster, "Device out"=w1898:refnum<class "Channel.lvclass">)  [unwired: 7 in]
          n680 = Increment(x=w1891) -> (x+1=w1892:i32)
        }
        frame 229 {
          n681 = call-dynamic "Read resp.vi"("error in (no error)"=w1906, "Device in"=w1907) -> ("error out"=w1900:errorcluster, "resp"=w1905:string, "Device out"=w1901:refnum<class "Channel.lvclass">)  [unwired: 7 in]
          n682 = Equal?(x=w1905, y="DONE") -> (x = y?=w1903:bool)
          n683 = case shown="True" w1903 {
            tunnel: [w1908 w1909] -> w1902
            tunnel: w1899 -> [w1908 w1910]
            frame False {
            }
            frame True {
              n684 = Increment(x=w1910) -> (x+1=w1909:i32)
            }
          }
        }
        frame 230 {
          n685 = call-dynamic "Write cmd.vi"("error in (no error)"=w1916, "cmd"="GET EM_MODE", "Device in"=w1914) -> ("error out"=w1915:errorcluster, "Device out"=w1917:refnum<class "Channel.lvclass">)  [unwired: 7 in]
          n686 = Increment(x=w1912) -> (x+1=w1913:i32)
        }
        frame 231 {
          n687 = call-dynamic "Read resp.vi"("error in (no error)"=w1928, "Device in"=w1929) -> ("error out"=w1926:errorcluster, "resp"=w1921:string, "Device out"=w1924:refnum<class "Channel.lvclass">)  [unwired: 7 in]
          n688 = Fract/Exp String To Number(string=w1921) -> (number=w1919:dbl)  [unwired: 3 in, 1 out]
          n689 = Unbundle By Name(w1924) -> ("Interface.lvclass"=w1923:refnum<class "Interface.lvclass">)
          n690 = call "Read Camera Setup.vi"("Interface in"=w1923) -> ("Camera Setup"=w1922:T4)  [unwired: 8 in, 2 out]
          n691 = Unbundle By Name(w1922) -> ("EM_MODE"=w1918:u8)
          n692 = Equal?(x=w1918, y=w1919) -> (x = y?=w1920:bool)
          n693 = case shown="True" w1920 {
            tunnel: [w1930 w1931] -> w1927
            tunnel: w1925 -> [w1930 w1932]
            frame False {
            }
            frame True {
              n694 = Increment(x=w1932) -> (x+1=w1931:i32)
            }
          }
        }
        frame 232 {
          n695 = Unbundle By Name(w1941) -> ("Interface.lvclass"=w1940:refnum<class "Interface.lvclass">)
          n696 = call "Read Camera Setup.vi"("Interface in"=w1940) -> ("Camera Setup"=w1934:T4)  [unwired: 8 in, 2 out]
          n697 = Unbundle By Name(w1934) -> ("EM_GAIN"=w1933:u16)
          n698 = Number To Fractional String(number=w1933) -> (F-format string=w1935:string)  [unwired: 3 in]
          n699 = Concatenate Strings("SET EM_GAIN " ("cmd"), w1935) -> (w1939:string)
          n700 = call-dynamic "Write cmd.vi"("error in (no error)"=w1943, "cmd"=w1939, "Device in"=w1941) -> ("error out"=w1942:errorcluster, "Device out"=w1944:refnum<class "Channel.lvclass">)  [unwired: 7 in]
          n701 = Increment(x=w1937) -> (x+1=w1938:i32)
        }
        frame 233 {
          n702 = call-dynamic "Read resp.vi"("error in (no error)"=w1952, "Device in"=w1953) -> ("error out"=w1946:errorcluster, "resp"=w1951:string, "Device out"=w1947:refnum<class "Channel.lvclass">)  [unwired: 7 in]
          n703 = Equal?(x=w1951, y="DONE") -> (x = y?=w1949:bool)
          n704 = case shown="True" w1949 {
            tunnel: [w1954 w1955] -> w1948
            tunnel: w1945 -> [w1954 w1956]
            frame False {
            }
            frame True {
              n705 = Increment(x=w1956) -> (x+1=w1955:i32)
            }
          }
        }
        frame 234 {
          n706 = call-dynamic "Write cmd.vi"("error in (no error)"=w1962, "cmd"="GET EM_GAIN", "Device in"=w1960) -> ("error out"=w1961:errorcluster, "Device out"=w1963:refnum<class "Channel.lvclass">)  [unwired: 7 in]
          n707 = Increment(x=w1958) -> (x+1=w1959:i32)
        }
        frame 235 {
          n708 = call-dynamic "Read resp.vi"("error in (no error)"=w1974, "Device in"=w1975) -> ("error out"=w1972:errorcluster, "resp"=w1967:string, "Device out"=w1970:refnum<class "Channel.lvclass">)  [unwired: 7 in]
          n709 = Fract/Exp String To Number(string=w1967) -> (number=w1965:dbl)  [unwired: 3 in, 1 out]
          n710 = Unbundle By Name(w1970) -> ("Interface.lvclass"=w1969:refnum<class "Interface.lvclass">)
          n711 = call "Read Camera Setup.vi"("Interface in"=w1969) -> ("Camera Setup"=w1968:T4)  [unwired: 8 in, 2 out]
          n712 = Unbundle By Name(w1968) -> ("EM_GAIN"=w1964:u16)
          n713 = Equal?(x=w1964, y=w1965) -> (x = y?=w1966:bool)
          n714 = disable-structure shown="Enabled" {
            disable-tunnel: [w1978 264 ("State")] -> w1973
            disable-tunnel: w1971 -> [w1977 _]
            disable-tunnel: w1966 -> [w1976 _]
            frame Disabled {
              n715 = case shown="True" w1976 {
                tunnel: [w1979 w1980] -> w1978
                tunnel: w1977 -> [w1979 w1981]
                frame False {
                }
                frame True {
                  n716 = Increment(x=w1981) -> (x+1=w1980:i32)
                }
              }
            }
            frame Enabled {
            }
          }
        }
        frame 236 {
          n717 = Unbundle By Name(w1991) -> ("Interface.lvclass"=w1990:refnum<class "Interface.lvclass">)
          n718 = call "Read Camera Setup.vi"("Interface in"=w1990) -> ("Camera Setup"=w1984:T4)  [unwired: 8 in, 2 out]
          n719 = Unbundle By Name(w1984) -> ("ACQUISITION_MODE"=w1983:u8)
          n720 = Number To Fractional String(number=w1983) -> (F-format string=w1985:string)  [unwired: 3 in]
          n721 = Concatenate Strings("SET ACQUISITION_MODE " ("cmd"), w1985) -> (w1989:string)
          n722 = call-dynamic "Write cmd.vi"("error in (no error)"=w1993, "cmd"=w1989, "Device in"=w1991) -> ("error out"=w1992:errorcluster, "Device out"=w1994:refnum<class "Channel.lvclass">)  [unwired: 7 in]
          n723 = Increment(x=w1987) -> (x+1=w1988:i32)
        }
        frame 237 {
          n724 = call-dynamic "Read resp.vi"("error in (no error)"=w2002, "Device in"=w2003) -> ("error out"=w1996:errorcluster, "resp"=w2001:string, "Device out"=w1997:refnum<class "Channel.lvclass">)  [unwired: 7 in]
          n725 = Equal?(x=w2001, y="DONE") -> (x = y?=w1999:bool)
          n726 = case shown="True" w1999 {
            tunnel: [w2004 w2005] -> w1998
            tunnel: w1995 -> [w2004 w2006]
            frame False {
            }
            frame True {
              n727 = Increment(x=w2006) -> (x+1=w2005:i32)
            }
          }
        }
        frame 238 {
          n728 = call-dynamic "Write cmd.vi"("error in (no error)"=w2012, "cmd"="GET ACQUISITION_MODE", "Device in"=w2010) -> ("error out"=w2011:errorcluster, "Device out"=w2013:refnum<class "Channel.lvclass">)  [unwired: 7 in]
          n729 = Increment(x=w2008) -> (x+1=w2009:i32)
        }
        frame 239 {
          n730 = call-dynamic "Read resp.vi"("error in (no error)"=w2024, "Device in"=w2025) -> ("error out"=w2022:errorcluster, "resp"=w2017:string, "Device out"=w2020:refnum<class "Channel.lvclass">)  [unwired: 7 in]
          n731 = Fract/Exp String To Number(string=w2017) -> (number=w2015:dbl)  [unwired: 3 in, 1 out]
          n732 = Unbundle By Name(w2020) -> ("Interface.lvclass"=w2019:refnum<class "Interface.lvclass">)
          n733 = call "Read Camera Setup.vi"("Interface in"=w2019) -> ("Camera Setup"=w2018:T4)  [unwired: 8 in, 2 out]
          n734 = Unbundle By Name(w2018) -> ("ACQUISITION_MODE"=w2014:u8)
          n735 = Equal?(x=w2014, y=w2015) -> (x = y?=w2016:bool)
          n736 = case shown="True" w2016 {
            tunnel: [w2026 w2027] -> w2023
            tunnel: w2021 -> [w2026 w2028]
            frame False {
            }
            frame True {
              n737 = Increment(x=w2028) -> (x+1=w2027:i32)
            }
          }
        }
        frame 240 {
          n738 = Unbundle By Name(w2037) -> ("Interface.lvclass"=w2036:refnum<class "Interface.lvclass">)
          n739 = call "Read Camera Setup.vi"("Interface in"=w2036) -> ("Camera Setup"=w2030:T4)  [unwired: 8 in, 2 out]
          n740 = Unbundle By Name(w2030) -> ("SHUTTER_MODE"=w2029:u8)
          n741 = Number To Fractional String(number=w2029) -> (F-format string=w2031:string)  [unwired: 3 in]
          n742 = Concatenate Strings("SET SHUTTER_MODE " ("cmd"), w2031) -> (w2035:string)
          n743 = call-dynamic "Write cmd.vi"("error in (no error)"=w2039, "cmd"=w2035, "Device in"=w2037) -> ("error out"=w2038:errorcluster, "Device out"=w2040:refnum<class "Channel.lvclass">)  [unwired: 7 in]
          n744 = Increment(x=w2033) -> (x+1=w2034:i32)
        }
        frame 241 {
          n745 = call-dynamic "Read resp.vi"("error in (no error)"=w2048, "Device in"=w2049) -> ("error out"=w2042:errorcluster, "resp"=w2047:string, "Device out"=w2043:refnum<class "Channel.lvclass">)  [unwired: 7 in]
          n746 = Equal?(x=w2047, y="DONE") -> (x = y?=w2045:bool)
          n747 = case shown="True" w2045 {
            tunnel: [w2050 w2051] -> w2044
            tunnel: w2041 -> [w2050 w2052]
            frame False {
            }
            frame True {
              n748 = Increment(x=w2052) -> (x+1=w2051:i32)
            }
          }
        }
        frame 242 {
          n749 = call-dynamic "Write cmd.vi"("error in (no error)"=w2058, "cmd"="GET SHUTTER_MODE", "Device in"=w2056) -> ("error out"=w2057:errorcluster, "Device out"=w2059:refnum<class "Channel.lvclass">)  [unwired: 7 in]
          n750 = Increment(x=w2054) -> (x+1=w2055:i32)
        }
        frame 243 {
          n751 = call-dynamic "Read resp.vi"("error in (no error)"=w2070, "Device in"=w2071) -> ("error out"=w2068:errorcluster, "resp"=w2063:string, "Device out"=w2066:refnum<class "Channel.lvclass">)  [unwired: 7 in]
          n752 = Fract/Exp String To Number(string=w2063) -> (number=w2061:dbl)  [unwired: 3 in, 1 out]
          n753 = Unbundle By Name(w2066) -> ("Interface.lvclass"=w2065:refnum<class "Interface.lvclass">)
          n754 = call "Read Camera Setup.vi"("Interface in"=w2065) -> ("Camera Setup"=w2064:T4)  [unwired: 8 in, 2 out]
          n755 = Unbundle By Name(w2064) -> ("SHUTTER_MODE"=w2060:u8)
          n756 = Equal?(x=w2060, y=w2061) -> (x = y?=w2062:bool)
          n757 = case shown="True" w2062 {
            tunnel: [w2072 w2073] -> w2069
            tunnel: w2067 -> [w2072 w2074]
            frame False {
            }
            frame True {
              n758 = Increment(x=w2074) -> (x+1=w2073:i32)
            }
          }
        }
        frame 244 {
          n759 = Unbundle By Name(w2083) -> ("Interface.lvclass"=w2082:refnum<class "Interface.lvclass">)
          n760 = call "Read Camera Setup.vi"("Interface in"=w2082) -> ("Camera Setup"=w2076:T4)  [unwired: 8 in, 2 out]
          n761 = Unbundle By Name(w2076) -> ("SHUTTER_TTL"=w2075:u8)
          n762 = Number To Fractional String(number=w2075) -> (F-format string=w2077:string)  [unwired: 3 in]
          n763 = Concatenate Strings("SET SHUTTER_TTL " ("cmd"), w2077) -> (w2081:string)
          n764 = call-dynamic "Write cmd.vi"("error in (no error)"=w2085, "cmd"=w2081, "Device in"=w2083) -> ("error out"=w2084:errorcluster, "Device out"=w2086:refnum<class "Channel.lvclass">)  [unwired: 7 in]
          n765 = Increment(x=w2079) -> (x+1=w2080:i32)
        }
        frame 245 {
          n766 = call-dynamic "Read resp.vi"("error in (no error)"=w2094, "Device in"=w2095) -> ("error out"=w2088:errorcluster, "resp"=w2093:string, "Device out"=w2089:refnum<class "Channel.lvclass">)  [unwired: 7 in]
          n767 = Equal?(x=w2093, y="DONE") -> (x = y?=w2091:bool)
          n768 = case shown="True" w2091 {
            tunnel: [w2096 w2097] -> w2090
            tunnel: w2087 -> [w2096 w2098]
            frame False {
            }
            frame True {
              n769 = Increment(x=w2098) -> (x+1=w2097:i32)
            }
          }
        }
        frame 246 {
          n770 = call-dynamic "Write cmd.vi"("error in (no error)"=w2104, "cmd"="GET SHUTTER_TTL", "Device in"=w2102) -> ("error out"=w2103:errorcluster, "Device out"=w2105:refnum<class "Channel.lvclass">)  [unwired: 7 in]
          n771 = Increment(x=w2100) -> (x+1=w2101:i32)
        }
        frame 247 {
          n772 = call-dynamic "Read resp.vi"("error in (no error)"=w2116, "Device in"=w2117) -> ("error out"=w2114:errorcluster, "resp"=w2109:string, "Device out"=w2112:refnum<class "Channel.lvclass">)  [unwired: 7 in]
          n773 = Fract/Exp String To Number(string=w2109) -> (number=w2107:dbl)  [unwired: 3 in, 1 out]
          n774 = Unbundle By Name(w2112) -> ("Interface.lvclass"=w2111:refnum<class "Interface.lvclass">)
          n775 = call "Read Camera Setup.vi"("Interface in"=w2111) -> ("Camera Setup"=w2110:T4)  [unwired: 8 in, 2 out]
          n776 = Unbundle By Name(w2110) -> ("SHUTTER_TTL"=w2106:u8)
          n777 = Equal?(x=w2106, y=w2107) -> (x = y?=w2108:bool)
          n778 = case shown="True" w2108 {
            tunnel: [w2118 w2119] -> w2115
            tunnel: w2113 -> [w2118 w2120]
            frame False {
            }
            frame True {
              n779 = Increment(x=w2120) -> (x+1=w2119:i32)
            }
          }
        }
        frame 248 {
          n780 = Unbundle By Name(w2129) -> ("Interface.lvclass"=w2128:refnum<class "Interface.lvclass">)
          n781 = call "Read Camera Setup.vi"("Interface in"=w2128) -> ("Camera Setup"=w2122:T4)  [unwired: 8 in, 2 out]
          n782 = Unbundle By Name(w2122) -> ("SHUTTER_OPENNING_TIME"=w2121:u16)
          n783 = Number To Fractional String(number=w2121) -> (F-format string=w2123:string)  [unwired: 3 in]
          n784 = Concatenate Strings("SET SHUTTER_OPENNING_TIME " ("cmd"), w2123) -> (w2127:string)
          n785 = call-dynamic "Write cmd.vi"("error in (no error)"=w2131, "cmd"=w2127, "Device in"=w2129) -> ("error out"=w2130:errorcluster, "Device out"=w2132:refnum<class "Channel.lvclass">)  [unwired: 7 in]
          n786 = Increment(x=w2125) -> (x+1=w2126:i32)
        }
        frame 249 {
          n787 = call-dynamic "Read resp.vi"("error in (no error)"=w2140, "Device in"=w2141) -> ("error out"=w2134:errorcluster, "resp"=w2139:string, "Device out"=w2135:refnum<class "Channel.lvclass">)  [unwired: 7 in]
          n788 = Equal?(x=w2139, y="DONE") -> (x = y?=w2137:bool)
          n789 = case shown="True" w2137 {
            tunnel: [w2142 w2143] -> w2136
            tunnel: w2133 -> [w2142 w2144]
            frame False {
            }
            frame True {
              n790 = Increment(x=w2144) -> (x+1=w2143:i32)
            }
          }
        }
        frame 250 {
          n791 = call-dynamic "Write cmd.vi"("error in (no error)"=w2150, "cmd"="GET SHUTTER_OPENNING_TIME", "Device in"=w2148) -> ("error out"=w2149:errorcluster, "Device out"=w2151:refnum<class "Channel.lvclass">)  [unwired: 7 in]
          n792 = Increment(x=w2146) -> (x+1=w2147:i32)
        }
        frame 251 {
          n793 = call-dynamic "Read resp.vi"("error in (no error)"=w2162, "Device in"=w2163) -> ("error out"=w2160:errorcluster, "resp"=w2155:string, "Device out"=w2158:refnum<class "Channel.lvclass">)  [unwired: 7 in]
          n794 = Fract/Exp String To Number(string=w2155) -> (number=w2153:dbl)  [unwired: 3 in, 1 out]
          n795 = Unbundle By Name(w2158) -> ("Interface.lvclass"=w2157:refnum<class "Interface.lvclass">)
          n796 = call "Read Camera Setup.vi"("Interface in"=w2157) -> ("Camera Setup"=w2156:T4)  [unwired: 8 in, 2 out]
          n797 = Unbundle By Name(w2156) -> ("SHUTTER_OPENNING_TIME"=w2152:u16)
          n798 = Equal?(x=w2152, y=w2153) -> (x = y?=w2154:bool)
          n799 = case shown="True" w2154 {
            tunnel: [w2164 w2165] -> w2161
            tunnel: w2159 -> [w2164 w2166]
            frame False {
            }
            frame True {
              n800 = Increment(x=w2166) -> (x+1=w2165:i32)
            }
          }
        }
        frame 252 {
          n801 = Unbundle By Name(w2175) -> ("Interface.lvclass"=w2174:refnum<class "Interface.lvclass">)
          n802 = call "Read Camera Setup.vi"("Interface in"=w2174) -> ("Camera Setup"=w2168:T4)  [unwired: 8 in, 2 out]
          n803 = Unbundle By Name(w2168) -> ("SHUTTER_CLOSING_TIME"=w2167:u16)
          n804 = Number To Fractional String(number=w2167) -> (F-format string=w2169:string)  [unwired: 3 in]
          n805 = Concatenate Strings("SET SHUTTER_CLOSING_TIME " ("cmd"), w2169) -> (w2173:string)
          n806 = call-dynamic "Write cmd.vi"("error in (no error)"=w2177, "cmd"=w2173, "Device in"=w2175) -> ("error out"=w2176:errorcluster, "Device out"=w2178:refnum<class "Channel.lvclass">)  [unwired: 7 in]
          n807 = Increment(x=w2171) -> (x+1=w2172:i32)
        }
        frame 253 {
          n808 = call-dynamic "Read resp.vi"("error in (no error)"=w2186, "Device in"=w2187) -> ("error out"=w2180:errorcluster, "resp"=w2185:string, "Device out"=w2181:refnum<class "Channel.lvclass">)  [unwired: 7 in]
          n809 = Equal?(x=w2185, y="DONE") -> (x = y?=w2183:bool)
          n810 = case shown="True" w2183 {
            tunnel: [w2188 w2189] -> w2182
            tunnel: w2179 -> [w2188 w2190]
            frame False {
            }
            frame True {
              n811 = Increment(x=w2190) -> (x+1=w2189:i32)
            }
          }
        }
        frame 254 {
          n812 = call-dynamic "Write cmd.vi"("error in (no error)"=w2196, "cmd"="GET SHUTTER_CLOSING_TIME", "Device in"=w2194) -> ("error out"=w2195:errorcluster, "Device out"=w2197:refnum<class "Channel.lvclass">)  [unwired: 7 in]
          n813 = Increment(x=w2192) -> (x+1=w2193:i32)
        }
        frame 255 {
          n814 = call-dynamic "Read resp.vi"("error in (no error)"=w2208, "Device in"=w2209) -> ("error out"=w2206:errorcluster, "resp"=w2201:string, "Device out"=w2204:refnum<class "Channel.lvclass">)  [unwired: 7 in]
          n815 = Fract/Exp String To Number(string=w2201) -> (number=w2199:dbl)  [unwired: 3 in, 1 out]
          n816 = Unbundle By Name(w2204) -> ("Interface.lvclass"=w2203:refnum<class "Interface.lvclass">)
          n817 = call "Read Camera Setup.vi"("Interface in"=w2203) -> ("Camera Setup"=w2202:T4)  [unwired: 8 in, 2 out]
          n818 = Unbundle By Name(w2202) -> ("SHUTTER_CLOSING_TIME"=w2198:u16)
          n819 = Equal?(x=w2198, y=w2199) -> (x = y?=w2200:bool)
          n820 = case shown="True" w2200 {
            tunnel: [w2210 w2211] -> w2207
            tunnel: w2205 -> [w2210 w2212]
            frame False {
            }
            frame True {
              n821 = Increment(x=w2212) -> (x+1=w2211:i32)
            }
          }
        }
        frame 256 {
          n822 = Unbundle By Name(w2221) -> ("Interface.lvclass"=w2220:refnum<class "Interface.lvclass">)
          n823 = call "Read Camera Setup.vi"("Interface in"=w2220) -> ("Camera Setup"=w2214:T4)  [unwired: 8 in, 2 out]
          n824 = Unbundle By Name(w2214) -> ("HBIN"=w2213:u16)
          n825 = Number To Fractional String(number=w2213) -> (F-format string=w2215:string)  [unwired: 3 in]
          n826 = Concatenate Strings("SET HBIN " ("cmd"), w2215) -> (w2219:string)
          n827 = call-dynamic "Write cmd.vi"("error in (no error)"=w2223, "cmd"=w2219, "Device in"=w2221) -> ("error out"=w2222:errorcluster, "Device out"=w2224:refnum<class "Channel.lvclass">)  [unwired: 7 in]
          n828 = Increment(x=w2217) -> (x+1=w2218:i32)
        }
        frame 257 {
          n829 = call-dynamic "Read resp.vi"("error in (no error)"=w2232, "Device in"=w2233) -> ("error out"=w2226:errorcluster, "resp"=w2231:string, "Device out"=w2227:refnum<class "Channel.lvclass">)  [unwired: 7 in]
          n830 = Equal?(x=w2231, y="DONE") -> (x = y?=w2229:bool)
          n831 = case shown="True" w2229 {
            tunnel: [w2234 w2235] -> w2228
            tunnel: w2225 -> [w2234 w2236]
            frame False {
            }
            frame True {
              n832 = Increment(x=w2236) -> (x+1=w2235:i32)
            }
          }
        }
        frame 258 {
          n833 = call-dynamic "Write cmd.vi"("error in (no error)"=w2242, "cmd"="GET HBIN", "Device in"=w2240) -> ("error out"=w2241:errorcluster, "Device out"=w2243:refnum<class "Channel.lvclass">)  [unwired: 7 in]
          n834 = Increment(x=w2238) -> (x+1=w2239:i32)
        }
        frame 259 {
          n835 = call-dynamic "Read resp.vi"("error in (no error)"=w2254, "Device in"=w2255) -> ("error out"=w2252:errorcluster, "resp"=w2247:string, "Device out"=w2250:refnum<class "Channel.lvclass">)  [unwired: 7 in]
          n836 = Fract/Exp String To Number(string=w2247) -> (number=w2245:dbl)  [unwired: 3 in, 1 out]
          n837 = Unbundle By Name(w2250) -> ("Interface.lvclass"=w2249:refnum<class "Interface.lvclass">)
          n838 = call "Read Camera Setup.vi"("Interface in"=w2249) -> ("Camera Setup"=w2248:T4)  [unwired: 8 in, 2 out]
          n839 = Unbundle By Name(w2248) -> ("HBIN"=w2244:u16)
          n840 = Equal?(x=w2244, y=w2245) -> (x = y?=w2246:bool)
          n841 = case shown="True" w2246 {
            tunnel: [w2256 w2257] -> w2253
            tunnel: w2251 -> [w2256 w2258]
            frame False {
            }
            frame True {
              n842 = Increment(x=w2258) -> (x+1=w2257:i32)
            }
          }
        }
        frame 260 {
          n843 = Unbundle By Name(w2267) -> ("Interface.lvclass"=w2266:refnum<class "Interface.lvclass">)
          n844 = call "Read Camera Setup.vi"("Interface in"=w2266) -> ("Camera Setup"=w2260:T4)  [unwired: 8 in, 2 out]
          n845 = Unbundle By Name(w2260) -> ("VBIN"=w2259:u16)
          n846 = Number To Fractional String(number=w2259) -> (F-format string=w2261:string)  [unwired: 3 in]
          n847 = Concatenate Strings("SET VBIN " ("cmd"), w2261) -> (w2265:string)
          n848 = call-dynamic "Write cmd.vi"("error in (no error)"=w2269, "cmd"=w2265, "Device in"=w2267) -> ("error out"=w2268:errorcluster, "Device out"=w2270:refnum<class "Channel.lvclass">)  [unwired: 7 in]
          n849 = Increment(x=w2263) -> (x+1=w2264:i32)
        }
        frame 261 {
          n850 = call-dynamic "Read resp.vi"("error in (no error)"=w2278, "Device in"=w2279) -> ("error out"=w2272:errorcluster, "resp"=w2277:string, "Device out"=w2273:refnum<class "Channel.lvclass">)  [unwired: 7 in]
          n851 = Equal?(x=w2277, y="DONE") -> (x = y?=w2275:bool)
          n852 = case shown="True" w2275 {
            tunnel: [w2280 w2281] -> w2274
            tunnel: w2271 -> [w2280 w2282]
            frame False {
            }
            frame True {
              n853 = Increment(x=w2282) -> (x+1=w2281:i32)
            }
          }
        }
        frame 262 {
          n854 = call-dynamic "Write cmd.vi"("error in (no error)"=w2288, "cmd"="GET VBIN", "Device in"=w2286) -> ("error out"=w2287:errorcluster, "Device out"=w2289:refnum<class "Channel.lvclass">)  [unwired: 7 in]
          n855 = Increment(x=w2284) -> (x+1=w2285:i32)
        }
        frame 263 {
          n856 = call-dynamic "Read resp.vi"("error in (no error)"=w2300, "Device in"=w2301) -> ("error out"=w2298:errorcluster, "resp"=w2293:string, "Device out"=w2296:refnum<class "Channel.lvclass">)  [unwired: 7 in]
          n857 = Fract/Exp String To Number(string=w2293) -> (number=w2291:dbl)  [unwired: 3 in, 1 out]
          n858 = Unbundle By Name(w2296) -> ("Interface.lvclass"=w2295:refnum<class "Interface.lvclass">)
          n859 = call "Read Camera Setup.vi"("Interface in"=w2295) -> ("Camera Setup"=w2294:T4)  [unwired: 8 in, 2 out]
          n860 = Unbundle By Name(w2294) -> ("VBIN"=w2290:u16)
          n861 = Equal?(x=w2290, y=w2291) -> (x = y?=w2292:bool)
          n862 = case shown="True" w2292 {
            tunnel: [w2302 w2303] -> w2299
            tunnel: w2297 -> [w2302 w2304]
            frame False {
            }
            frame True {
              n863 = Increment(x=w2304) -> (x+1=w2303:i32)
            }
          }
        }
        frame 264 {
          n864 = Unbundle By Name(w2313) -> ("Interface.lvclass"=w2312:refnum<class "Interface.lvclass">)
          n865 = call "Read Camera Setup.vi"("Interface in"=w2312) -> ("Camera Setup"=w2306:T4)  [unwired: 8 in, 2 out]
          n866 = Unbundle By Name(w2306) -> ("INITIAL_LINE"=w2305:u16)
          n867 = Number To Fractional String(number=w2305) -> (F-format string=w2307:string)  [unwired: 3 in]
          n868 = Concatenate Strings("SET INITIAL_LINE " ("cmd"), w2307) -> (w2311:string)
          n869 = call-dynamic "Write cmd.vi"("error in (no error)"=w2315, "cmd"=w2311, "Device in"=w2313) -> ("error out"=w2314:errorcluster, "Device out"=w2316:refnum<class "Channel.lvclass">)  [unwired: 7 in]
          n870 = Increment(x=w2309) -> (x+1=w2310:i32)
        }
        frame 265 {
          n871 = call-dynamic "Read resp.vi"("error in (no error)"=w2324, "Device in"=w2325) -> ("error out"=w2318:errorcluster, "resp"=w2323:string, "Device out"=w2319:refnum<class "Channel.lvclass">)  [unwired: 7 in]
          n872 = Equal?(x=w2323, y="DONE") -> (x = y?=w2321:bool)
          n873 = case shown="True" w2321 {
            tunnel: [w2326 w2327] -> w2320
            tunnel: w2317 -> [w2326 w2328]
            frame False {
            }
            frame True {
              n874 = Increment(x=w2328) -> (x+1=w2327:i32)
            }
          }
        }
        frame 266 {
          n875 = call-dynamic "Write cmd.vi"("error in (no error)"=w2334, "cmd"="GET INITIAL_LINE", "Device in"=w2332) -> ("error out"=w2333:errorcluster, "Device out"=w2335:refnum<class "Channel.lvclass">)  [unwired: 7 in]
          n876 = Increment(x=w2330) -> (x+1=w2331:i32)
        }
        frame 267 {
          n877 = call-dynamic "Read resp.vi"("error in (no error)"=w2346, "Device in"=w2347) -> ("error out"=w2344:errorcluster, "resp"=w2339:string, "Device out"=w2342:refnum<class "Channel.lvclass">)  [unwired: 7 in]
          n878 = Fract/Exp String To Number(string=w2339) -> (number=w2337:dbl)  [unwired: 3 in, 1 out]
          n879 = Unbundle By Name(w2342) -> ("Interface.lvclass"=w2341:refnum<class "Interface.lvclass">)
          n880 = call "Read Camera Setup.vi"("Interface in"=w2341) -> ("Camera Setup"=w2340:T4)  [unwired: 8 in, 2 out]
          n881 = Unbundle By Name(w2340) -> ("INITIAL_LINE"=w2336:u16)
          n882 = Equal?(x=w2336, y=w2337) -> (x = y?=w2338:bool)
          n883 = case shown="True" w2338 {
            tunnel: [w2348 w2349] -> w2345
            tunnel: w2343 -> [w2348 w2350]
            frame False {
            }
            frame True {
              n884 = Increment(x=w2350) -> (x+1=w2349:i32)
            }
          }
        }
        frame 268 {
          n885 = Unbundle By Name(w2359) -> ("Interface.lvclass"=w2358:refnum<class "Interface.lvclass">)
          n886 = call "Read Camera Setup.vi"("Interface in"=w2358) -> ("Camera Setup"=w2352:T4)  [unwired: 8 in, 2 out]
          n887 = Unbundle By Name(w2352) -> ("INITIAL_COLUMN"=w2351:u16)
          n888 = Number To Fractional String(number=w2351) -> (F-format string=w2353:string)  [unwired: 3 in]
          n889 = Concatenate Strings("SET INITIAL_COLUMN " ("cmd"), w2353) -> (w2357:string)
          n890 = call-dynamic "Write cmd.vi"("error in (no error)"=w2361, "cmd"=w2357, "Device in"=w2359) -> ("error out"=w2360:errorcluster, "Device out"=w2362:refnum<class "Channel.lvclass">)  [unwired: 7 in]
          n891 = Increment(x=w2355) -> (x+1=w2356:i32)
        }
        frame 269 {
          n892 = call-dynamic "Read resp.vi"("error in (no error)"=w2370, "Device in"=w2371) -> ("error out"=w2364:errorcluster, "resp"=w2369:string, "Device out"=w2365:refnum<class "Channel.lvclass">)  [unwired: 7 in]
          n893 = Equal?(x=w2369, y="DONE") -> (x = y?=w2367:bool)
          n894 = case shown="True" w2367 {
            tunnel: [w2372 w2373] -> w2366
            tunnel: w2363 -> [w2372 w2374]
            frame False {
            }
            frame True {
              n895 = Increment(x=w2374) -> (x+1=w2373:i32)
            }
          }
        }
        frame 270 {
          n896 = call-dynamic "Write cmd.vi"("error in (no error)"=w2380, "cmd"="GET INITIAL_COLUMN", "Device in"=w2378) -> ("error out"=w2379:errorcluster, "Device out"=w2381:refnum<class "Channel.lvclass">)  [unwired: 7 in]
          n897 = Increment(x=w2376) -> (x+1=w2377:i32)
        }
        frame 271 {
          n898 = call-dynamic "Read resp.vi"("error in (no error)"=w2392, "Device in"=w2393) -> ("error out"=w2390:errorcluster, "resp"=w2385:string, "Device out"=w2388:refnum<class "Channel.lvclass">)  [unwired: 7 in]
          n899 = Fract/Exp String To Number(string=w2385) -> (number=w2383:dbl)  [unwired: 3 in, 1 out]
          n900 = Unbundle By Name(w2388) -> ("Interface.lvclass"=w2387:refnum<class "Interface.lvclass">)
          n901 = call "Read Camera Setup.vi"("Interface in"=w2387) -> ("Camera Setup"=w2386:T4)  [unwired: 8 in, 2 out]
          n902 = Unbundle By Name(w2386) -> ("INITIAL_COLUMN"=w2382:u16)
          n903 = Equal?(x=w2382, y=w2383) -> (x = y?=w2384:bool)
          n904 = case shown="True" w2384 {
            tunnel: [w2394 w2395] -> w2391
            tunnel: w2389 -> [w2394 w2396]
            frame False {
            }
            frame True {
              n905 = Increment(x=w2396) -> (x+1=w2395:i32)
            }
          }
        }
        frame 272 {
          n906 = Unbundle By Name(w2405) -> ("Interface.lvclass"=w2404:refnum<class "Interface.lvclass">)
          n907 = call "Read Camera Setup.vi"("Interface in"=w2404) -> ("Camera Setup"=w2398:T4)  [unwired: 8 in, 2 out]
          n908 = Unbundle By Name(w2398) -> ("FINAL_LINE"=w2397:u16)
          n909 = Number To Fractional String(number=w2397) -> (F-format string=w2399:string)  [unwired: 3 in]
          n910 = Concatenate Strings("SET FINAL_LINE " ("cmd"), w2399) -> (w2403:string)
          n911 = call-dynamic "Write cmd.vi"("error in (no error)"=w2407, "cmd"=w2403, "Device in"=w2405) -> ("error out"=w2406:errorcluster, "Device out"=w2408:refnum<class "Channel.lvclass">)  [unwired: 7 in]
          n912 = Increment(x=w2401) -> (x+1=w2402:i32)
        }
        frame 273 {
          n913 = call-dynamic "Read resp.vi"("error in (no error)"=w2416, "Device in"=w2417) -> ("error out"=w2410:errorcluster, "resp"=w2415:string, "Device out"=w2411:refnum<class "Channel.lvclass">)  [unwired: 7 in]
          n914 = Equal?(x=w2415, y="DONE") -> (x = y?=w2413:bool)
          n915 = case shown="True" w2413 {
            tunnel: [w2418 w2419] -> w2412
            tunnel: w2409 -> [w2418 w2420]
            frame False {
            }
            frame True {
              n916 = Increment(x=w2420) -> (x+1=w2419:i32)
            }
          }
        }
        frame 274 {
          n917 = call-dynamic "Write cmd.vi"("error in (no error)"=w2426, "cmd"="GET FINAL_LINE", "Device in"=w2424) -> ("error out"=w2425:errorcluster, "Device out"=w2427:refnum<class "Channel.lvclass">)  [unwired: 7 in]
          n918 = Increment(x=w2422) -> (x+1=w2423:i32)
        }
        frame 275 {
          n919 = call-dynamic "Read resp.vi"("error in (no error)"=w2438, "Device in"=w2439) -> ("error out"=w2436:errorcluster, "resp"=w2431:string, "Device out"=w2434:refnum<class "Channel.lvclass">)  [unwired: 7 in]
          n920 = Fract/Exp String To Number(string=w2431) -> (number=w2429:dbl)  [unwired: 3 in, 1 out]
          n921 = Unbundle By Name(w2434) -> ("Interface.lvclass"=w2433:refnum<class "Interface.lvclass">)
          n922 = call "Read Camera Setup.vi"("Interface in"=w2433) -> ("Camera Setup"=w2432:T4)  [unwired: 8 in, 2 out]
          n923 = Unbundle By Name(w2432) -> ("FINAL_LINE"=w2428:u16)
          n924 = Equal?(x=w2428, y=w2429) -> (x = y?=w2430:bool)
          n925 = case shown="True" w2430 {
            tunnel: [w2440 w2441] -> w2437
            tunnel: w2435 -> [w2440 w2442]
            frame False {
            }
            frame True {
              n926 = Increment(x=w2442) -> (x+1=w2441:i32)
            }
          }
        }
        frame 276 {
          n927 = Unbundle By Name(w2451) -> ("Interface.lvclass"=w2450:refnum<class "Interface.lvclass">)
          n928 = call "Read Camera Setup.vi"("Interface in"=w2450) -> ("Camera Setup"=w2444:T4)  [unwired: 8 in, 2 out]
          n929 = Unbundle By Name(w2444) -> ("FINAL_COLUMN"=w2443:u16)
          n930 = Number To Fractional String(number=w2443) -> (F-format string=w2445:string)  [unwired: 3 in]
          n931 = Concatenate Strings("SET FINAL_COLUMN " ("cmd"), w2445) -> (w2449:string)
          n932 = call-dynamic "Write cmd.vi"("error in (no error)"=w2453, "cmd"=w2449, "Device in"=w2451) -> ("error out"=w2452:errorcluster, "Device out"=w2454:refnum<class "Channel.lvclass">)  [unwired: 7 in]
          n933 = Increment(x=w2447) -> (x+1=w2448:i32)
        }
        frame 277 {
          n934 = call-dynamic "Read resp.vi"("error in (no error)"=w2462, "Device in"=w2463) -> ("error out"=w2456:errorcluster, "resp"=w2461:string, "Device out"=w2457:refnum<class "Channel.lvclass">)  [unwired: 7 in]
          n935 = Equal?(x=w2461, y="DONE") -> (x = y?=w2459:bool)
          n936 = case shown="True" w2459 {
            tunnel: [w2464 w2465] -> w2458
            tunnel: w2455 -> [w2464 w2466]
            frame False {
            }
            frame True {
              n937 = Increment(x=w2466) -> (x+1=w2465:i32)
            }
          }
        }
        frame 278 {
          n938 = call-dynamic "Write cmd.vi"("error in (no error)"=w2472, "cmd"="GET FINAL_COLUMN", "Device in"=w2470) -> ("error out"=w2471:errorcluster, "Device out"=w2473:refnum<class "Channel.lvclass">)  [unwired: 7 in]
          n939 = Increment(x=w2468) -> (x+1=w2469:i32)
        }
        frame 279 {
          n940 = call-dynamic "Read resp.vi"("error in (no error)"=w2484, "Device in"=w2485) -> ("error out"=w2482:errorcluster, "resp"=w2477:string, "Device out"=w2480:refnum<class "Channel.lvclass">)  [unwired: 7 in]
          n941 = Fract/Exp String To Number(string=w2477) -> (number=w2475:dbl)  [unwired: 3 in, 1 out]
          n942 = Unbundle By Name(w2480) -> ("Interface.lvclass"=w2479:refnum<class "Interface.lvclass">)
          n943 = call "Read Camera Setup.vi"("Interface in"=w2479) -> ("Camera Setup"=w2478:T4)  [unwired: 8 in, 2 out]
          n944 = Unbundle By Name(w2478) -> ("FINAL_COLUMN"=w2474:u16)
          n945 = Equal?(x=w2474, y=w2475) -> (x = y?=w2476:bool)
          n946 = disable-structure shown="Enabled" {
            disable-tunnel: [w2488 0 ("State")] -> w2483
            disable-tunnel: w2481 -> [w2487 _]
            disable-tunnel: w2476 -> [w2486 _]
            frame Disabled {
              n947 = case shown="True" w2486 {
                tunnel: [w2489 w2490] -> w2488
                tunnel: w2487 -> [w2489 w2491]
                frame False {
                }
                frame True {
                  n948 = Increment(x=w2491) -> (x+1=w2490:i32)
                }
              }
            }
            frame Enabled {
            }
          }
        }
        frame 280 {
          n949 = Unbundle By Name(w2501) -> ("Interface.lvclass"=w2500:refnum<class "Interface.lvclass">)
          n950 = call "Read Camera Setup.vi"("Interface in"=w2500) -> ("Camera Setup"=w2494:T4)  [unwired: 8 in, 2 out]
          n951 = Unbundle By Name(w2494) -> ("VERTICAL_CLOCK_VOLTAGE"=w2493:u8)
          n952 = Number To Fractional String(number=w2493) -> (F-format string=w2495:string)  [unwired: 3 in]
          n953 = Concatenate Strings("SET VERTICAL_CLOCK_VOLTAGE " ("cmd"), w2495) -> (w2499:string)
          n954 = call-dynamic "Write cmd.vi"("error in (no error)"=w2503, "cmd"=w2499, "Device in"=w2501) -> ("error out"=w2502:errorcluster, "Device out"=w2504:refnum<class "Channel.lvclass">)  [unwired: 7 in]
          n955 = Increment(x=w2497) -> (x+1=w2498:i32)
        }
        frame 281 {
          n956 = call-dynamic "Read resp.vi"("error in (no error)"=w2512, "Device in"=w2513) -> ("error out"=w2506:errorcluster, "resp"=w2511:string, "Device out"=w2507:refnum<class "Channel.lvclass">)  [unwired: 7 in]
          n957 = Equal?(x=w2511, y="DONE") -> (x = y?=w2509:bool)
          n958 = case shown="True" w2509 {
            tunnel: [w2514 w2515] -> w2508
            tunnel: w2505 -> [w2514 w2516]
            frame False {
            }
            frame True {
              n959 = Increment(x=w2516) -> (x+1=w2515:i32)
            }
          }
        }
        frame 282 {
          n960 = call-dynamic "Write cmd.vi"("error in (no error)"=w2522, "cmd"="GET VERTICAL_CLOCK_VOLTAGE", "Device in"=w2520) -> ("error out"=w2521:errorcluster, "Device out"=w2523:refnum<class "Channel.lvclass">)  [unwired: 7 in]
          n961 = Increment(x=w2518) -> (x+1=w2519:i32)
        }
        frame 283 {
          n962 = call-dynamic "Read resp.vi"("error in (no error)"=w2534, "Device in"=w2535) -> ("error out"=w2532:errorcluster, "resp"=w2527:string, "Device out"=w2530:refnum<class "Channel.lvclass">)  [unwired: 7 in]
          n963 = Fract/Exp String To Number(string=w2527) -> (number=w2525:dbl)  [unwired: 3 in, 1 out]
          n964 = Unbundle By Name(w2530) -> ("Interface.lvclass"=w2529:refnum<class "Interface.lvclass">)
          n965 = call "Read Camera Setup.vi"("Interface in"=w2529) -> ("Camera Setup"=w2528:T4)  [unwired: 8 in, 2 out]
          n966 = Unbundle By Name(w2528) -> ("VERTICAL_CLOCK_VOLTAGE"=w2524:u8)
          n967 = Equal?(x=w2524, y=w2525) -> (x = y?=w2526:bool)
          n968 = case shown="True" w2526 {
            tunnel: [w2536 w2537] -> w2533
            tunnel: w2531 -> [w2536 w2538]
            frame False {
            }
            frame True {
              n969 = Increment(x=w2538) -> (x+1=w2537:i32)
            }
          }
        }
        frame 284 {
          n970 = Unbundle By Name(w2547) -> ("Interface.lvclass"=w2546:refnum<class "Interface.lvclass">)
          n971 = call "Read Camera Setup.vi"("Interface in"=w2546) -> ("Camera Setup"=w2541:T4)  [unwired: 8 in, 2 out]
          n972 = Unbundle By Name(w2541) -> ("FRAME_TRANSFER"=w2540:bool)
          n973 = case shown="True" w2540 {
            tunnel: ["T" ("cmd") "F" ("cmd")] -> w2539
            frame True {
            }
            frame False {
            }
          }
          n974 = Concatenate Strings("SET FRAME_TRANSFER " ("cmd"), w2539) -> (w2545:string)
          n975 = call-dynamic "Write cmd.vi"("error in (no error)"=w2549, "cmd"=w2545, "Device in"=w2547) -> ("error out"=w2548:errorcluster, "Device out"=w2550:refnum<class "Channel.lvclass">)  [unwired: 7 in]
          n976 = Increment(x=w2543) -> (x+1=w2544:i32)
        }
        frame 285 {
          n977 = call-dynamic "Read resp.vi"("error in (no error)"=w2560, "Device in"=w2561) -> ("error out"=w2554:errorcluster, "resp"=w2559:string, "Device out"=w2555:refnum<class "Channel.lvclass">)  [unwired: 7 in]
          n978 = Equal?(x=w2559, y="DONE") -> (x = y?=w2557:bool)
          n979 = case shown="True" w2557 {
            tunnel: [w2562 w2563] -> w2556
            tunnel: w2553 -> [w2562 w2564]
            frame False {
            }
            frame True {
              n980 = Increment(x=w2564) -> (x+1=w2563:i32)
            }
          }
        }
        frame 286 {
          n981 = call-dynamic "Write cmd.vi"("error in (no error)"=w2570, "cmd"="GET FRAME_TRANSFER", "Device in"=w2568) -> ("error out"=w2569:errorcluster, "Device out"=w2571:refnum<class "Channel.lvclass">)  [unwired: 7 in]
          n982 = Increment(x=w2566) -> (x+1=w2567:i32)
        }
        frame 287 {
          n983 = call-dynamic "Read resp.vi"("error in (no error)"=w2582, "Device in"=w2583) -> ("error out"=w2580:errorcluster, "resp"=w2574:string, "Device out"=w2578:refnum<class "Channel.lvclass">)  [unwired: 7 in]
          n984 = Unbundle By Name(w2578) -> ("Interface.lvclass"=w2577:refnum<class "Interface.lvclass">)
          n985 = call "Read Camera Setup.vi"("Interface in"=w2577) -> ("Camera Setup"=w2576:T4)  [unwired: 8 in, 2 out]
          n986 = Unbundle By Name(w2576) -> ("FRAME_TRANSFER"=w2573:bool)
          n987 = case shown="True" w2573 {
            tunnel: ["T" "F"] -> w2572
            frame True {
            }
            frame False {
            }
          }
          n988 = Equal?(x=w2572, y=w2574) -> (x = y?=w2575:bool)
          n989 = case shown="True" w2575 {
            tunnel: [w2586 w2587] -> w2581
            tunnel: w2579 -> [w2586 w2588]
            frame False {
            }
            frame True {
              n990 = Increment(x=w2588) -> (x+1=w2587:i32)
            }
          }
        }
        frame 288 {
          n991 = Unbundle By Name(w2597) -> ("Interface.lvclass"=w2596:refnum<class "Interface.lvclass">)
          n992 = call "Read Camera Setup.vi"("Interface in"=w2596) -> ("Camera Setup"=w2590:T4)  [unwired: 8 in, 2 out]
          n993 = Unbundle By Name(w2590) -> ("AD_CHANNEL"=w2589:u32)
          n994 = Number To Fractional String(number=w2589) -> (F-format string=w2591:string)  [unwired: 3 in]
          n995 = Concatenate Strings("SET AD_CHANNEL " ("cmd"), w2591) -> (w2595:string)
          n996 = call-dynamic "Write cmd.vi"("error in (no error)"=w2599, "cmd"=w2595, "Device in"=w2597) -> ("error out"=w2598:errorcluster, "Device out"=w2600:refnum<class "Channel.lvclass">)  [unwired: 7 in]
          n997 = Increment(x=w2593) -> (x+1=w2594:i32)
        }
        frame 289 {
          n998 = call-dynamic "Read resp.vi"("error in (no error)"=w2608, "Device in"=w2609) -> ("error out"=w2602:errorcluster, "resp"=w2607:string, "Device out"=w2603:refnum<class "Channel.lvclass">)  [unwired: 7 in]
          n999 = Equal?(x=w2607, y="DONE") -> (x = y?=w2605:bool)
          n1000 = case shown="True" w2605 {
            tunnel: [w2610 w2611] -> w2604
            tunnel: w2601 -> [w2610 w2612]
            frame False {
            }
            frame True {
              n1001 = Increment(x=w2612) -> (x+1=w2611:i32)
            }
          }
        }
        frame 290 {
          n1002 = call-dynamic "Write cmd.vi"("error in (no error)"=w2618, "cmd"="GET AD_CHANNEL", "Device in"=w2616) -> ("error out"=w2617:errorcluster, "Device out"=w2619:refnum<class "Channel.lvclass">)  [unwired: 7 in]
          n1003 = Increment(x=w2614) -> (x+1=w2615:i32)
        }
        frame 291 {
          n1004 = call-dynamic "Read resp.vi"("error in (no error)"=w2630, "Device in"=w2631) -> ("error out"=w2628:errorcluster, "resp"=w2623:string, "Device out"=w2626:refnum<class "Channel.lvclass">)  [unwired: 7 in]
          n1005 = Fract/Exp String To Number(string=w2623) -> (number=w2621:dbl)  [unwired: 3 in, 1 out]
          n1006 = Unbundle By Name(w2626) -> ("Interface.lvclass"=w2625:refnum<class "Interface.lvclass">)
          n1007 = call "Read Camera Setup.vi"("Interface in"=w2625) -> ("Camera Setup"=w2624:T4)  [unwired: 8 in, 2 out]
          n1008 = Unbundle By Name(w2624) -> ("AD_CHANNEL"=w2620:u32)
          n1009 = Equal?(x=w2620, y=w2621) -> (x = y?=w2622:bool)
          n1010 = case shown="True" w2622 {
            tunnel: [w2632 w2633] -> w2629
            tunnel: w2627 -> [w2632 w2634]
            frame False {
            }
            frame True {
              n1011 = Increment(x=w2634) -> (x+1=w2633:i32)
            }
          }
        }
        frame 300 {
          # "suffix"
          n1012 = call-dynamic "Write Timer.vi"("error in (no error)"=w2637, "Timer"=u32 200, "State Machine in"=w2641) -> ("error out"=w2642:errorcluster, "State Machine out"=w2635:refnum<class "State Machine.lvclass">)  [unwired: 7 in]
          n1013 = call-dynamic "Write State Machine.vi"("error in (no error)"=w2642, "State Machine.lvclass"=w2635, "Device in"=w2639) -> ("error out"=w2636:errorcluster, "Device out"=w2638:refnum<class "Channel.lvclass">)  [unwired: 7 in]
          n1014 = Unbundle By Name(w2638) -> ("Interface.lvclass"=w2648:refnum<class "Interface.lvclass">)
          n1015 = call-dynamic "Read Suffix.vi"("Interface in"=w2648) -> ("Suffix"=w2643:string)  [unwired: 8 in, 2 out]
          n1016 = Concatenate Strings("SET SUFFIX " ("cmd"), w2643) -> (w2647:string)
          n1017 = call-dynamic "Write cmd.vi"("error in (no error)"=w2636, "cmd"=w2647, "Device in"=w2638) -> ("error out"=w2649:errorcluster, "Device out"=w2650:refnum<class "Channel.lvclass">)  [unwired: 7 in]
          n1018 = Increment(x=w2645) -> (x+1=w2646:i32)
        }
        frame 301 {
          # "Compara o parametro enviado com\no parametro no Acquisition Configuration\nda msg de STATUS do ACS."
          # "Verifica timeout para ACS responder.\nSe estourar timeout é porque o ACS não \nrespondeu e este canal volta para o estado 0\npara não \"travar\" os outros canais no \nS4ACS_GUI:HandleObservation.vi."
          n1019 = call "Verify Timer.vi"("error in (no error)"=w2682, "State Machine in"=w2684) -> ("error out"=w2681:errorcluster, "timeout"=w2679:bool, "State Machine out"=w2683:refnum<class "State Machine.lvclass">)  [unwired: 7 in]
          n1020 = call-dynamic "Write State Machine.vi"("error in (no error)"=w2681, "State Machine.lvclass"=w2683, "Device in"=w2685) -> ("error out"=w2680:errorcluster, "Device out"=w2676:refnum<class "Channel.lvclass">)  [unwired: 7 in]
          n1021 = call-dynamic "Read resp.vi"("error in (no error)"=w2680, "Device in"=w2676) -> ("error out"=w2670:errorcluster, "resp"=w2654:string, "Device out"=w2675:refnum<class "Channel.lvclass">)  [unwired: 7 in]
          n1022 = Unbundle By Name(w2675) -> ("Interface.lvclass"=w2674:refnum<class "Interface.lvclass">)
          n1023 = call-dynamic "UpdateACQconf.vi"("error in (no error)"=w2670, "status"=w2654, "Interface in"=w2674) -> ("error out"=w2669:errorcluster, "ACQ conf rx"=w2672:T2, "Interface out"=w2673:refnum<class "Interface.lvclass">)  [unwired: 6 in]
          n1024 = Unbundle By Name(w2672) -> ("suffix"=w2671:string)
          n1025 = call-dynamic "Read Suffix.vi"("error in (no error)"=w2669, "Interface in"=w2673) -> ("error out"=w2653:errorcluster, "Suffix"=w2668:string, "Interface out"=w2656:refnum<class "Interface.lvclass">)  [unwired: 7 in]
          n1026 = Equal?(x=w2668, y=w2671) -> (x = y?=w2667:bool)
          n1027 = call-dynamic "UpdateS4GUI_JSON_string.vi"("error in (no error)"=w2653, "status"=w2654, "Interface in"=w2656) -> ("error out"=w2652:errorcluster, "S4GUI JSON string rx"=w2651:T5, "Interface out"=w2655:refnum<class "Interface.lvclass">)  [unwired: 6 in]
          n1028 = Unbundle By Name(w2651) -> ("OBSTYPE"=w2660:string, "OBJECT"=w2659:string)
          n1029 = call-dynamic "Read ObsType.vi"("error in (no error)"=w2652, "Interface in"=w2655) -> ("error out"=w2665:errorcluster, "ObsType"=w2662:string, "Interface out"=w2663:refnum<class "Interface.lvclass">)  [unwired: 7 in]
          n1030 = call-dynamic "Read Object.vi"("error in (no error)"=w2665, "Interface in"=w2663) -> ("error out"=w2664:errorcluster, "Object"=w2661:string)  [unwired: 7 in, 1 out]
          n1031 = Equal?(x=w2662, y=w2660) -> (x = y?=w2658:bool)
          n1032 = Equal?(x=w2661, y=w2659) -> (x = y?=w2657:bool)
          n1033 = disable-structure shown="Enabled" {
            disable-tunnel: w2667 -> [w2689 w2690]
            disable-tunnel: [w2688 w2690] -> w2666
            disable-tunnel: w2658 -> [w2687 _]
            disable-tunnel: w2657 -> [w2686 _]
            frame Enabled {
              n1034 = Compound Arithmetic op=AND(w2689, w2687, w2686) -> (w2688:bool)
            }
            frame Disabled {
            }
          }
          n1035 = case shown="False" w2679 {
            tunnel: [w2692 27] -> w2677
            tunnel: w2678 -> [w2693 _]
            tunnel: w2666 -> [w2691 _]
            frame False {
              n1036 = case shown="True" w2691 {
                tunnel: [w2694 w2695] -> w2692
                tunnel: w2693 -> [w2694 w2696]
                frame False {
                }
                frame True {
                  n1037 = Increment(x=w2696) -> (x+1=w2695:i32)
                }
              }
            }
            frame True {
              # "ERRO"
            }
          }
        }
        frame 302 {
          # "2024-03-20:\nSó envia o SUFFIX por comando SET.\nO resto dos parametros estão na  \npublicação do STATUS do S4GUI."
          n1038 = call "Verify Timer.vi"("error in (no error)"=w2706, "State Machine in"=w2707) -> ("error out"=w2703:errorcluster, "timeout"=w2698:bool, "State Machine out"=w2704:refnum<class "State Machine.lvclass">)  [unwired: 7 in]
          n1039 = call-dynamic "Write State Machine.vi"("error in (no error)"=w2703, "State Machine.lvclass"=w2704, "Device in"=w2705) -> ("error out"=w2702:errorcluster, "Device out"=w2701:refnum<class "Channel.lvclass">)  [unwired: 7 in]
          n1040 = case shown="True" w2698 {
            tunnel: [w2708 40 ("State")] -> w2700
            tunnel: w2699 -> [w2708 _]
            frame False {
            }
            frame True {
            }
          }
        }
        frame 312 {
          # "filter"
          n1041 = call-dynamic "Write Timer.vi"("error in (no error)"=w2715, "Timer"=u32 50, "State Machine in"=w2713) -> ("error out"=w2720:errorcluster, "State Machine out"=w2718:refnum<class "State Machine.lvclass">)  [unwired: 7 in]
          n1042 = call-dynamic "Write State Machine.vi"("error in (no error)"=w2720, "State Machine.lvclass"=w2718, "Device in"=w2717) -> ("error out"=w2710:errorcluster, "Device out"=w2716:refnum<class "Channel.lvclass">)  [unwired: 7 in]
          n1043 = Unbundle By Name(w2716) -> ("Filter"=w2712:u8)
          n1044 = case shown="0, Default" w2712 {
            tunnel: ["U" ("cmd") "B" ("cmd") "V" ("cmd") "R" ("cmd") "I" ("cmd") "CLEAR" ("cmd")] -> w2711
            frame 1 {
            }
            frame 2 {
            }
            frame 3 {
            }
            frame 4 {
            }
            frame 5 {
            }
            frame 0, Default {
            }
          }
          n1045 = Concatenate Strings("SET FILTER " ("cmd"), w2711) -> (w2723:string)
          n1046 = call-dynamic "Write cmd.vi"("error in (no error)"=w2710, "cmd"=w2723, "Device in"=w2716) -> ("error out"=w2724:errorcluster, "Device out"=w2725:refnum<class "Channel.lvclass">)  [unwired: 7 in]
          n1047 = Increment(x=w2721) -> (x+1=w2722:i32)
        }
        frame 313 {
          n1048 = call "Verify Timer.vi"("error in (no error)"=w2740, "State Machine in"=w2738) -> ("error out"=w2739:errorcluster, "timeout"=w2735:bool, "State Machine out"=w2742:refnum<class "State Machine.lvclass">)  [unwired: 7 in]
          n1049 = call-dynamic "Write State Machine.vi"("error in (no error)"=w2739, "State Machine.lvclass"=w2742, "Device in"=w2741) -> ("error out"=w2736:errorcluster, "Device out"=w2737:refnum<class "Channel.lvclass">)  [unwired: 7 in]
          n1050 = call-dynamic "Read resp.vi"("error in (no error)"=w2736, "Device in"=w2737) -> ("error out"=w2743:errorcluster, "resp"=w2746:string, "Device out"=w2744:refnum<class "Channel.lvclass">)  [unwired: 7 in]
          n1051 = Equal?(x=w2746, y="DONE") -> (x = y?=w2733:bool)
          n1052 = case shown="False" w2735 {
            tunnel: [w2748 0] -> w2732
            tunnel: w2734 -> [w2749 _]
            tunnel: w2733 -> [w2747 _]
            frame False {
              n1053 = case shown="True" w2747 {
                tunnel: w2749 -> [w2750 w2752]
                tunnel: [w2750 w2751] -> w2748
                frame False {
                }
                frame True {
                  n1054 = Increment(x=w2752) -> (x+1=w2751:i32)
                }
              }
            }
            frame True {
            }
          }
        }
        frame 314 {
          n1055 = call-dynamic "Write Timer.vi"("error in (no error)"=w2757, "Timer"=u32 50, "State Machine in"=w2756) -> ("error out"=w2762:errorcluster, "State Machine out"=w2760:refnum<class "State Machine.lvclass">)  [unwired: 7 in]
          n1056 = call-dynamic "Write State Machine.vi"("error in (no error)"=w2762, "State Machine.lvclass"=w2760, "Device in"=w2759) -> ("error out"=w2755:errorcluster, "Device out"=w2758:refnum<class "Channel.lvclass">)  [unwired: 7 in]
          n1057 = call-dynamic "Write cmd.vi"("error in (no error)"=w2755, "cmd"="SET CTRLINTE S4GUI", "Device in"=w2758) -> ("error out"=w2765:errorcluster, "Device out"=w2766:refnum<class "Channel.lvclass">)  [unwired: 7 in]
          n1058 = Increment(x=w2763) -> (x+1=w2764:i32)
        }
        frame 315 {
          n1059 = call "Verify Timer.vi"("error in (no error)"=w2775, "State Machine in"=w2773) -> ("error out"=w2774:errorcluster, "timeout"=w2770:bool, "State Machine out"=w2777:refnum<class "State Machine.lvclass">)  [unwired: 7 in]
          n1060 = call-dynamic "Write State Machine.vi"("error in (no error)"=w2774, "State Machine.lvclass"=w2777, "Device in"=w2776) -> ("error out"=w2771:errorcluster, "Device out"=w2772:refnum<class "Channel.lvclass">)  [unwired: 7 in]
          n1061 = call-dynamic "Read resp.vi"("error in (no error)"=w2771, "Device in"=w2772) -> ("error out"=w2778:errorcluster, "resp"=w2781:string, "Device out"=w2779:refnum<class "Channel.lvclass">)  [unwired: 7 in]
          n1062 = Equal?(x=w2781, y="DONE") -> (x = y?=w2768:bool)
          n1063 = case shown="False" w2770 {
            tunnel: [w2783 0] -> w2767
            tunnel: w2769 -> [w2784 _]
            tunnel: w2768 -> [w2782 _]
            frame False {
              n1064 = case shown="True" w2782 {
                tunnel: w2784 -> [w2785 w2787]
                tunnel: [w2785 w2786] -> w2783
                frame False {
                }
                frame True {
                  n1065 = Increment(x=w2787) -> (x+1=w2786:i32)
                }
              }
            }
            frame True {
            }
          }
        }
        frame 316 {
          # "Carrega timeout de 50 ciclos\npara resposta do ACS"
          n1066 = call-dynamic "Write Timer.vi"("error in (no error)"=w2797, "Timer"=u32 50, "State Machine in"=w2796) -> ("error out"=w2799:errorcluster, "State Machine out"=w2801:refnum<class "State Machine.lvclass">)  [unwired: 7 in]
          n1067 = call-dynamic "Write State Machine.vi"("error in (no error)"=w2799, "State Machine.lvclass"=w2801, "Device in"=w2798) -> ("error out"=w2791:errorcluster, "Device out"=w2790:refnum<class "Channel.lvclass">)  [unwired: 7 in]
          n1068 = Unbundle By Name(w2790) -> ("rotator"=w2789:dbl)
          n1069 = Number To Fractional String(number=w2789) -> (F-format string=w2793:string)  [unwired: 3 in]
          n1070 = Concatenate Strings("SET INSTROT " ("cmd"), w2793) -> (w2792:string)
          n1071 = call-dynamic "Write cmd.vi"("error in (no error)"=w2791, "cmd"=w2792, "Device in"=w2790) -> ("error out"=w2803:errorcluster, "Device out"=w2804:refnum<class "Channel.lvclass">)  [unwired: 7 in]
          n1072 = Increment(x=w2795) -> (x+1=w2802:i32)
        }
        frame 317 {
          n1073 = call "Verify Timer.vi"("error in (no error)"=w2809, "State Machine in"=w2810) -> ("error out"=w2814:errorcluster, "timeout"=w2806:bool, "State Machine out"=w2815:refnum<class "State Machine.lvclass">)  [unwired: 7 in]
          n1074 = call-dynamic "Write State Machine.vi"("error in (no error)"=w2814, "State Machine.lvclass"=w2815, "Device in"=w2813) -> ("error out"=w2811:errorcluster, "Device out"=w2812:refnum<class "Channel.lvclass">)  [unwired: 7 in]
          n1075 = call-dynamic "Read resp.vi"("error in (no error)"=w2811, "Device in"=w2812) -> ("error out"=w2816:errorcluster, "resp"=w2819:string, "Device out"=w2817:refnum<class "Channel.lvclass">)  [unwired: 7 in]
          n1076 = Equal?(x=w2819, y="DONE") -> (x = y?=w2805:bool)
          n1077 = case shown="False" w2806 {
            tunnel: [w2821 0] -> w2808
            tunnel: w2807 -> [w2822 _]
            tunnel: w2805 -> [w2820 _]
            frame False {
              n1078 = case shown="True" w2820 {
                tunnel: [w2823 w2824] -> w2821
                tunnel: w2822 -> [w2823 w2825]
                frame False {
                }
                frame True {
                  n1079 = Increment(x=w2825) -> (x+1=w2824:i32)
                }
              }
            }
            frame True {
            }
          }
        }
        frame 318 {
          # "Carrega timeout de 50 ciclos\npara resposta do ACS"
          n1080 = call-dynamic "Write Timer.vi"("error in (no error)"=w2834, "Timer"=u32 50, "State Machine in"=w2833) -> ("error out"=w2836:errorcluster, "State Machine out"=w2838:refnum<class "State Machine.lvclass">)  [unwired: 7 in]
          n1081 = call-dynamic "Write State Machine.vi"("error in (no error)"=w2836, "State Machine.lvclass"=w2838, "Device in"=w2835) -> ("error out"=w2829:errorcluster, "Device out"=w2828:refnum<class "Channel.lvclass">)  [unwired: 7 in]
          n1082 = Unbundle By Name(w2828) -> ("TCS mode"=w2827:string)
          n1083 = Concatenate Strings("SET TCSMODE " ("cmd"), w2827) -> (w2830:string)
          n1084 = call-dynamic "Write cmd.vi"("error in (no error)"=w2829, "cmd"=w2830, "Device in"=w2828) -> ("error out"=w2840:errorcluster, "Device out"=w2841:refnum<class "Channel.lvclass">)  [unwired: 7 in]
          n1085 = Increment(x=w2832) -> (x+1=w2839:i32)
        }
        frame 319 {
          n1086 = call "Verify Timer.vi"("error in (no error)"=w2846, "State Machine in"=w2847) -> ("error out"=w2851:errorcluster, "timeout"=w2843:bool, "State Machine out"=w2852:refnum<class "State Machine.lvclass">)  [unwired: 7 in]
          n1087 = call-dynamic "Write State Machine.vi"("error in (no error)"=w2851, "State Machine.lvclass"=w2852, "Device in"=w2850) -> ("error out"=w2848:errorcluster, "Device out"=w2849:refnum<class "Channel.lvclass">)  [unwired: 7 in]
          n1088 = call-dynamic "Read resp.vi"("error in (no error)"=w2848, "Device in"=w2849) -> ("error out"=w2853:errorcluster, "resp"=w2856:string, "Device out"=w2854:refnum<class "Channel.lvclass">)  [unwired: 7 in]
          n1089 = Equal?(x=w2856, y="DONE") -> (x = y?=w2842:bool)
          n1090 = case shown="False" w2843 {
            tunnel: [w2858 0] -> w2845
            tunnel: w2844 -> [w2859 _]
            tunnel: w2842 -> [w2857 _]
            frame False {
              n1091 = case shown="True" w2857 {
                tunnel: [w2860 w2861] -> w2858
                tunnel: w2859 -> [w2860 w2862]
                frame False {
                }
                frame True {
                  n1092 = Increment(x=w2862) -> (x+1=w2861:i32)
                }
              }
            }
            frame True {
            }
          }
        }
        frame 320 {
          # "Carrega timeout de 50 ciclos\npara resposta do ACS"
          n1093 = call-dynamic "Write Timer.vi"("error in (no error)"=w2871, "Timer"=u32 50, "State Machine in"=w2870) -> ("error out"=w2873:errorcluster, "State Machine out"=w2875:refnum<class "State Machine.lvclass">)  [unwired: 7 in]
          n1094 = call-dynamic "Write State Machine.vi"("error in (no error)"=w2873, "State Machine.lvclass"=w2875, "Device in"=w2872) -> ("error out"=w2866:errorcluster, "Device out"=w2865:refnum<class "Channel.lvclass">)  [unwired: 7 in]
          n1095 = Unbundle By Name(w2865) -> ("ICS mode"=w2864:string)
          n1096 = Concatenate Strings("SET ICSMODE " ("cmd"), w2864) -> (w2867:string)
          n1097 = call-dynamic "Write cmd.vi"("error in (no error)"=w2866, "cmd"=w2867, "Device in"=w2865) -> ("error out"=w2877:errorcluster, "Device out"=w2878:refnum<class "Channel.lvclass">)  [unwired: 7 in]
          n1098 = Increment(x=w2869) -> (x+1=w2876:i32)
        }
        frame 321 {
          n1099 = call "Verify Timer.vi"("error in (no error)"=w2883, "State Machine in"=w2884) -> ("error out"=w2888:errorcluster, "timeout"=w2882:bool, "State Machine out"=w2889:refnum<class "State Machine.lvclass">)  [unwired: 7 in]
          n1100 = call-dynamic "Write State Machine.vi"("error in (no error)"=w2888, "State Machine.lvclass"=w2889, "Device in"=w2887) -> ("error out"=w2885:errorcluster, "Device out"=w2886:refnum<class "Channel.lvclass">)  [unwired: 7 in]
          n1101 = call-dynamic "Read resp.vi"("error in (no error)"=w2885, "Device in"=w2886) -> ("error out"=w2890:errorcluster, "resp"=w2893:string, "Device out"=w2891:refnum<class "Channel.lvclass">)  [unwired: 7 in]
          n1102 = Equal?(x=w2893, y="DONE") -> (x = y?=w2880:bool)
          n1103 = case shown="False" w2882 {
            tunnel: [w2895 w2901] -> w2879
            tunnel: w2881 -> [w2896 _]
            tunnel: w2880 -> [w2894 _]
            frame False {
              n1104 = case shown="True" w2894 {
                tunnel: [w2897 w2898] -> w2895
                tunnel: w2896 -> [w2897 _]
                frame False {
                }
                frame True {
                  n1105 = disable-structure shown="Enabled" {
                    disable-tunnel: [0 ("State") 40] -> w2898
                    frame Disabled {
                    }
                    frame Enabled {
                      # "Configura\nExpMode"
                    }
                  }
                }
              }
            }
            frame True {
              n1106 = disable-structure shown="Enabled" {
                disable-tunnel: [0 40] -> w2901
                frame Enabled {
                }
                frame Disabled {
                  # "Configura\nExpMode"
                }
              }
            }
          }
        }
      }
      n1107 = call-dynamic "Read State Machine.vi"("error in (no error)"=w7, "Device in"=w14) -> ("error out"=w10:errorcluster, "State Machine.lvclass"=w13:refnum<class "State Machine.lvclass">, "Device out"=w12:refnum<class "Channel.lvclass">)  [unwired: 7 in]
      n1108 = call "Next State.vi"("error in (no error)"=w10, "New_State"=w8, "State Machine in"=w13) -> ("error out"=w9:errorcluster, "State Machine out"=w15:refnum<class "State Machine.lvclass">)  [unwired: 7 in]
      n1109 = call-dynamic "Write State Machine.vi"("error in (no error)"=w9, "State Machine.lvclass"=w15, "Device in"=w12) -> ("error out"=w6:errorcluster, "Device out"=w11:refnum<class "Channel.lvclass">)  [unwired: 7 in]
    }
    frame Error {
    }
  }
  "error out" <- w3
  "Channel out" <- w1
